vi "LabView Text Okuma.vi"() -> ()   [LabVIEW 2017]
uses:
  <vilib>/Math Plots/3D Math Plots/3D Bar/3D Bar XCtrl/3D Bar.xctl
  <vilib>/Utility/file.llb/Read Delimited Spreadsheet (DBL).vi
  <vilib>/Math Plots/3D Math Plots/3D Bar/3D Bar Datatype/Public/Plot Helper (Matrix).vi
  <vilib>/Math Plots/3D Math Plots/3D Bar/3D Bar Datatype/3D Bar Datatype.lvclass
panel:
  in  "stop 2":bool
  in  "stop":bool
  in  "Gerilme Türünü Seçiniz":string(combo)
  in  "Parça Seçiniz":string(combo)
  in  "Grafik Türünü Seçiniz":string(combo)
  out "?":refnum<class "3D Plot Datatype.lvclass">[](xcontrol)
  out "Array 3":dbl[][](array[numeric])
  out "Min. Yer Değiştirme(mm)":dbl
  out "Max. Yer Değiştirme(mm)":dbl
  out "Max.VonMises Gerilmesi(MPA)":dbl
  out "Min. VonMises Gerilmesi (MPA)":dbl
  in  "Gerilme Türünü Seçiniz":string(combo)
  in  "Ugulanacak Kuvvet Seçiniz (N)":string(combo)
  in  "Parça Seçiniz":string(combo)
  out "Sonuçlar":dbl[][](array[numeric])
  in  "Çıkış":bool
  in  "Oku":bool
  in  "Analiz Yapmak İstedeğiniz Parçanın Veri Dosyasını Açınız!":path
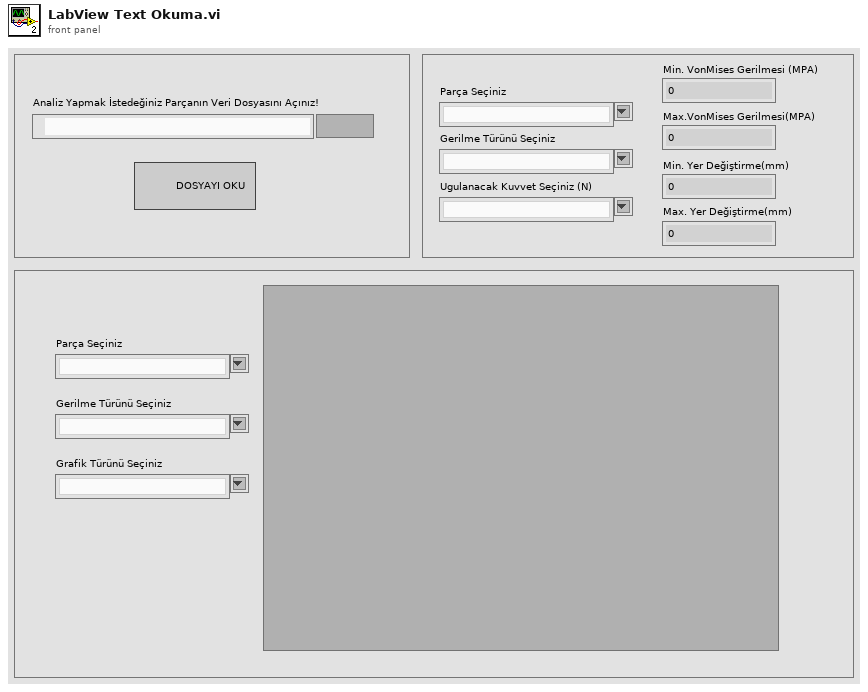
[diagram p1: front panel]
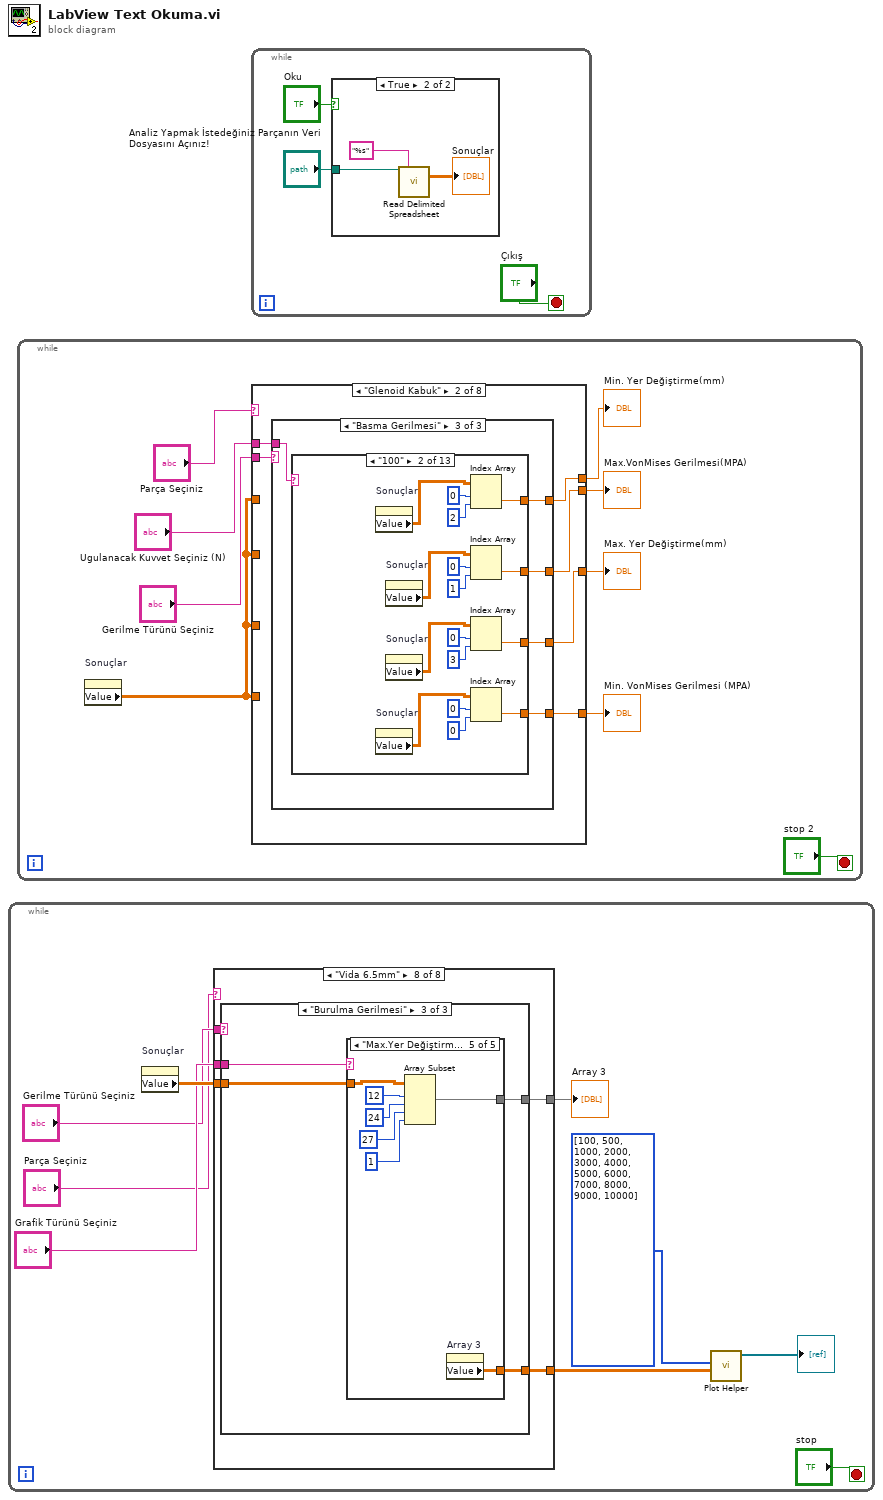
[diagram p0: block diagram]
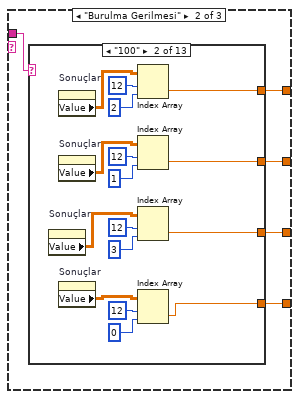
[diagram p4: hidden frame]
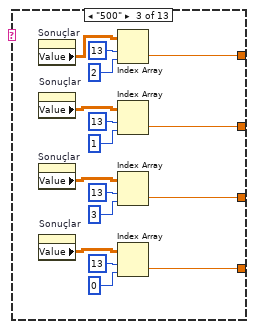
[diagram p6: hidden frame]
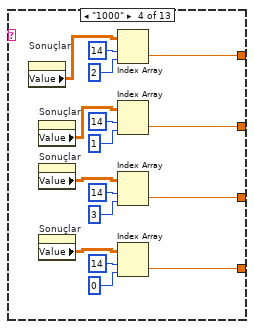
[diagram p7: hidden frame]
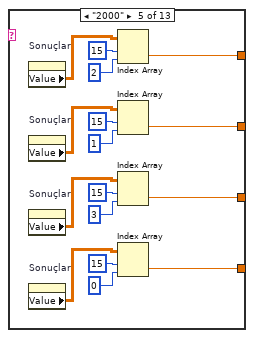
[diagram p8: hidden frame]
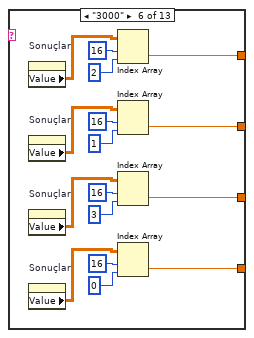
[diagram p9: hidden frame]
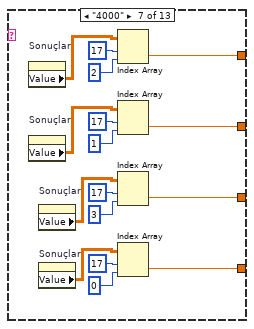
[diagram p10: hidden frame]
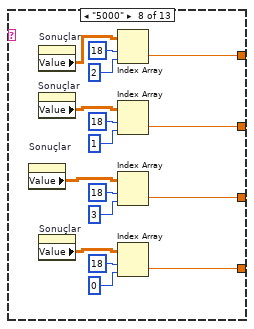
[diagram p11: hidden frame]
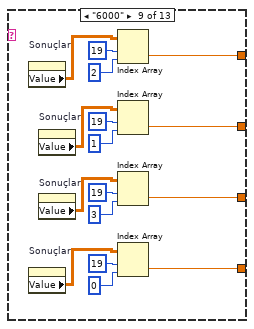
[diagram p12: hidden frame]
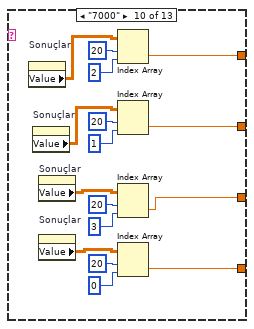
[diagram p13: hidden frame]
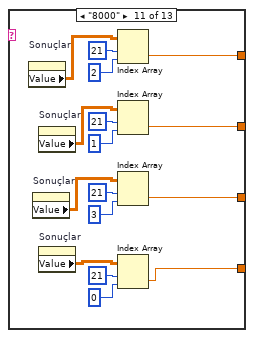
[diagram p14: hidden frame]
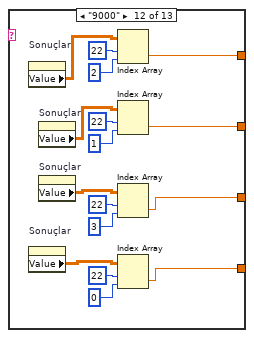
[diagram p15: hidden frame]
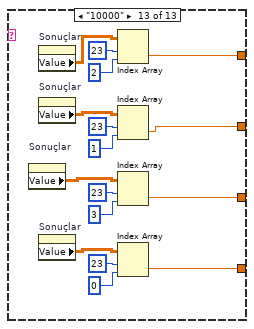
[diagram p16: hidden frame]
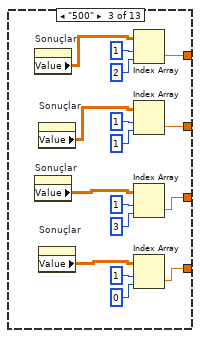
[diagram p18: hidden frame]
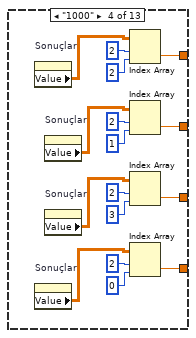
[diagram p19: hidden frame]
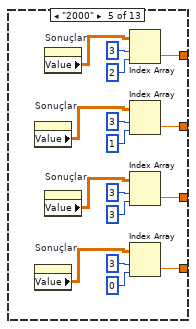
[diagram p20: hidden frame]
diagram:
  n1 = while {
    stop <- "stop" stop-if-true
    n2 = property on="Sonuçlar" class="Arr (strict)"() -> ("Value"=w8:dbl[][])  [unwired: 2 in, 2 out]
    n3 = case shown="\"Vida 6.5mm\"" "Parça Seçiniz" {
      tunnel: w8 -> [_ w14 w83 w152 w220 w290 w359 w428]
      tunnel: "Grafik Türünü Seçiniz" -> [_ w13 w80 w149 w218 w287 w356 w426]
      tunnel: [_ w10 w82 w151 w219 w289 w358 w427] -> w2
      tunnel: [_ w11 w81 w150 w221 w288 w357 w424] -> w6
      tunnel: "Gerilme Türünü Seçiniz" -> [_ w12 w79 w148 w217 w286 w355 w425]
      frame "False", Default {
      }
      frame "Glenoid Kabuk" {
        n4 = case shown="\"Burulma Gerilmesi\"" w12 {
          tunnel: w14 -> [_ w17 w49]
          tunnel: [_ w15 w48] -> w10
          tunnel: [_ w18 w47] -> w11
          tunnel: w13 -> [_ w16 w50]
          frame "False", Default {
          }
          frame "Basma Gerilmesi" {
            n5 = case shown="\"Max.Yer Değiştirme\"" w16 {
              tunnel: w17 -> [_ w20 w28 w35 w43]
              tunnel: [_ w21 w27 w36 w42] -> w15
              tunnel: [_ w19 w26 w33 w40] -> w18
              frame "False", Default {
              }
              frame "Min.VonMises" {
                n6 = Array Subset(array=w20, index (row)=0 ("index"), length (row)=12 ("length"), index (col)=0 ("index"), length (col)=1 ("length")) -> (w21:dbl[][])
                n7 = property on="Array 3" class="Arr (strict)"() -> ("Value"=w19:dbl[][])  [unwired: 2 in, 2 out]
              }
              frame "Max.VonMises" {
                n8 = Array Subset(array=w28, index (row)=0 ("index"), length (row)=12 ("length"), index (col)=1 ("index"), length (col)=1 ("length")) -> (w27:dbl[][])
                n9 = property on="Array 3" class="Arr (strict)"() -> ("Value"=w26:dbl[][])  [unwired: 2 in, 2 out]
              }
              frame "Min.Yer Değiştirme" {
                n10 = Array Subset(array=w35, index (row)=0 ("index"), length (row)=12 ("length"), index (col)=2 ("index"), length (col)=1 ("length")) -> (w36:dbl[][])
                n11 = property on="Array 3" class="Arr (strict)"() -> ("Value"=w33:dbl[][])  [unwired: 2 in, 2 out]
              }
              frame "Max.Yer Değiştirme" {
                n12 = Array Subset(array=w43, index (row)=0 ("index"), length (row)=12 ("length"), index (col)=3 ("index"), length (col)=1 ("length")) -> (w42:dbl[][])
                n13 = property on="Array 3" class="Arr (strict)"() -> ("Value"=w40:dbl[][])  [unwired: 2 in, 2 out]
              }
            }
          }
          frame "Burulma Gerilmesi" {
            n14 = case shown="\"Max.Yer Değiştirme\"" w50 {
              tunnel: w49 -> [_ w57 w60 w67 w75]
              tunnel: [_ w52 w59 w68 w74] -> w48
              tunnel: [_ w51 w58 w65 w72] -> w47
              frame "False", Default {
              }
              frame "Min.VonMises" {
                n15 = Array Subset(array=w57, index (row)=12 ("index"), length (row)=24 ("length"), index (col)=0 ("index"), length (col)=1 ("length")) -> (w52:dbl[][])
                n16 = property on="Array 3" class="Arr (strict)"() -> ("Value"=w51:dbl[][])  [unwired: 2 in, 2 out]
              }
              frame "Max.VonMises" {
                n17 = Array Subset(array=w60, index (row)=12 ("index"), length (row)=24 ("length"), index (col)=1 ("index"), length (col)=1 ("length")) -> (w59:dbl[][])
                n18 = property on="Array 3" class="Arr (strict)"() -> ("Value"=w58:dbl[][])  [unwired: 2 in, 2 out]
              }
              frame "Min.Yer Değiştirme" {
                n19 = Array Subset(array=w67, index (row)=12 ("index"), length (row)=24 ("length"), index (col)=2 ("index"), length (col)=1 ("length")) -> (w68:dbl[][])
                n20 = property on="Array 3" class="Arr (strict)"() -> ("Value"=w65:dbl[][])  [unwired: 2 in, 2 out]
              }
              frame "Max.Yer Değiştirme" {
                n21 = Array Subset(array=w75, index (row)=12 ("index"), length (row)=24 ("length"), index (col)=3 ("index"), length (col)=1 ("length")) -> (w74:dbl[][])
                n22 = property on="Array 3" class="Arr (strict)"() -> ("Value"=w72:dbl[][])  [unwired: 2 in, 2 out]
              }
            }
          }
        }
      }
      frame "Glenoid Yuva" {
        n23 = case shown="\"Burulma Gerilmesi\"" w79 {
          tunnel: w83 -> [_ w86 w118]
          tunnel: [_ w85 w117] -> w82
          tunnel: [_ w87 w116] -> w81
          tunnel: w80 -> [_ w84 w119]
          frame "False", Default {
          }
          frame "Basma Gerilmesi" {
            n24 = case shown="\"Max.Yer Değiştirme\"" w84 {
              tunnel: w86 -> [_ w89 w97 w104 w112]
              tunnel: [_ w90 w96 w105 w111] -> w85
              tunnel: [_ w88 w95 w102 w109] -> w87
              frame "False", Default {
              }
              frame "Min.VonMises" {
                n25 = Array Subset(array=w89, index (row)=0 ("index"), length (row)=12 ("length"), index (col)=4 ("index"), length (col)=1 ("length")) -> (w90:dbl[][])
                n26 = property on="Array 3" class="Arr (strict)"() -> ("Value"=w88:dbl[][])  [unwired: 2 in, 2 out]
              }
              frame "Max.VonMises" {
                n27 = Array Subset(array=w97, index (row)=0 ("index"), length (row)=12 ("length"), index (col)=5 ("index"), length (col)=1 ("length")) -> (w96:dbl[][])
                n28 = property on="Array 3" class="Arr (strict)"() -> ("Value"=w95:dbl[][])  [unwired: 2 in, 2 out]
              }
              frame "Min.Yer Değiştirme" {
                n29 = Array Subset(array=w104, index (row)=0 ("index"), length (row)=12 ("length"), index (col)=6 ("index"), length (col)=1 ("length")) -> (w105:dbl[][])
                n30 = property on="Array 3" class="Arr (strict)"() -> ("Value"=w102:dbl[][])  [unwired: 2 in, 2 out]
              }
              frame "Max.Yer Değiştirme" {
                n31 = Array Subset(array=w112, index (row)=0 ("index"), length (row)=12 ("length"), index (col)=7 ("index"), length (col)=1 ("length")) -> (w111:dbl[][])
                n32 = property on="Array 3" class="Arr (strict)"() -> ("Value"=w109:dbl[][])  [unwired: 2 in, 2 out]
              }
            }
          }
          frame "Burulma Gerilmesi" {
            n33 = case shown="\"Max.Yer Değiştirme\"" w119 {
              tunnel: w118 -> [_ w126 w129 w136 w144]
              tunnel: [_ w121 w128 w137 w143] -> w117
              tunnel: [_ w120 w127 w134 w141] -> w116
              frame "False", Default {
              }
              frame "Min.VonMises" {
                n34 = Array Subset(array=w126, index (row)=12 ("index"), length (row)=24 ("length"), index (col)=4 ("index"), length (col)=1 ("length")) -> (w121:dbl[][])
                n35 = property on="Array 3" class="Arr (strict)"() -> ("Value"=w120:dbl[][])  [unwired: 2 in, 2 out]
              }
              frame "Max.VonMises" {
                n36 = Array Subset(array=w129, index (row)=12 ("index"), length (row)=24 ("length"), index (col)=5 ("index"), length (col)=1 ("length")) -> (w128:dbl[][])
                n37 = property on="Array 3" class="Arr (strict)"() -> ("Value"=w127:dbl[][])  [unwired: 2 in, 2 out]
              }
              frame "Min.Yer Değiştirme" {
                n38 = Array Subset(array=w136, index (row)=12 ("index"), length (row)=24 ("length"), index (col)=6 ("index"), length (col)=1 ("length")) -> (w137:dbl[][])
                n39 = property on="Array 3" class="Arr (strict)"() -> ("Value"=w134:dbl[][])  [unwired: 2 in, 2 out]
              }
              frame "Max.Yer Değiştirme" {
                n40 = Array Subset(array=w144, index (row)=12 ("index"), length (row)=24 ("length"), index (col)=7 ("index"), length (col)=1 ("length")) -> (w143:dbl[][])
                n41 = property on="Array 3" class="Arr (strict)"() -> ("Value"=w141:dbl[][])  [unwired: 2 in, 2 out]
              }
            }
          }
        }
      }
      frame "BüyükKafa" {
        n42 = case shown="\"Burulma Gerilmesi\"" w148 {
          tunnel: w152 -> [_ w155 w187]
          tunnel: [_ w154 w186] -> w151
          tunnel: [_ w156 w185] -> w150
          tunnel: w149 -> [_ w153 w188]
          frame "False", Default {
          }
          frame "Basma Gerilmesi" {
            n43 = case shown="\"Min.VonMises\"" w153 {
              tunnel: w155 -> [_ w158 w166 w173 w181]
              tunnel: [_ w159 w165 w174 w180] -> w154
              tunnel: [_ w157 w164 w171 w178] -> w156
              frame "False", Default {
              }
              frame "Min.VonMises" {
                n44 = Array Subset(array=w158, index (row)=0 ("index"), length (row)=12 ("length"), index (col)=8 ("index"), length (col)=1 ("length")) -> (w159:dbl[][])
                n45 = property on="Array 3" class="Arr (strict)"() -> ("Value"=w157:dbl[][])  [unwired: 2 in, 2 out]
              }
              frame "Max.VonMises" {
                n46 = Array Subset(array=w166, index (row)=0 ("index"), length (row)=12 ("length"), index (col)=9 ("index"), length (col)=1 ("length")) -> (w165:dbl[][])
                n47 = property on="Array 3" class="Arr (strict)"() -> ("Value"=w164:dbl[][])  [unwired: 2 in, 2 out]
              }
              frame "Min.Yer Değiştirme" {
                n48 = Array Subset(array=w173, index (row)=0 ("index"), length (row)=12 ("length"), index (col)=10 ("index"), length (col)=1 ("length")) -> (w174:dbl[][])
                n49 = property on="Array 3" class="Arr (strict)"() -> ("Value"=w171:dbl[][])  [unwired: 2 in, 2 out]
              }
              frame "Max.Yer Değiştirme" {
                n50 = Array Subset(array=w181, index (row)=0 ("index"), length (row)=12 ("length"), index (col)=11 ("index"), length (col)=1 ("length")) -> (w180:dbl[][])
                n51 = property on="Array 3" class="Arr (strict)"() -> ("Value"=w178:dbl[][])  [unwired: 2 in, 2 out]
              }
            }
          }
          frame "Burulma Gerilmesi" {
            n52 = case shown="\"Max.Yer Değiştirme\"" w188 {
              tunnel: w187 -> [_ w195 w198 w205 w213]
              tunnel: [_ w190 w197 w206 w212] -> w186
              tunnel: [_ w189 w196 w203 w210] -> w185
              frame "False", Default {
              }
              frame "Min.VonMises" {
                n53 = Array Subset(array=w195, index (row)=12 ("index"), length (row)=24 ("length"), index (col)=8 ("index"), length (col)=1 ("length")) -> (w190:dbl[][])
                n54 = property on="Array 3" class="Arr (strict)"() -> ("Value"=w189:dbl[][])  [unwired: 2 in, 2 out]
              }
              frame "Max.VonMises" {
                n55 = Array Subset(array=w198, index (row)=12 ("index"), length (row)=24 ("length"), index (col)=9 ("index"), length (col)=1 ("length")) -> (w197:dbl[][])
                n56 = property on="Array 3" class="Arr (strict)"() -> ("Value"=w196:dbl[][])  [unwired: 2 in, 2 out]
              }
              frame "Min.Yer Değiştirme" {
                n57 = Array Subset(array=w205, index (row)=12 ("index"), length (row)=24 ("length"), index (col)=10 ("index"), length (col)=1 ("length")) -> (w206:dbl[][])
                n58 = property on="Array 3" class="Arr (strict)"() -> ("Value"=w203:dbl[][])  [unwired: 2 in, 2 out]
              }
              frame "Max.Yer Değiştirme" {
                n59 = Array Subset(array=w213, index (row)=12 ("index"), length (row)=24 ("length"), index (col)=11 ("index"), length (col)=1 ("length")) -> (w212:dbl[][])
                n60 = property on="Array 3" class="Arr (strict)"() -> ("Value"=w210:dbl[][])  [unwired: 2 in, 2 out]
              }
            }
          }
        }
      }
      frame "KüçükKafa" {
        n61 = case shown="\"Burulma Gerilmesi\"" w217 {
          tunnel: w220 -> [_ w224 w256]
          tunnel: [_ w223 w255] -> w219
          tunnel: [_ w225 w254] -> w221
          tunnel: w218 -> [_ w222 w257]
          frame "False", Default {
          }
          frame "Basma Gerilmesi" {
            n62 = case shown="\"Min.Yer Değiştirme\"" w222 {
              tunnel: w224 -> [_ w232 w235 w242 w250]
              tunnel: [_ w227 w234 w243 w249] -> w223
              tunnel: [_ w226 w233 w240 w247] -> w225
              frame "False", Default {
              }
              frame "Min.VonMises" {
                n63 = Array Subset(array=w232, index (row)=0 ("index"), length (row)=12 ("length"), index (col)=12 ("index"), length (col)=1 ("length")) -> (w227:dbl[][])
                n64 = property on="Array 3" class="Arr (strict)"() -> ("Value"=w226:dbl[][])  [unwired: 2 in, 2 out]
              }
              frame "Max.VonMises" {
                n65 = Array Subset(array=w235, index (row)=0 ("index"), length (row)=12 ("length"), index (col)=13 ("index"), length (col)=1 ("length")) -> (w234:dbl[][])
                n66 = property on="Array 3" class="Arr (strict)"() -> ("Value"=w233:dbl[][])  [unwired: 2 in, 2 out]
              }
              frame "Min.Yer Değiştirme" {
                n67 = Array Subset(array=w242, index (row)=0 ("index"), length (row)=12 ("length"), index (col)=14 ("index"), length (col)=1 ("length")) -> (w243:dbl[][])
                n68 = property on="Array 3" class="Arr (strict)"() -> ("Value"=w240:dbl[][])  [unwired: 2 in, 2 out]
              }
              frame "Max.Yer Değiştirme" {
                n69 = Array Subset(array=w250, index (row)=0 ("index"), length (row)=12 ("length"), index (col)=15 ("index"), length (col)=1 ("length")) -> (w249:dbl[][])
                n70 = property on="Array 3" class="Arr (strict)"() -> ("Value"=w247:dbl[][])  [unwired: 2 in, 2 out]
              }
            }
          }
          frame "Burulma Gerilmesi" {
            n71 = case shown="\"Max.Yer Değiştirme\"" w257 {
              tunnel: w256 -> [_ w264 w267 w274 w282]
              tunnel: [_ w259 w266 w275 w281] -> w255
              tunnel: [_ w258 w265 w272 w279] -> w254
              frame "False", Default {
              }
              frame "Min.VonMises" {
                n72 = Array Subset(array=w264, index (row)=12 ("index"), length (row)=24 ("length"), index (col)=12 ("index"), length (col)=1 ("length")) -> (w259:dbl[][])
                n73 = property on="Array 3" class="Arr (strict)"() -> ("Value"=w258:dbl[][])  [unwired: 2 in, 2 out]
              }
              frame "Max.VonMises" {
                n74 = Array Subset(array=w267, index (row)=12 ("index"), length (row)=24 ("length"), index (col)=13 ("index"), length (col)=1 ("length")) -> (w266:dbl[][])
                n75 = property on="Array 3" class="Arr (strict)"() -> ("Value"=w265:dbl[][])  [unwired: 2 in, 2 out]
              }
              frame "Min.Yer Değiştirme" {
                n76 = Array Subset(array=w274, index (row)=12 ("index"), length (row)=24 ("length"), index (col)=14 ("index"), length (col)=1 ("length")) -> (w275:dbl[][])
                n77 = property on="Array 3" class="Arr (strict)"() -> ("Value"=w272:dbl[][])  [unwired: 2 in, 2 out]
              }
              frame "Max.Yer Değiştirme" {
                n78 = Array Subset(array=w282, index (row)=12 ("index"), length (row)=24 ("length"), index (col)=15 ("index"), length (col)=1 ("length")) -> (w281:dbl[][])
                n79 = property on="Array 3" class="Arr (strict)"() -> ("Value"=w279:dbl[][])  [unwired: 2 in, 2 out]
              }
            }
          }
        }
      }
      frame "Humeral Sap" {
        n80 = case shown="\"Basma Gerilmesi\"" w286 {
          tunnel: w290 -> [_ w294 w325]
          tunnel: [_ w291 w324] -> w289
          tunnel: [_ w293 w323] -> w288
          tunnel: w287 -> [_ w292 w326]
          frame "False", Default {
          }
          frame "Basma Gerilmesi" {
            n81 = case shown="\"Max.Yer Değiştirme\"" w292 {
              tunnel: w294 -> [_ w301 w304 w311 w319]
              tunnel: [_ w296 w303 w312 w318] -> w291
              tunnel: [_ w295 w302 w310 w317] -> w293
              frame "False", Default {
              }
              frame "Min.VonMises" {
                n82 = Array Subset(array=w301, index (row)=0 ("index"), length (row)=12 ("length"), index (col)=16 ("index"), length (col)=1 ("length")) -> (w296:dbl[][])
                n83 = property on="Array 3" class="Arr (strict)"() -> ("Value"=w295:dbl[][])  [unwired: 2 in, 2 out]
              }
              frame "Max.VonMises" {
                n84 = Array Subset(array=w304, index (row)=0 ("index"), length (row)=12 ("length"), index (col)=17 ("index"), length (col)=1 ("length")) -> (w303:dbl[][])
                n85 = property on="Array 3" class="Arr (strict)"() -> ("Value"=w302:dbl[][])  [unwired: 2 in, 2 out]
              }
              frame "Min.Yer Değiştirme" {
                n86 = Array Subset(array=w311, index (row)=0 ("index"), length (row)=12 ("length"), index (col)=18 ("index"), length (col)=1 ("length")) -> (w312:dbl[][])
                n87 = property on="Array 3" class="Arr (strict)"() -> ("Value"=w310:dbl[][])  [unwired: 2 in, 2 out]
              }
              frame "Max.Yer Değiştirme" {
                n88 = Array Subset(array=w319, index (row)=0 ("index"), length (row)=12 ("length"), index (col)=19 ("index"), length (col)=1 ("length")) -> (w318:dbl[][])
                n89 = property on="Array 3" class="Arr (strict)"() -> ("Value"=w317:dbl[][])  [unwired: 2 in, 2 out]
              }
            }
          }
          frame "Burulma Gerilmesi" {
            n90 = case shown="\"Max.Yer Değiştirme\"" w326 {
              tunnel: w325 -> [_ w333 w336 w343 w351]
              tunnel: [_ w328 w335 w344 w350] -> w324
              tunnel: [_ w327 w334 w341 w348] -> w323
              frame "False", Default {
              }
              frame "Min.VonMises" {
                n91 = Array Subset(array=w333, index (row)=12 ("index"), length (row)=24 ("length"), index (col)=16 ("index"), length (col)=1 ("length")) -> (w328:dbl[][])
                n92 = property on="Array 3" class="Arr (strict)"() -> ("Value"=w327:dbl[][])  [unwired: 2 in, 2 out]
              }
              frame "Max.VonMises" {
                n93 = Array Subset(array=w336, index (row)=12 ("index"), length (row)=24 ("length"), index (col)=17 ("index"), length (col)=1 ("length")) -> (w335:dbl[][])
                n94 = property on="Array 3" class="Arr (strict)"() -> ("Value"=w334:dbl[][])  [unwired: 2 in, 2 out]
              }
              frame "Min.Yer Değiştirme" {
                n95 = Array Subset(array=w343, index (row)=12 ("index"), length (row)=24 ("length"), index (col)=18 ("index"), length (col)=1 ("length")) -> (w344:dbl[][])
                n96 = property on="Array 3" class="Arr (strict)"() -> ("Value"=w341:dbl[][])  [unwired: 2 in, 2 out]
              }
              frame "Max.Yer Değiştirme" {
                n97 = Array Subset(array=w351, index (row)=12 ("index"), length (row)=24 ("length"), index (col)=19 ("index"), length (col)=1 ("length")) -> (w350:dbl[][])
                n98 = property on="Array 3" class="Arr (strict)"() -> ("Value"=w348:dbl[][])  [unwired: 2 in, 2 out]
              }
            }
          }
        }
      }
      frame "Vida 4mm" {
        n99 = case shown="\"Burulma Gerilmesi\"" w355 {
          tunnel: w359 -> [_ w362 w394]
          tunnel: [_ w361 w393] -> w358
          tunnel: [_ w363 w392] -> w357
          tunnel: w356 -> [_ w360 w395]
          frame "False", Default {
          }
          frame "Basma Gerilmesi" {
            n100 = case shown="\"False\", Default" w360 {
              tunnel: w362 -> [_ w370 w373 w380 w388]
              tunnel: [_ w365 w372 w381 w387] -> w361
              tunnel: [_ w364 w371 w378 w385] -> w363
              frame "False", Default {
              }
              frame "Min.VonMises" {
                n101 = Array Subset(array=w370, index (row)=0 ("index"), length (row)=12 ("length"), index (col)=20 ("index"), length (col)=1 ("length")) -> (w365:dbl[][])
                n102 = property on="Array 3" class="Arr (strict)"() -> ("Value"=w364:dbl[][])  [unwired: 2 in, 2 out]
              }
              frame "Max.VonMises" {
                n103 = Array Subset(array=w373, index (row)=0 ("index"), length (row)=12 ("length"), index (col)=21 ("index"), length (col)=1 ("length")) -> (w372:dbl[][])
                n104 = property on="Array 3" class="Arr (strict)"() -> ("Value"=w371:dbl[][])  [unwired: 2 in, 2 out]
              }
              frame "Min.Yer Değiştirme" {
                n105 = Array Subset(array=w380, index (row)=0 ("index"), length (row)=12 ("length"), index (col)=22 ("index"), length (col)=1 ("length")) -> (w381:dbl[][])
                n106 = property on="Array 3" class="Arr (strict)"() -> ("Value"=w378:dbl[][])  [unwired: 2 in, 2 out]
              }
              frame "Max.Yer Değiştirme" {
                n107 = Array Subset(array=w388, index (row)=0 ("index"), length (row)=12 ("length"), index (col)=23 ("index"), length (col)=1 ("length")) -> (w387:dbl[][])
                n108 = property on="Array 3" class="Arr (strict)"() -> ("Value"=w385:dbl[][])  [unwired: 2 in, 2 out]
              }
            }
          }
          frame "Burulma Gerilmesi" {
            n109 = case shown="\"False\", Default" w395 {
              tunnel: w394 -> [_ w402 w405 w412 w420]
              tunnel: [_ w397 w404 w413 w419] -> w393
              tunnel: [_ w396 w403 w410 w417] -> w392
              frame "False", Default {
              }
              frame "Min.VonMises" {
                n110 = Array Subset(array=w402, index (row)=12 ("index"), length (row)=24 ("length"), index (col)=20 ("index"), length (col)=1 ("length")) -> (w397:dbl[][])
                n111 = property on="Array 3" class="Arr (strict)"() -> ("Value"=w396:dbl[][])  [unwired: 2 in, 2 out]
              }
              frame "Max.VonMises" {
                n112 = Array Subset(array=w405, index (row)=12 ("index"), length (row)=24 ("length"), index (col)=21 ("index"), length (col)=1 ("length")) -> (w404:dbl[][])
                n113 = property on="Array 3" class="Arr (strict)"() -> ("Value"=w403:dbl[][])  [unwired: 2 in, 2 out]
              }
              frame "Min.Yer Değiştirme" {
                n114 = Array Subset(array=w412, index (row)=12 ("index"), length (row)=24 ("length"), index (col)=22 ("index"), length (col)=1 ("length")) -> (w413:dbl[][])
                n115 = property on="Array 3" class="Arr (strict)"() -> ("Value"=w410:dbl[][])  [unwired: 2 in, 2 out]
              }
              frame "Max.Yer Değiştirme" {
                n116 = Array Subset(array=w420, index (row)=12 ("index"), length (row)=24 ("length"), index (col)=23 ("index"), length (col)=1 ("length")) -> (w419:dbl[][])
                n117 = property on="Array 3" class="Arr (strict)"() -> ("Value"=w417:dbl[][])  [unwired: 2 in, 2 out]
              }
            }
          }
        }
      }
      frame "Vida 6.5mm" {
        n118 = case shown="\"Burulma Gerilmesi\"" w425 {
          tunnel: w428 -> [_ w431 w463]
          tunnel: [_ w430 w462] -> w427
          tunnel: [_ w432 w461] -> w424
          tunnel: w426 -> [_ w429 w464]
          frame "False", Default {
          }
          frame "Basma Gerilmesi" {
            n119 = case shown="\"Min.VonMises\"" w429 {
              tunnel: w431 -> [_ w434 w442 w449 w457]
              tunnel: [_ w435 w441 w450 w456] -> w430
              tunnel: [_ w433 w440 w447 w454] -> w432
              frame "False", Default {
              }
              frame "Min.VonMises" {
                n120 = Array Subset(array=w434, index (row)=0 ("index"), length (row)=12 ("length"), index (col)=24 ("index"), length (col)=1 ("length")) -> (w435:dbl[][])
                n121 = property on="Array 3" class="Arr (strict)"() -> ("Value"=w433:dbl[][])  [unwired: 2 in, 2 out]
              }
              frame "Max.VonMises" {
                n122 = Array Subset(array=w442, index (row)=0 ("index"), length (row)=12 ("length"), index (col)=25 ("index"), length (col)=1 ("length")) -> (w441:dbl[][])
                n123 = property on="Array 3" class="Arr (strict)"() -> ("Value"=w440:dbl[][])  [unwired: 2 in, 2 out]
              }
              frame "Min.Yer Değiştirme" {
                n124 = Array Subset(array=w449, index (row)=0 ("index"), length (row)=12 ("length"), index (col)=26 ("index"), length (col)=1 ("length")) -> (w450:dbl[][])
                n125 = property on="Array 3" class="Arr (strict)"() -> ("Value"=w447:dbl[][])  [unwired: 2 in, 2 out]
              }
              frame "Max.Yer Değiştirme" {
                n126 = Array Subset(array=w457, index (row)=0 ("index"), length (row)=12 ("length"), index (col)=27 ("index"), length (col)=1 ("length")) -> (w456:dbl[][])
                n127 = property on="Array 3" class="Arr (strict)"() -> ("Value"=w454:dbl[][])  [unwired: 2 in, 2 out]
              }
            }
          }
          frame "Burulma Gerilmesi" {
            n128 = case shown="\"Max.Yer Değiştirme\"" w464 {
              tunnel: w463 -> [_ w471 w474 w481 w489]
              tunnel: [_ w466 w473 w482 w488] -> w462
              tunnel: [_ w465 w472 w479 w486] -> w461
              frame "False", Default {
              }
              frame "Min.VonMises" {
                n129 = Array Subset(array=w471, index (row)=12 ("index"), length (row)=24 ("length"), index (col)=24 ("index"), length (col)=1 ("length")) -> (w466:dbl[][])
                n130 = property on="Array 3" class="Arr (strict)"() -> ("Value"=w465:dbl[][])  [unwired: 2 in, 2 out]
              }
              frame "Max.VonMises" {
                n131 = Array Subset(array=w474, index (row)=12 ("index"), length (row)=24 ("length"), index (col)=24 ("index"), length (col)=1 ("length")) -> (w473:dbl[][])
                n132 = property on="Array 3" class="Arr (strict)"() -> ("Value"=w472:dbl[][])  [unwired: 2 in, 2 out]
              }
              frame "Min.Yer Değiştirme" {
                n133 = Array Subset(array=w481, index (row)=12 ("index"), length (row)=24 ("length"), index (col)=26 ("index"), length (col)=1 ("length")) -> (w482:dbl[][])
                n134 = property on="Array 3" class="Arr (strict)"() -> ("Value"=w479:dbl[][])  [unwired: 2 in, 2 out]
              }
              frame "Max.Yer Değiştirme" {
                n135 = Array Subset(array=w489, index (row)=12 ("index"), length (row)=24 ("length"), index (col)=27 ("index"), length (col)=1 ("length")) -> (w488:dbl[][])
                n136 = property on="Array 3" class="Arr (strict)"() -> ("Value"=w486:dbl[][])  [unwired: 2 in, 2 out]
              }
            }
          }
        }
      }
    }
    "Array 3" <- w2
    n137 = call-poly <vilib>:"Plot Helper.vi"("z matrix"=w6, "y vector"=i32[] [100, 500, 1000, 2000, 3000, 4000, 5000, 6000, 7000, 8000, 9000, 10000]) -> ("3D Plot lvclass Array out"=→"?":refnum<class "3D Plot Datatype.lvclass">[])  [unwired: 1 in, 8 out]
  }
  n138 = while {
    stop <- "stop 2" stop-if-true
    n139 = property on="Sonuçlar" class="Arr (strict)"() -> ("Value"=w494:dbl[][])  [unwired: 2 in, 2 out]
    n140 = case shown="\"Glenoid Kabuk\"" "Parça Seçiniz" {
      tunnel: "Gerilme Türünü Seçiniz" -> [_ w506 w906 w1306 w1706 w2111 w2522 w2934]
      tunnel: "Ugulanacak Kuvvet Seçiniz (N)" -> [_ w507 w907 w1307 w1707 w2110 w2523 w2935]
      tunnel: [_ w505 w903 w1304 w1705 w2103 w2514 w2926] -> w498
      tunnel: [_ w504 w904 w1303 w1703 w2106 w2516 w2928] -> w497
      tunnel: [_ w503 w905 w1302 w1702 w2108 w2517 w2929] -> w495
      tunnel: [_ w502 w902 w1305 w1704 w2102 w2515 w2927] -> w496
      tunnel: w494 -> [_ _ _ _ _ w2109 w2519 w2931]
      tunnel: w494 -> [_ _ _ _ _ w2107 w2521 w2933]
      tunnel: w494 -> [_ _ _ _ _ w2105 w2520 w2932]
      tunnel: w494 -> [_ _ _ _ _ w2104 w2518 w2930]
      frame "False", Default {
      }
      frame "Glenoid Kabuk" {
        n141 = case shown="\"Basma Gerilmesi\"" w506 {
          tunnel: w507 -> [_ w512 w709]
          tunnel: [_ w509 w708] -> w505
          tunnel: [_ w511 w707] -> w504
          tunnel: [_ w510 w706] -> w503
          tunnel: [_ w508 w705] -> w502
          frame "False", Default {
          }
          frame "Burulma Gerilmesi" {
            n142 = case shown="\"100\"" w512 {
              tunnel: [_ w514 w531 w546 w563 w579 w595 w612 w627 w642 w659 w674 w691] -> w511
              tunnel: [_ w513 w532 w545 w564 w580 w596 w611 w628 w641 w660 w673 w692] -> w510
              tunnel: [_ w515 w530 w547 w562 w578 w594 w610 w626 w643 w658 w675 w690] -> w509
              tunnel: [_ w516 w529 w548 w561 w577 w593 w609 w625 w644 w657 w676 w689] -> w508
              frame "False", Default {
              }
              frame "100" {
                n143 = property on="Sonuçlar" class="Arr (strict)"() -> ("Value"=w521:dbl[][])  [unwired: 2 in, 2 out]
                n144 = property on="Sonuçlar" class="Arr (strict)"() -> ("Value"=w524:dbl[][])  [unwired: 2 in, 2 out]
                n145 = property on="Sonuçlar" class="Arr (strict)"() -> ("Value"=w523:dbl[][])  [unwired: 2 in, 2 out]
                n146 = property on="Sonuçlar" class="Arr (strict)"() -> ("Value"=w522:dbl[][])  [unwired: 2 in, 2 out]
                n147 = Index Array(array=w524, index (row)=12 ("index"), index (col)=2 ("disabled index (col)")) -> (element=w513:dbl)
                n148 = Index Array(array=w523, index (row)=12 ("index"), index (col)=1 ("disabled index (col)")) -> (element=w514:dbl)
                n149 = Index Array(array=w521, index (row)=12 ("index"), index (col)=3 ("disabled index (col)")) -> (element=w516:dbl)
                n150 = Index Array(array=w522, index (row)=12 ("index"), index (col)=0 ("disabled index (col)")) -> (element=w515:dbl)
              }
              frame "500" {
                n151 = property on="Sonuçlar" class="Arr (strict)"() -> ("Value"=w534:dbl[][])  [unwired: 2 in, 2 out]
                n152 = property on="Sonuçlar" class="Arr (strict)"() -> ("Value"=w536:dbl[][])  [unwired: 2 in, 2 out]
                n153 = property on="Sonuçlar" class="Arr (strict)"() -> ("Value"=w540:dbl[][])  [unwired: 2 in, 2 out]
                n154 = property on="Sonuçlar" class="Arr (strict)"() -> ("Value"=w538:dbl[][])  [unwired: 2 in, 2 out]
                n155 = Index Array(array=w534, index (row)=13 ("index"), index (col)=2 ("disabled index (col)")) -> (element=w532:dbl)
                n156 = Index Array(array=w536, index (row)=13 ("index"), index (col)=1 ("disabled index (col)")) -> (element=w531:dbl)
                n157 = Index Array(array=w540, index (row)=13 ("index"), index (col)=3 ("disabled index (col)")) -> (element=w529:dbl)
                n158 = Index Array(array=w538, index (row)=13 ("index"), index (col)=0 ("disabled index (col)")) -> (element=w530:dbl)
              }
              frame "1000" {
                n159 = property on="Sonuçlar" class="Arr (strict)"() -> ("Value"=w556:dbl[][])  [unwired: 2 in, 2 out]
                n160 = property on="Sonuçlar" class="Arr (strict)"() -> ("Value"=w555:dbl[][])  [unwired: 2 in, 2 out]
                n161 = property on="Sonuçlar" class="Arr (strict)"() -> ("Value"=w553:dbl[][])  [unwired: 2 in, 2 out]
                n162 = property on="Sonuçlar" class="Arr (strict)"() -> ("Value"=w554:dbl[][])  [unwired: 2 in, 2 out]
                n163 = Index Array(array=w556, index (row)=14 ("index"), index (col)=2 ("disabled index (col)")) -> (element=w545:dbl)
                n164 = Index Array(array=w555, index (row)=14 ("index"), index (col)=1 ("disabled index (col)")) -> (element=w546:dbl)
                n165 = Index Array(array=w553, index (row)=14 ("index"), index (col)=3 ("disabled index (col)")) -> (element=w548:dbl)
                n166 = Index Array(array=w554, index (row)=14 ("index"), index (col)=0 ("disabled index (col)")) -> (element=w547:dbl)
              }
              frame "2000" {
                n167 = property on="Sonuçlar" class="Arr (strict)"() -> ("Value"=w572:dbl[][])  [unwired: 2 in, 2 out]
                n168 = property on="Sonuçlar" class="Arr (strict)"() -> ("Value"=w571:dbl[][])  [unwired: 2 in, 2 out]
                n169 = property on="Sonuçlar" class="Arr (strict)"() -> ("Value"=w569:dbl[][])  [unwired: 2 in, 2 out]
                n170 = property on="Sonuçlar" class="Arr (strict)"() -> ("Value"=w570:dbl[][])  [unwired: 2 in, 2 out]
                n171 = Index Array(array=w572, index (row)=15 ("index"), index (col)=2 ("disabled index (col)")) -> (element=w564:dbl)
                n172 = Index Array(array=w571, index (row)=15 ("index"), index (col)=1 ("disabled index (col)")) -> (element=w563:dbl)
                n173 = Index Array(array=w569, index (row)=15 ("index"), index (col)=3 ("disabled index (col)")) -> (element=w561:dbl)
                n174 = Index Array(array=w570, index (row)=15 ("index"), index (col)=0 ("disabled index (col)")) -> (element=w562:dbl)
              }
              frame "3000" {
                n175 = property on="Sonuçlar" class="Arr (strict)"() -> ("Value"=w582:dbl[][])  [unwired: 2 in, 2 out]
                n176 = property on="Sonuçlar" class="Arr (strict)"() -> ("Value"=w584:dbl[][])  [unwired: 2 in, 2 out]
                n177 = property on="Sonuçlar" class="Arr (strict)"() -> ("Value"=w588:dbl[][])  [unwired: 2 in, 2 out]
                n178 = property on="Sonuçlar" class="Arr (strict)"() -> ("Value"=w586:dbl[][])  [unwired: 2 in, 2 out]
                n179 = Index Array(array=w582, index (row)=16 ("index"), index (col)=2 ("disabled index (col)")) -> (element=w580:dbl)
                n180 = Index Array(array=w584, index (row)=16 ("index"), index (col)=1 ("disabled index (col)")) -> (element=w579:dbl)
                n181 = Index Array(array=w588, index (row)=16 ("index"), index (col)=3 ("disabled index (col)")) -> (element=w577:dbl)
                n182 = Index Array(array=w586, index (row)=16 ("index"), index (col)=0 ("disabled index (col)")) -> (element=w578:dbl)
              }
              frame "4000" {
                n183 = property on="Sonuçlar" class="Arr (strict)"() -> ("Value"=w601:dbl[][])  [unwired: 2 in, 2 out]
                n184 = property on="Sonuçlar" class="Arr (strict)"() -> ("Value"=w602:dbl[][])  [unwired: 2 in, 2 out]
                n185 = property on="Sonuçlar" class="Arr (strict)"() -> ("Value"=w604:dbl[][])  [unwired: 2 in, 2 out]
                n186 = property on="Sonuçlar" class="Arr (strict)"() -> ("Value"=w603:dbl[][])  [unwired: 2 in, 2 out]
                n187 = Index Array(array=w601, index (row)=17 ("index"), index (col)=2 ("disabled index (col)")) -> (element=w596:dbl)
                n188 = Index Array(array=w602, index (row)=17 ("index"), index (col)=1 ("disabled index (col)")) -> (element=w595:dbl)
                n189 = Index Array(array=w604, index (row)=17 ("index"), index (col)=3 ("disabled index (col)")) -> (element=w593:dbl)
                n190 = Index Array(array=w603, index (row)=17 ("index"), index (col)=0 ("disabled index (col)")) -> (element=w594:dbl)
              }
              frame "5000" {
                n191 = property on="Sonuçlar" class="Arr (strict)"() -> ("Value"=w617:dbl[][])  [unwired: 2 in, 2 out]
                n192 = property on="Sonuçlar" class="Arr (strict)"() -> ("Value"=w619:dbl[][])  [unwired: 2 in, 2 out]
                n193 = property on="Sonuçlar" class="Arr (strict)"() -> ("Value"=w620:dbl[][])  [unwired: 2 in, 2 out]
                n194 = property on="Sonuçlar" class="Arr (strict)"() -> ("Value"=w618:dbl[][])  [unwired: 2 in, 2 out]
                n195 = Index Array(array=w619, index (row)=18 ("index"), index (col)=2 ("disabled index (col)")) -> (element=w611:dbl)
                n196 = Index Array(array=w620, index (row)=18 ("index"), index (col)=1 ("disabled index (col)")) -> (element=w612:dbl)
                n197 = Index Array(array=w617, index (row)=18 ("index"), index (col)=3 ("disabled index (col)")) -> (element=w609:dbl)
                n198 = Index Array(array=w618, index (row)=18 ("index"), index (col)=0 ("disabled index (col)")) -> (element=w610:dbl)
              }
              frame "6000" {
                n199 = property on="Sonuçlar" class="Arr (strict)"() -> ("Value"=w633:dbl[][])  [unwired: 2 in, 2 out]
                n200 = property on="Sonuçlar" class="Arr (strict)"() -> ("Value"=w635:dbl[][])  [unwired: 2 in, 2 out]
                n201 = property on="Sonuçlar" class="Arr (strict)"() -> ("Value"=w634:dbl[][])  [unwired: 2 in, 2 out]
                n202 = property on="Sonuçlar" class="Arr (strict)"() -> ("Value"=w636:dbl[][])  [unwired: 2 in, 2 out]
                n203 = Index Array(array=w633, index (row)=19 ("index"), index (col)=2 ("disabled index (col)")) -> (element=w628:dbl)
                n204 = Index Array(array=w634, index (row)=19 ("index"), index (col)=1 ("disabled index (col)")) -> (element=w627:dbl)
                n205 = Index Array(array=w636, index (row)=19 ("index"), index (col)=3 ("disabled index (col)")) -> (element=w625:dbl)
                n206 = Index Array(array=w635, index (row)=19 ("index"), index (col)=0 ("disabled index (col)")) -> (element=w626:dbl)
              }
              frame "7000" {
                n207 = property on="Sonuçlar" class="Arr (strict)"() -> ("Value"=w649:dbl[][])  [unwired: 2 in, 2 out]
                n208 = property on="Sonuçlar" class="Arr (strict)"() -> ("Value"=w650:dbl[][])  [unwired: 2 in, 2 out]
                n209 = property on="Sonuçlar" class="Arr (strict)"() -> ("Value"=w652:dbl[][])  [unwired: 2 in, 2 out]
                n210 = property on="Sonuçlar" class="Arr (strict)"() -> ("Value"=w651:dbl[][])  [unwired: 2 in, 2 out]
                n211 = Index Array(array=w649, index (row)=20 ("index"), index (col)=2 ("disabled index (col)")) -> (element=w641:dbl)
                n212 = Index Array(array=w650, index (row)=20 ("index"), index (col)=1 ("disabled index (col)")) -> (element=w642:dbl)
                n213 = Index Array(array=w652, index (row)=20 ("index"), index (col)=3 ("disabled index (col)")) -> (element=w644:dbl)
                n214 = Index Array(array=w651, index (row)=20 ("index"), index (col)=0 ("disabled index (col)")) -> (element=w643:dbl)
              }
              frame "8000" {
                n215 = property on="Sonuçlar" class="Arr (strict)"() -> ("Value"=w665:dbl[][])  [unwired: 2 in, 2 out]
                n216 = property on="Sonuçlar" class="Arr (strict)"() -> ("Value"=w668:dbl[][])  [unwired: 2 in, 2 out]
                n217 = property on="Sonuçlar" class="Arr (strict)"() -> ("Value"=w666:dbl[][])  [unwired: 2 in, 2 out]
                n218 = property on="Sonuçlar" class="Arr (strict)"() -> ("Value"=w667:dbl[][])  [unwired: 2 in, 2 out]
                n219 = Index Array(array=w665, index (row)=21 ("index"), index (col)=2 ("disabled index (col)")) -> (element=w660:dbl)
                n220 = Index Array(array=w666, index (row)=21 ("index"), index (col)=1 ("disabled index (col)")) -> (element=w659:dbl)
                n221 = Index Array(array=w668, index (row)=21 ("index"), index (col)=3 ("disabled index (col)")) -> (element=w657:dbl)
                n222 = Index Array(array=w667, index (row)=21 ("index"), index (col)=0 ("disabled index (col)")) -> (element=w658:dbl)
              }
              frame "9000" {
                n223 = property on="Sonuçlar" class="Arr (strict)"() -> ("Value"=w681:dbl[][])  [unwired: 2 in, 2 out]
                n224 = property on="Sonuçlar" class="Arr (strict)"() -> ("Value"=w683:dbl[][])  [unwired: 2 in, 2 out]
                n225 = property on="Sonuçlar" class="Arr (strict)"() -> ("Value"=w682:dbl[][])  [unwired: 2 in, 2 out]
                n226 = property on="Sonuçlar" class="Arr (strict)"() -> ("Value"=w684:dbl[][])  [unwired: 2 in, 2 out]
                n227 = Index Array(array=w681, index (row)=22 ("index"), index (col)=2 ("disabled index (col)")) -> (element=w673:dbl)
                n228 = Index Array(array=w682, index (row)=22 ("index"), index (col)=1 ("disabled index (col)")) -> (element=w674:dbl)
                n229 = Index Array(array=w684, index (row)=22 ("index"), index (col)=3 ("disabled index (col)")) -> (element=w676:dbl)
                n230 = Index Array(array=w683, index (row)=22 ("index"), index (col)=0 ("disabled index (col)")) -> (element=w675:dbl)
              }
              frame "10000" {
                n231 = property on="Sonuçlar" class="Arr (strict)"() -> ("Value"=w697:dbl[][])  [unwired: 2 in, 2 out]
                n232 = property on="Sonuçlar" class="Arr (strict)"() -> ("Value"=w700:dbl[][])  [unwired: 2 in, 2 out]
                n233 = property on="Sonuçlar" class="Arr (strict)"() -> ("Value"=w699:dbl[][])  [unwired: 2 in, 2 out]
                n234 = property on="Sonuçlar" class="Arr (strict)"() -> ("Value"=w698:dbl[][])  [unwired: 2 in, 2 out]
                n235 = Index Array(array=w700, index (row)=23 ("index"), index (col)=2 ("disabled index (col)")) -> (element=w692:dbl)
                n236 = Index Array(array=w699, index (row)=23 ("index"), index (col)=1 ("disabled index (col)")) -> (element=w691:dbl)
                n237 = Index Array(array=w697, index (row)=23 ("index"), index (col)=3 ("disabled index (col)")) -> (element=w689:dbl)
                n238 = Index Array(array=w698, index (row)=23 ("index"), index (col)=0 ("disabled index (col)")) -> (element=w690:dbl)
              }
            }
          }
          frame "Basma Gerilmesi" {
            n239 = case shown="\"100\"" w709 {
              tunnel: [_ w713 w738 w745 w761 w777 w793 w809 w826 w845 w854 w873 w886] -> w708
              tunnel: [_ w710 w734 w742 w758 w774 w790 w806 w822 w842 w856 w870 w889] -> w707
              tunnel: [_ w712 w727 w744 w760 w776 w792 w808 w827 w844 w857 w872 w887] -> w706
              tunnel: [_ w711 w726 w743 w759 w775 w791 w807 w824 w843 w855 w871 w888] -> w705
              frame "False", Default {
              }
              frame "100" {
                n240 = property on="Sonuçlar" class="Arr (strict)"() -> ("Value"=w723:dbl[][])  [unwired: 2 in, 2 out]
                n241 = property on="Sonuçlar" class="Arr (strict)"() -> ("Value"=w722:dbl[][])  [unwired: 2 in, 2 out]
                n242 = property on="Sonuçlar" class="Arr (strict)"() -> ("Value"=w725:dbl[][])  [unwired: 2 in, 2 out]
                n243 = property on="Sonuçlar" class="Arr (strict)"() -> ("Value"=w724:dbl[][])  [unwired: 2 in, 2 out]
                n244 = Index Array(array=w723, index (row)=0, index (col)=2 ("disabled index (col)")) -> (element=w712:dbl)
                n245 = Index Array(array=w725, index (row)=0, index (col)=1 ("disabled index (col)")) -> (element=w710:dbl)
                n246 = Index Array(array=w724, index (row)=0, index (col)=3 ("disabled index (col)")) -> (element=w711:dbl)
                n247 = Index Array(array=w722, index (row)=0, index (col)=0 ("disabled index (col)")) -> (element=w713:dbl)
              }
              frame "500" {
                n248 = property on="Sonuçlar" class="Arr (strict)"() -> ("Value"=w733:dbl[][])  [unwired: 2 in, 2 out]
                n249 = property on="Sonuçlar" class="Arr (strict)"() -> ("Value"=w730:dbl[][])  [unwired: 2 in, 2 out]
                n250 = property on="Sonuçlar" class="Arr (strict)"() -> ("Value"=w737:dbl[][])  [unwired: 2 in, 2 out]
                n251 = property on="Sonuçlar" class="Arr (strict)"() -> ("Value"=w741:dbl[][])  [unwired: 2 in, 2 out]
                n252 = Index Array(array=w733, index (row)=1, index (col)=2 ("disabled index (col)")) -> (element=w727:dbl)
                n253 = Index Array(array=w737, index (row)=1, index (col)=1 ("disabled index (col)")) -> (element=w734:dbl)
                n254 = Index Array(array=w730, index (row)=1, index (col)=3 ("disabled index (col)")) -> (element=w726:dbl)
                n255 = Index Array(array=w741, index (row)=1, index (col)=0 ("disabled index (col)")) -> (element=w738:dbl)
              }
              frame "1000" {
                n256 = property on="Sonuçlar" class="Arr (strict)"() -> ("Value"=w755:dbl[][])  [unwired: 2 in, 2 out]
                n257 = property on="Sonuçlar" class="Arr (strict)"() -> ("Value"=w754:dbl[][])  [unwired: 2 in, 2 out]
                n258 = property on="Sonuçlar" class="Arr (strict)"() -> ("Value"=w757:dbl[][])  [unwired: 2 in, 2 out]
                n259 = property on="Sonuçlar" class="Arr (strict)"() -> ("Value"=w756:dbl[][])  [unwired: 2 in, 2 out]
                n260 = Index Array(array=w755, index (row)=2, index (col)=2 ("disabled index (col)")) -> (element=w744:dbl)
                n261 = Index Array(array=w757, index (row)=2, index (col)=1 ("disabled index (col)")) -> (element=w742:dbl)
                n262 = Index Array(array=w756, index (row)=2, index (col)=3 ("disabled index (col)")) -> (element=w743:dbl)
                n263 = Index Array(array=w754, index (row)=2, index (col)=0 ("disabled index (col)")) -> (element=w745:dbl)
              }
              frame "2000" {
                n264 = property on="Sonuçlar" class="Arr (strict)"() -> ("Value"=w773:dbl[][])  [unwired: 2 in, 2 out]
                n265 = property on="Sonuçlar" class="Arr (strict)"() -> ("Value"=w770:dbl[][])  [unwired: 2 in, 2 out]
                n266 = property on="Sonuçlar" class="Arr (strict)"() -> ("Value"=w771:dbl[][])  [unwired: 2 in, 2 out]
                n267 = property on="Sonuçlar" class="Arr (strict)"() -> ("Value"=w772:dbl[][])  [unwired: 2 in, 2 out]
                n268 = Index Array(array=w771, index (row)=3, index (col)=2 ("disabled index (col)")) -> (element=w760:dbl)
                n269 = Index Array(array=w773, index (row)=3, index (col)=1 ("disabled index (col)")) -> (element=w758:dbl)
                n270 = Index Array(array=w772, index (row)=3, index (col)=3 ("disabled index (col)")) -> (element=w759:dbl)
                n271 = Index Array(array=w770, index (row)=3, index (col)=0 ("disabled index (col)")) -> (element=w761:dbl)
              }
              frame "3000" {
                n272 = property on="Sonuçlar" class="Arr (strict)"() -> ("Value"=w787:dbl[][])  [unwired: 2 in, 2 out]
                n273 = property on="Sonuçlar" class="Arr (strict)"() -> ("Value"=w789:dbl[][])  [unwired: 2 in, 2 out]
                n274 = property on="Sonuçlar" class="Arr (strict)"() -> ("Value"=w788:dbl[][])  [unwired: 2 in, 2 out]
                n275 = property on="Sonuçlar" class="Arr (strict)"() -> ("Value"=w786:dbl[][])  [unwired: 2 in, 2 out]
                n276 = Index Array(array=w787, index (row)=4, index (col)=2 ("disabled index (col)")) -> (element=w776:dbl)
                n277 = Index Array(array=w789, index (row)=4, index (col)=1 ("disabled index (col)")) -> (element=w774:dbl)
                n278 = Index Array(array=w788, index (row)=4, index (col)=3 ("disabled index (col)")) -> (element=w775:dbl)
                n279 = Index Array(array=w786, index (row)=4, index (col)=0 ("disabled index (col)")) -> (element=w777:dbl)
              }
              frame "4000" {
                n280 = property on="Sonuçlar" class="Arr (strict)"() -> ("Value"=w805:dbl[][])  [unwired: 2 in, 2 out]
                n281 = property on="Sonuçlar" class="Arr (strict)"() -> ("Value"=w804:dbl[][])  [unwired: 2 in, 2 out]
                n282 = property on="Sonuçlar" class="Arr (strict)"() -> ("Value"=w802:dbl[][])  [unwired: 2 in, 2 out]
                n283 = property on="Sonuçlar" class="Arr (strict)"() -> ("Value"=w803:dbl[][])  [unwired: 2 in, 2 out]
                n284 = Index Array(array=w804, index (row)=5, index (col)=2 ("disabled index (col)")) -> (element=w792:dbl)
                n285 = Index Array(array=w802, index (row)=5 ("disabled index (row)"), index (col)=1 ("disabled index (col)")) -> (element=w790:dbl)
                n286 = Index Array(array=w803, index (row)=5, index (col)=3 ("disabled index (col)")) -> (element=w791:dbl)
                n287 = Index Array(array=w805, index (row)=5, index (col)=0 ("disabled index (col)")) -> (element=w793:dbl)
              }
              frame "5000" {
                n288 = property on="Sonuçlar" class="Arr (strict)"() -> ("Value"=w818:dbl[][])  [unwired: 2 in, 2 out]
                n289 = property on="Sonuçlar" class="Arr (strict)"() -> ("Value"=w819:dbl[][])  [unwired: 2 in, 2 out]
                n290 = property on="Sonuçlar" class="Arr (strict)"() -> ("Value"=w821:dbl[][])  [unwired: 2 in, 2 out]
                n291 = property on="Sonuçlar" class="Arr (strict)"() -> ("Value"=w820:dbl[][])  [unwired: 2 in, 2 out]
                n292 = Index Array(array=w819, index (row)=6, index (col)=2 ("disabled index (col)")) -> (element=w808:dbl)
                n293 = Index Array(array=w821, index (row)=6, index (col)=1 ("disabled index (col)")) -> (element=w806:dbl)
                n294 = Index Array(array=w820, index (row)=6 ("disabled index (row)"), index (col)=3 ("disabled index (col)")) -> (element=w807:dbl)
                n295 = Index Array(array=w818, index (row)=6, index (col)=0 ("disabled index (col)")) -> (element=w809:dbl)
              }
              frame "6000" {
                n296 = property on="Sonuçlar" class="Arr (strict)"() -> ("Value"=w832:dbl[][])  [unwired: 2 in, 2 out]
                n297 = property on="Sonuçlar" class="Arr (strict)"() -> ("Value"=w833:dbl[][])  [unwired: 2 in, 2 out]
                n298 = property on="Sonuçlar" class="Arr (strict)"() -> ("Value"=w830:dbl[][])  [unwired: 2 in, 2 out]
                n299 = property on="Sonuçlar" class="Arr (strict)"() -> ("Value"=w831:dbl[][])  [unwired: 2 in, 2 out]
                n300 = Index Array(array=w832, index (row)=7 ("index"), index (col)=2 ("disabled index (col)")) -> (element=w827:dbl)
                n301 = Index Array(array=w830, index (row)=7 ("index"), index (col)=1 ("disabled index (col)")) -> (element=w822:dbl)
                n302 = Index Array(array=w831, index (row)=7 ("index"), index (col)=3 ("disabled index (col)")) -> (element=w824:dbl)
                n303 = Index Array(array=w833, index (row)=7 ("index"), index (col)=0 ("disabled index (col)")) -> (element=w826:dbl)
              }
              frame "7000" {
                n304 = property on="Sonuçlar" class="Arr (strict)"() -> ("Value"=w849:dbl[][])  [unwired: 2 in, 2 out]
                n305 = property on="Sonuçlar" class="Arr (strict)"() -> ("Value"=w848:dbl[][])  [unwired: 2 in, 2 out]
                n306 = property on="Sonuçlar" class="Arr (strict)"() -> ("Value"=w846:dbl[][])  [unwired: 2 in, 2 out]
                n307 = property on="Sonuçlar" class="Arr (strict)"() -> ("Value"=w847:dbl[][])  [unwired: 2 in, 2 out]
                n308 = Index Array(array=w848, index (row)=8 ("index"), index (col)=2 ("disabled index (col)")) -> (element=w844:dbl)
                n309 = Index Array(array=w846, index (row)=8 ("index"), index (col)=1 ("disabled index (col)")) -> (element=w842:dbl)
                n310 = Index Array(array=w847, index (row)=8 ("index"), index (col)=3 ("disabled index (col)")) -> (element=w843:dbl)
                n311 = Index Array(array=w849, index (row)=8 ("index"), index (col)=0 ("disabled index (col)")) -> (element=w845:dbl)
              }
              frame "8000" {
                n312 = property on="Sonuçlar" class="Arr (strict)"() -> ("Value"=w865:dbl[][])  [unwired: 2 in, 2 out]
                n313 = property on="Sonuçlar" class="Arr (strict)"() -> ("Value"=w863:dbl[][])  [unwired: 2 in, 2 out]
                n314 = property on="Sonuçlar" class="Arr (strict)"() -> ("Value"=w864:dbl[][])  [unwired: 2 in, 2 out]
                n315 = property on="Sonuçlar" class="Arr (strict)"() -> ("Value"=w862:dbl[][])  [unwired: 2 in, 2 out]
                n316 = Index Array(array=w863, index (row)=9 ("index"), index (col)=2 ("disabled index (col)")) -> (element=w857:dbl)
                n317 = Index Array(array=w864, index (row)=9 ("index"), index (col)=1 ("disabled index (col)")) -> (element=w856:dbl)
                n318 = Index Array(array=w862, index (row)=9 ("index"), index (col)=3 ("disabled index (col)")) -> (element=w855:dbl)
                n319 = Index Array(array=w865, index (row)=9 ("index"), index (col)=0 ("disabled index (col)")) -> (element=w854:dbl)
              }
              frame "9000" {
                n320 = property on="Sonuçlar" class="Arr (strict)"() -> ("Value"=w878:dbl[][])  [unwired: 2 in, 2 out]
                n321 = property on="Sonuçlar" class="Arr (strict)"() -> ("Value"=w879:dbl[][])  [unwired: 2 in, 2 out]
                n322 = property on="Sonuçlar" class="Arr (strict)"() -> ("Value"=w881:dbl[][])  [unwired: 2 in, 2 out]
                n323 = property on="Sonuçlar" class="Arr (strict)"() -> ("Value"=w880:dbl[][])  [unwired: 2 in, 2 out]
                n324 = Index Array(array=w879, index (row)=10 ("index"), index (col)=2 ("disabled index (col)")) -> (element=w872:dbl)
                n325 = Index Array(array=w881, index (row)=10 ("index"), index (col)=1 ("disabled index (col)")) -> (element=w870:dbl)
                n326 = Index Array(array=w880, index (row)=10 ("index"), index (col)=3 ("disabled index (col)")) -> (element=w871:dbl)
                n327 = Index Array(array=w878, index (row)=10 ("index"), index (col)=0 ("disabled index (col)")) -> (element=w873:dbl)
              }
              frame "10000" {
                n328 = property on="Sonuçlar" class="Arr (strict)"() -> ("Value"=w894:dbl[][])  [unwired: 2 in, 2 out]
                n329 = property on="Sonuçlar" class="Arr (strict)"() -> ("Value"=w895:dbl[][])  [unwired: 2 in, 2 out]
                n330 = property on="Sonuçlar" class="Arr (strict)"() -> ("Value"=w897:dbl[][])  [unwired: 2 in, 2 out]
                n331 = property on="Sonuçlar" class="Arr (strict)"() -> ("Value"=w896:dbl[][])  [unwired: 2 in, 2 out]
                n332 = Index Array(array=w895, index (row)=11 ("index"), index (col)=2 ("disabled index (col)")) -> (element=w887:dbl)
                n333 = Index Array(array=w897, index (row)=11 ("index"), index (col)=1 ("disabled index (col)")) -> (element=w889:dbl)
                n334 = Index Array(array=w896, index (row)=11 ("index"), index (col)=3 ("disabled index (col)")) -> (element=w888:dbl)
                n335 = Index Array(array=w894, index (row)=11 ("index"), index (col)=0 ("disabled index (col)")) -> (element=w886:dbl)
              }
            }
          }
        }
      }
      frame "Glenoid Yuva" {
        n336 = case shown="\"Burulma Gerilmesi\"" w906 {
          tunnel: w907 -> [_ w912 w1109]
          tunnel: [_ w911 w1108] -> w905
          tunnel: [_ w910 w1107] -> w904
          tunnel: [_ w909 w1106] -> w903
          tunnel: [_ w908 w1105] -> w902
          frame "False", Default {
          }
          frame "Burulma Gerilmesi" {
            n337 = case shown="\"10000\"" w912 {
              tunnel: [_ w916 w932 w948 w964 w980 w999 w1015 w1031 w1048 w1064 w1080 w1096] -> w911
              tunnel: [_ w915 w931 w947 w963 w979 w998 w1013 w1030 w1046 w1061 w1077 w1095] -> w910
              tunnel: [_ w914 w930 w946 w962 w978 w995 w1011 w1029 w1043 w1060 w1076 w1093] -> w909
              tunnel: [_ w913 w929 w945 w961 w977 w993 w1009 w1028 w1042 w1058 w1073 w1091] -> w908
              frame "False", Default {
              }
              frame "100" {
                n338 = property on="Sonuçlar" class="Arr (strict)"() -> ("Value"=w921:dbl[][])  [unwired: 2 in, 2 out]
                n339 = property on="Sonuçlar" class="Arr (strict)"() -> ("Value"=w919:dbl[][])  [unwired: 2 in, 2 out]
                n340 = property on="Sonuçlar" class="Arr (strict)"() -> ("Value"=w917:dbl[][])  [unwired: 2 in, 2 out]
                n341 = property on="Sonuçlar" class="Arr (strict)"() -> ("Value"=w918:dbl[][])  [unwired: 2 in, 2 out]
                n342 = Index Array(array=w921, index (row)=12 ("index"), index (col)=6 ("disabled index (col)")) -> (element=w916:dbl)
                n343 = Index Array(array=w919, index (row)=12 ("index"), index (col)=5 ("disabled index (col)")) -> (element=w915:dbl)
                n344 = Index Array(array=w917, index (row)=12 ("index"), index (col)=7 ("disabled index (col)")) -> (element=w913:dbl)
                n345 = Index Array(array=w918, index (row)=12 ("index"), index (col)=4 ("disabled index (col)")) -> (element=w914:dbl)
              }
              frame "500" {
                n346 = property on="Sonuçlar" class="Arr (strict)"() -> ("Value"=w934:dbl[][])  [unwired: 2 in, 2 out]
                n347 = property on="Sonuçlar" class="Arr (strict)"() -> ("Value"=w935:dbl[][])  [unwired: 2 in, 2 out]
                n348 = property on="Sonuçlar" class="Arr (strict)"() -> ("Value"=w937:dbl[][])  [unwired: 2 in, 2 out]
                n349 = property on="Sonuçlar" class="Arr (strict)"() -> ("Value"=w936:dbl[][])  [unwired: 2 in, 2 out]
                n350 = Index Array(array=w934, index (row)=13 ("index"), index (col)=6 ("disabled index (col)")) -> (element=w932:dbl)
                n351 = Index Array(array=w935, index (row)=13 ("index"), index (col)=5 ("disabled index (col)")) -> (element=w931:dbl)
                n352 = Index Array(array=w937, index (row)=13 ("index"), index (col)=7 ("disabled index (col)")) -> (element=w929:dbl)
                n353 = Index Array(array=w936, index (row)=13 ("index"), index (col)=4 ("disabled index (col)")) -> (element=w930:dbl)
              }
              frame "1000" {
                n354 = property on="Sonuçlar" class="Arr (strict)"() -> ("Value"=w950:dbl[][])  [unwired: 2 in, 2 out]
                n355 = property on="Sonuçlar" class="Arr (strict)"() -> ("Value"=w951:dbl[][])  [unwired: 2 in, 2 out]
                n356 = property on="Sonuçlar" class="Arr (strict)"() -> ("Value"=w953:dbl[][])  [unwired: 2 in, 2 out]
                n357 = property on="Sonuçlar" class="Arr (strict)"() -> ("Value"=w952:dbl[][])  [unwired: 2 in, 2 out]
                n358 = Index Array(array=w950, index (row)=14 ("index"), index (col)=6 ("disabled index (col)")) -> (element=w948:dbl)
                n359 = Index Array(array=w951, index (row)=14 ("index"), index (col)=5 ("disabled index (col)")) -> (element=w947:dbl)
                n360 = Index Array(array=w953, index (row)=14 ("index"), index (col)=7 ("disabled index (col)")) -> (element=w945:dbl)
                n361 = Index Array(array=w952, index (row)=14 ("index"), index (col)=4 ("disabled index (col)")) -> (element=w946:dbl)
              }
              frame "2000" {
                n362 = property on="Sonuçlar" class="Arr (strict)"() -> ("Value"=w969:dbl[][])  [unwired: 2 in, 2 out]
                n363 = property on="Sonuçlar" class="Arr (strict)"() -> ("Value"=w967:dbl[][])  [unwired: 2 in, 2 out]
                n364 = property on="Sonuçlar" class="Arr (strict)"() -> ("Value"=w965:dbl[][])  [unwired: 2 in, 2 out]
                n365 = property on="Sonuçlar" class="Arr (strict)"() -> ("Value"=w966:dbl[][])  [unwired: 2 in, 2 out]
                n366 = Index Array(array=w969, index (row)=15 ("index"), index (col)=6 ("disabled index (col)")) -> (element=w964:dbl)
                n367 = Index Array(array=w967, index (row)=15 ("index"), index (col)=5 ("disabled index (col)")) -> (element=w963:dbl)
                n368 = Index Array(array=w965, index (row)=15 ("index"), index (col)=7 ("disabled index (col)")) -> (element=w961:dbl)
                n369 = Index Array(array=w966, index (row)=15 ("index"), index (col)=4 ("disabled index (col)")) -> (element=w962:dbl)
              }
              frame "3000" {
                n370 = property on="Sonuçlar" class="Arr (strict)"() -> ("Value"=w985:dbl[][])  [unwired: 2 in, 2 out]
                n371 = property on="Sonuçlar" class="Arr (strict)"() -> ("Value"=w983:dbl[][])  [unwired: 2 in, 2 out]
                n372 = property on="Sonuçlar" class="Arr (strict)"() -> ("Value"=w981:dbl[][])  [unwired: 2 in, 2 out]
                n373 = property on="Sonuçlar" class="Arr (strict)"() -> ("Value"=w982:dbl[][])  [unwired: 2 in, 2 out]
                n374 = Index Array(array=w985, index (row)=16 ("index"), index (col)=6 ("disabled index (col)")) -> (element=w980:dbl)
                n375 = Index Array(array=w983, index (row)=16 ("index"), index (col)=5 ("disabled index (col)")) -> (element=w979:dbl)
                n376 = Index Array(array=w981, index (row)=16 ("index"), index (col)=7 ("disabled index (col)")) -> (element=w977:dbl)
                n377 = Index Array(array=w982, index (row)=16 ("index"), index (col)=4 ("disabled index (col)")) -> (element=w978:dbl)
              }
              frame "4000" {
                n378 = property on="Sonuçlar" class="Arr (strict)"() -> ("Value"=w1001:dbl[][])  [unwired: 2 in, 2 out]
                n379 = property on="Sonuçlar" class="Arr (strict)"() -> ("Value"=w997:dbl[][])  [unwired: 2 in, 2 out]
                n380 = property on="Sonuçlar" class="Arr (strict)"() -> ("Value"=w994:dbl[][])  [unwired: 2 in, 2 out]
                n381 = property on="Sonuçlar" class="Arr (strict)"() -> ("Value"=w996:dbl[][])  [unwired: 2 in, 2 out]
                n382 = Index Array(array=w1001, index (row)=17 ("index"), index (col)=6 ("disabled index (col)")) -> (element=w999:dbl)
                n383 = Index Array(array=w997, index (row)=17 ("index"), index (col)=5 ("disabled index (col)")) -> (element=w998:dbl)
                n384 = Index Array(array=w994, index (row)=17 ("index"), index (col)=7 ("disabled index (col)")) -> (element=w993:dbl)
                n385 = Index Array(array=w996, index (row)=17 ("index"), index (col)=4 ("disabled index (col)")) -> (element=w995:dbl)
              }
              frame "5000" {
                n386 = property on="Sonuçlar" class="Arr (strict)"() -> ("Value"=w1017:dbl[][])  [unwired: 2 in, 2 out]
                n387 = property on="Sonuçlar" class="Arr (strict)"() -> ("Value"=w1014:dbl[][])  [unwired: 2 in, 2 out]
                n388 = property on="Sonuçlar" class="Arr (strict)"() -> ("Value"=w1010:dbl[][])  [unwired: 2 in, 2 out]
                n389 = property on="Sonuçlar" class="Arr (strict)"() -> ("Value"=w1012:dbl[][])  [unwired: 2 in, 2 out]
                n390 = Index Array(array=w1017, index (row)=18 ("index"), index (col)=6 ("disabled index (col)")) -> (element=w1015:dbl)
                n391 = Index Array(array=w1014, index (row)=18 ("index"), index (col)=5 ("disabled index (col)")) -> (element=w1013:dbl)
                n392 = Index Array(array=w1010, index (row)=18 ("index"), index (col)=7 ("disabled index (col)")) -> (element=w1009:dbl)
                n393 = Index Array(array=w1012, index (row)=18 ("index"), index (col)=4 ("disabled index (col)")) -> (element=w1011:dbl)
              }
              frame "6000" {
                n394 = property on="Sonuçlar" class="Arr (strict)"() -> ("Value"=w1033:dbl[][])  [unwired: 2 in, 2 out]
                n395 = property on="Sonuçlar" class="Arr (strict)"() -> ("Value"=w1025:dbl[][])  [unwired: 2 in, 2 out]
                n396 = property on="Sonuçlar" class="Arr (strict)"() -> ("Value"=w1027:dbl[][])  [unwired: 2 in, 2 out]
                n397 = property on="Sonuçlar" class="Arr (strict)"() -> ("Value"=w1026:dbl[][])  [unwired: 2 in, 2 out]
                n398 = Index Array(array=w1033, index (row)=19 ("index"), index (col)=6 ("disabled index (col)")) -> (element=w1031:dbl)
                n399 = Index Array(array=w1025, index (row)=19 ("index"), index (col)=5 ("disabled index (col)")) -> (element=w1030:dbl)
                n400 = Index Array(array=w1027, index (row)=19 ("index"), index (col)=7 ("disabled index (col)")) -> (element=w1028:dbl)
                n401 = Index Array(array=w1026, index (row)=19 ("index"), index (col)=4 ("disabled index (col)")) -> (element=w1029:dbl)
              }
              frame "7000" {
                n402 = property on="Sonuçlar" class="Arr (strict)"() -> ("Value"=w1049:dbl[][])  [unwired: 2 in, 2 out]
                n403 = property on="Sonuçlar" class="Arr (strict)"() -> ("Value"=w1045:dbl[][])  [unwired: 2 in, 2 out]
                n404 = property on="Sonuçlar" class="Arr (strict)"() -> ("Value"=w1041:dbl[][])  [unwired: 2 in, 2 out]
                n405 = property on="Sonuçlar" class="Arr (strict)"() -> ("Value"=w1044:dbl[][])  [unwired: 2 in, 2 out]
                n406 = Index Array(array=w1049, index (row)=20 ("index"), index (col)=6 ("disabled index (col)")) -> (element=w1048:dbl)
                n407 = Index Array(array=w1045, index (row)=20 ("index"), index (col)=5 ("disabled index (col)")) -> (element=w1046:dbl)
                n408 = Index Array(array=w1041, index (row)=20 ("index"), index (col)=7 ("disabled index (col)")) -> (element=w1042:dbl)
                n409 = Index Array(array=w1044, index (row)=20 ("index"), index (col)=4 ("disabled index (col)")) -> (element=w1043:dbl)
              }
              frame "8000" {
                n410 = property on="Sonuçlar" class="Arr (strict)"() -> ("Value"=w1065:dbl[][])  [unwired: 2 in, 2 out]
                n411 = property on="Sonuçlar" class="Arr (strict)"() -> ("Value"=w1062:dbl[][])  [unwired: 2 in, 2 out]
                n412 = property on="Sonuçlar" class="Arr (strict)"() -> ("Value"=w1057:dbl[][])  [unwired: 2 in, 2 out]
                n413 = property on="Sonuçlar" class="Arr (strict)"() -> ("Value"=w1059:dbl[][])  [unwired: 2 in, 2 out]
                n414 = Index Array(array=w1065, index (row)=21 ("index"), index (col)=6 ("disabled index (col)")) -> (element=w1064:dbl)
                n415 = Index Array(array=w1062, index (row)=21 ("index"), index (col)=5 ("disabled index (col)")) -> (element=w1061:dbl)
                n416 = Index Array(array=w1057, index (row)=21 ("index"), index (col)=7 ("disabled index (col)")) -> (element=w1058:dbl)
                n417 = Index Array(array=w1059, index (row)=21 ("index"), index (col)=4 ("disabled index (col)")) -> (element=w1060:dbl)
              }
              frame "9000" {
                n418 = property on="Sonuçlar" class="Arr (strict)"() -> ("Value"=w1081:dbl[][])  [unwired: 2 in, 2 out]
                n419 = property on="Sonuçlar" class="Arr (strict)"() -> ("Value"=w1078:dbl[][])  [unwired: 2 in, 2 out]
                n420 = property on="Sonuçlar" class="Arr (strict)"() -> ("Value"=w1074:dbl[][])  [unwired: 2 in, 2 out]
                n421 = property on="Sonuçlar" class="Arr (strict)"() -> ("Value"=w1075:dbl[][])  [unwired: 2 in, 2 out]
                n422 = Index Array(array=w1081, index (row)=22 ("index"), index (col)=6 ("disabled index (col)")) -> (element=w1080:dbl)
                n423 = Index Array(array=w1078, index (row)=22 ("index"), index (col)=5 ("disabled index (col)")) -> (element=w1077:dbl)
                n424 = Index Array(array=w1074, index (row)=22 ("index"), index (col)=7 ("disabled index (col)")) -> (element=w1073:dbl)
                n425 = Index Array(array=w1075, index (row)=22 ("index"), index (col)=4 ("disabled index (col)")) -> (element=w1076:dbl)
              }
              frame "10000" {
                n426 = property on="Sonuçlar" class="Arr (strict)"() -> ("Value"=w1097:dbl[][])  [unwired: 2 in, 2 out]
                n427 = property on="Sonuçlar" class="Arr (strict)"() -> ("Value"=w1094:dbl[][])  [unwired: 2 in, 2 out]
                n428 = property on="Sonuçlar" class="Arr (strict)"() -> ("Value"=w1090:dbl[][])  [unwired: 2 in, 2 out]
                n429 = property on="Sonuçlar" class="Arr (strict)"() -> ("Value"=w1092:dbl[][])  [unwired: 2 in, 2 out]
                n430 = Index Array(array=w1097, index (row)=23 ("index"), index (col)=6 ("disabled index (col)")) -> (element=w1096:dbl)
                n431 = Index Array(array=w1094, index (row)=23 ("index"), index (col)=5 ("disabled index (col)")) -> (element=w1095:dbl)
                n432 = Index Array(array=w1090, index (row)=23 ("index"), index (col)=7 ("disabled index (col)")) -> (element=w1091:dbl)
                n433 = Index Array(array=w1092, index (row)=23 ("index"), index (col)=4 ("disabled index (col)")) -> (element=w1093:dbl)
              }
            }
          }
          frame "Basma Gerilmesi" {
            n434 = case shown="\"10000\"" w1109 {
              tunnel: [_ w1113 w1129 w1145 w1161 w1177 w1193 w1209 w1225 w1241 w1257 w1270 w1289] -> w1108
              tunnel: [_ w1112 w1128 w1144 w1160 w1176 w1192 w1208 w1224 w1240 w1256 w1271 w1288] -> w1107
              tunnel: [_ w1111 w1127 w1143 w1159 w1175 w1191 w1207 w1223 w1239 w1255 w1272 w1287] -> w1106
              tunnel: [_ w1110 w1126 w1142 w1158 w1174 w1190 w1206 w1222 w1238 w1254 w1273 w1286] -> w1105
              frame "False", Default {
              }
              frame "100" {
                n435 = property on="Sonuçlar" class="Arr (strict)"() -> ("Value"=w1121:dbl[][])  [unwired: 2 in, 2 out]
                n436 = property on="Sonuçlar" class="Arr (strict)"() -> ("Value"=w1119:dbl[][])  [unwired: 2 in, 2 out]
                n437 = property on="Sonuçlar" class="Arr (strict)"() -> ("Value"=w1115:dbl[][])  [unwired: 2 in, 2 out]
                n438 = property on="Sonuçlar" class="Arr (strict)"() -> ("Value"=w1117:dbl[][])  [unwired: 2 in, 2 out]
                n439 = Index Array(array=w1121, index (row)=0 ("index"), index (col)=6 ("disabled index (col)")) -> (element=w1113:dbl)
                n440 = Index Array(array=w1119, index (row)=0 ("index"), index (col)=5 ("disabled index (col)")) -> (element=w1112:dbl)
                n441 = Index Array(array=w1115, index (row)=0 ("index"), index (col)=7 ("disabled index (col)")) -> (element=w1110:dbl)
                n442 = Index Array(array=w1117, index (row)=0 ("index"), index (col)=4 ("disabled index (col)")) -> (element=w1111:dbl)
              }
              frame "500" {
                n443 = property on="Sonuçlar" class="Arr (strict)"() -> ("Value"=w1131:dbl[][])  [unwired: 2 in, 2 out]
                n444 = property on="Sonuçlar" class="Arr (strict)"() -> ("Value"=w1133:dbl[][])  [unwired: 2 in, 2 out]
                n445 = property on="Sonuçlar" class="Arr (strict)"() -> ("Value"=w1132:dbl[][])  [unwired: 2 in, 2 out]
                n446 = property on="Sonuçlar" class="Arr (strict)"() -> ("Value"=w1134:dbl[][])  [unwired: 2 in, 2 out]
                n447 = Index Array(array=w1131, index (row)=1 ("index"), index (col)=6 ("disabled index (col)")) -> (element=w1129:dbl)
                n448 = Index Array(array=w1133, index (row)=1 ("index"), index (col)=5 ("disabled index (col)")) -> (element=w1128:dbl)
                n449 = Index Array(array=w1132, index (row)=1 ("index"), index (col)=7 ("disabled index (col)")) -> (element=w1126:dbl)
                n450 = Index Array(array=w1134, index (row)=1 ("index"), index (col)=4 ("disabled index (col)")) -> (element=w1127:dbl)
              }
              frame "1000" {
                n451 = property on="Sonuçlar" class="Arr (strict)"() -> ("Value"=w1147:dbl[][])  [unwired: 2 in, 2 out]
                n452 = property on="Sonuçlar" class="Arr (strict)"() -> ("Value"=w1148:dbl[][])  [unwired: 2 in, 2 out]
                n453 = property on="Sonuçlar" class="Arr (strict)"() -> ("Value"=w1150:dbl[][])  [unwired: 2 in, 2 out]
                n454 = property on="Sonuçlar" class="Arr (strict)"() -> ("Value"=w1149:dbl[][])  [unwired: 2 in, 2 out]
                n455 = Index Array(array=w1147, index (row)=2 ("index"), index (col)=6 ("disabled index (col)")) -> (element=w1145:dbl)
                n456 = Index Array(array=w1148, index (row)=2 ("index"), index (col)=5 ("disabled index (col)")) -> (element=w1144:dbl)
                n457 = Index Array(array=w1150, index (row)=2 ("index"), index (col)=7 ("disabled index (col)")) -> (element=w1142:dbl)
                n458 = Index Array(array=w1149, index (row)=2 ("index"), index (col)=4 ("disabled index (col)")) -> (element=w1143:dbl)
              }
              frame "2000" {
                n459 = property on="Sonuçlar" class="Arr (strict)"() -> ("Value"=w1163:dbl[][])  [unwired: 2 in, 2 out]
                n460 = property on="Sonuçlar" class="Arr (strict)"() -> ("Value"=w1164:dbl[][])  [unwired: 2 in, 2 out]
                n461 = property on="Sonuçlar" class="Arr (strict)"() -> ("Value"=w1166:dbl[][])  [unwired: 2 in, 2 out]
                n462 = property on="Sonuçlar" class="Arr (strict)"() -> ("Value"=w1165:dbl[][])  [unwired: 2 in, 2 out]
                n463 = Index Array(array=w1163, index (row)=3 ("index"), index (col)=6 ("disabled index (col)")) -> (element=w1161:dbl)
                n464 = Index Array(array=w1164, index (row)=3 ("index"), index (col)=5 ("disabled index (col)")) -> (element=w1160:dbl)
                n465 = Index Array(array=w1166, index (row)=3 ("index"), index (col)=7 ("disabled index (col)")) -> (element=w1158:dbl)
                n466 = Index Array(array=w1165, index (row)=3 ("index"), index (col)=4 ("disabled index (col)")) -> (element=w1159:dbl)
              }
              frame "3000" {
                n467 = property on="Sonuçlar" class="Arr (strict)"() -> ("Value"=w1179:dbl[][])  [unwired: 2 in, 2 out]
                n468 = property on="Sonuçlar" class="Arr (strict)"() -> ("Value"=w1180:dbl[][])  [unwired: 2 in, 2 out]
                n469 = property on="Sonuçlar" class="Arr (strict)"() -> ("Value"=w1182:dbl[][])  [unwired: 2 in, 2 out]
                n470 = property on="Sonuçlar" class="Arr (strict)"() -> ("Value"=w1181:dbl[][])  [unwired: 2 in, 2 out]
                n471 = Index Array(array=w1179, index (row)=4 ("index"), index (col)=6 ("disabled index (col)")) -> (element=w1177:dbl)
                n472 = Index Array(array=w1180, index (row)=4 ("index"), index (col)=5 ("disabled index (col)")) -> (element=w1176:dbl)
                n473 = Index Array(array=w1182, index (row)=4 ("index"), index (col)=7 ("disabled index (col)")) -> (element=w1174:dbl)
                n474 = Index Array(array=w1181, index (row)=4 ("index"), index (col)=4 ("disabled index (col)")) -> (element=w1175:dbl)
              }
              frame "4000" {
                n475 = property on="Sonuçlar" class="Arr (strict)"() -> ("Value"=w1195:dbl[][])  [unwired: 2 in, 2 out]
                n476 = property on="Sonuçlar" class="Arr (strict)"() -> ("Value"=w1196:dbl[][])  [unwired: 2 in, 2 out]
                n477 = property on="Sonuçlar" class="Arr (strict)"() -> ("Value"=w1198:dbl[][])  [unwired: 2 in, 2 out]
                n478 = property on="Sonuçlar" class="Arr (strict)"() -> ("Value"=w1197:dbl[][])  [unwired: 2 in, 2 out]
                n479 = Index Array(array=w1195, index (row)=5 ("index"), index (col)=6 ("disabled index (col)")) -> (element=w1193:dbl)
                n480 = Index Array(array=w1196, index (row)=5 ("index"), index (col)=5 ("disabled index (col)")) -> (element=w1192:dbl)
                n481 = Index Array(array=w1198, index (row)=5 ("index"), index (col)=7 ("disabled index (col)")) -> (element=w1190:dbl)
                n482 = Index Array(array=w1197, index (row)=5 ("index"), index (col)=4 ("disabled index (col)")) -> (element=w1191:dbl)
              }
              frame "5000" {
                n483 = property on="Sonuçlar" class="Arr (strict)"() -> ("Value"=w1211:dbl[][])  [unwired: 2 in, 2 out]
                n484 = property on="Sonuçlar" class="Arr (strict)"() -> ("Value"=w1212:dbl[][])  [unwired: 2 in, 2 out]
                n485 = property on="Sonuçlar" class="Arr (strict)"() -> ("Value"=w1214:dbl[][])  [unwired: 2 in, 2 out]
                n486 = property on="Sonuçlar" class="Arr (strict)"() -> ("Value"=w1213:dbl[][])  [unwired: 2 in, 2 out]
                n487 = Index Array(array=w1211, index (row)=6 ("index"), index (col)=6 ("disabled index (col)")) -> (element=w1209:dbl)
                n488 = Index Array(array=w1212, index (row)=6 ("index"), index (col)=5 ("disabled index (col)")) -> (element=w1208:dbl)
                n489 = Index Array(array=w1214, index (row)=6 ("index"), index (col)=7 ("disabled index (col)")) -> (element=w1206:dbl)
                n490 = Index Array(array=w1213, index (row)=6 ("index"), index (col)=4 ("disabled index (col)")) -> (element=w1207:dbl)
              }
              frame "6000" {
                n491 = property on="Sonuçlar" class="Arr (strict)"() -> ("Value"=w1227:dbl[][])  [unwired: 2 in, 2 out]
                n492 = property on="Sonuçlar" class="Arr (strict)"() -> ("Value"=w1228:dbl[][])  [unwired: 2 in, 2 out]
                n493 = property on="Sonuçlar" class="Arr (strict)"() -> ("Value"=w1230:dbl[][])  [unwired: 2 in, 2 out]
                n494 = property on="Sonuçlar" class="Arr (strict)"() -> ("Value"=w1229:dbl[][])  [unwired: 2 in, 2 out]
                n495 = Index Array(array=w1227, index (row)=7 ("index"), index (col)=6 ("disabled index (col)")) -> (element=w1225:dbl)
                n496 = Index Array(array=w1228, index (row)=7 ("index"), index (col)=5 ("disabled index (col)")) -> (element=w1224:dbl)
                n497 = Index Array(array=w1230, index (row)=7 ("index"), index (col)=7 ("disabled index (col)")) -> (element=w1222:dbl)
                n498 = Index Array(array=w1229, index (row)=7 ("index"), index (col)=4 ("disabled index (col)")) -> (element=w1223:dbl)
              }
              frame "7000" {
                n499 = property on="Sonuçlar" class="Arr (strict)"() -> ("Value"=w1243:dbl[][])  [unwired: 2 in, 2 out]
                n500 = property on="Sonuçlar" class="Arr (strict)"() -> ("Value"=w1244:dbl[][])  [unwired: 2 in, 2 out]
                n501 = property on="Sonuçlar" class="Arr (strict)"() -> ("Value"=w1246:dbl[][])  [unwired: 2 in, 2 out]
                n502 = property on="Sonuçlar" class="Arr (strict)"() -> ("Value"=w1245:dbl[][])  [unwired: 2 in, 2 out]
                n503 = Index Array(array=w1243, index (row)=8 ("index"), index (col)=6 ("disabled index (col)")) -> (element=w1241:dbl)
                n504 = Index Array(array=w1244, index (row)=8 ("index"), index (col)=5 ("disabled index (col)")) -> (element=w1240:dbl)
                n505 = Index Array(array=w1246, index (row)=8 ("index"), index (col)=7 ("disabled index (col)")) -> (element=w1238:dbl)
                n506 = Index Array(array=w1245, index (row)=8 ("index"), index (col)=4 ("disabled index (col)")) -> (element=w1239:dbl)
              }
              frame "8000" {
                n507 = property on="Sonuçlar" class="Arr (strict)"() -> ("Value"=w1259:dbl[][])  [unwired: 2 in, 2 out]
                n508 = property on="Sonuçlar" class="Arr (strict)"() -> ("Value"=w1260:dbl[][])  [unwired: 2 in, 2 out]
                n509 = property on="Sonuçlar" class="Arr (strict)"() -> ("Value"=w1262:dbl[][])  [unwired: 2 in, 2 out]
                n510 = property on="Sonuçlar" class="Arr (strict)"() -> ("Value"=w1261:dbl[][])  [unwired: 2 in, 2 out]
                n511 = Index Array(array=w1259, index (row)=9 ("index"), index (col)=6 ("disabled index (col)")) -> (element=w1257:dbl)
                n512 = Index Array(array=w1260, index (row)=9 ("index"), index (col)=5 ("disabled index (col)")) -> (element=w1256:dbl)
                n513 = Index Array(array=w1262, index (row)=9 ("index"), index (col)=7 ("disabled index (col)")) -> (element=w1254:dbl)
                n514 = Index Array(array=w1261, index (row)=9 ("index"), index (col)=4 ("disabled index (col)")) -> (element=w1255:dbl)
              }
              frame "9000" {
                n515 = property on="Sonuçlar" class="Arr (strict)"() -> ("Value"=w1278:dbl[][])  [unwired: 2 in, 2 out]
                n516 = property on="Sonuçlar" class="Arr (strict)"() -> ("Value"=w1276:dbl[][])  [unwired: 2 in, 2 out]
                n517 = property on="Sonuçlar" class="Arr (strict)"() -> ("Value"=w1274:dbl[][])  [unwired: 2 in, 2 out]
                n518 = property on="Sonuçlar" class="Arr (strict)"() -> ("Value"=w1275:dbl[][])  [unwired: 2 in, 2 out]
                n519 = Index Array(array=w1278, index (row)=10 ("index"), index (col)=6 ("disabled index (col)")) -> (element=w1270:dbl)
                n520 = Index Array(array=w1276, index (row)=10 ("index"), index (col)=5 ("disabled index (col)")) -> (element=w1271:dbl)
                n521 = Index Array(array=w1274, index (row)=10 ("index"), index (col)=7 ("disabled index (col)")) -> (element=w1273:dbl)
                n522 = Index Array(array=w1275, index (row)=10 ("index"), index (col)=4 ("disabled index (col)")) -> (element=w1272:dbl)
              }
              frame "10000" {
                n523 = property on="Sonuçlar" class="Arr (strict)"() -> ("Value"=w1291:dbl[][])  [unwired: 2 in, 2 out]
                n524 = property on="Sonuçlar" class="Arr (strict)"() -> ("Value"=w1292:dbl[][])  [unwired: 2 in, 2 out]
                n525 = property on="Sonuçlar" class="Arr (strict)"() -> ("Value"=w1294:dbl[][])  [unwired: 2 in, 2 out]
                n526 = property on="Sonuçlar" class="Arr (strict)"() -> ("Value"=w1293:dbl[][])  [unwired: 2 in, 2 out]
                n527 = Index Array(array=w1291, index (row)=11 ("index"), index (col)=6 ("disabled index (col)")) -> (element=w1289:dbl)
                n528 = Index Array(array=w1292, index (row)=11 ("index"), index (col)=5 ("disabled index (col)")) -> (element=w1288:dbl)
                n529 = Index Array(array=w1294, index (row)=11 ("index"), index (col)=7 ("disabled index (col)")) -> (element=w1286:dbl)
                n530 = Index Array(array=w1293, index (row)=11 ("index"), index (col)=4 ("disabled index (col)")) -> (element=w1287:dbl)
              }
            }
          }
        }
      }
      frame "BüyükKafa" {
        n531 = case shown="\"Basma Gerilmesi\"" w1306 {
          tunnel: w1307 -> [_ w1312 w1509]
          tunnel: [_ w1311 w1508] -> w1305
          tunnel: [_ w1310 w1507] -> w1304
          tunnel: [_ w1309 w1506] -> w1303
          tunnel: [_ w1308 w1505] -> w1302
          frame "False", Default {
          }
          frame "Burulma Gerilmesi" {
            n532 = case shown="\"10000\"" w1312 {
              tunnel: [_ w1319 w1335 w1351 w1361 w1384 w1393 w1412 w1425 w1441 w1457 w1476 w1489] -> w1311
              tunnel: [_ w1317 w1333 w1350 w1363 w1382 w1395 w1411 w1427 w1443 w1459 w1475 w1491] -> w1310
              tunnel: [_ w1315 w1332 w1349 w1367 w1380 w1397 w1410 w1429 w1445 w1461 w1474 w1493] -> w1309
              tunnel: [_ w1313 w1331 w1348 w1365 w1378 w1399 w1409 w1431 w1447 w1463 w1473 w1495] -> w1308
              frame "False", Default {
              }
              frame "100" {
                n533 = property on="Sonuçlar" class="Arr (strict)"() -> ("Value"=w1314:dbl[][])  [unwired: 2 in, 2 out]
                n534 = property on="Sonuçlar" class="Arr (strict)"() -> ("Value"=w1316:dbl[][])  [unwired: 2 in, 2 out]
                n535 = property on="Sonuçlar" class="Arr (strict)"() -> ("Value"=w1320:dbl[][])  [unwired: 2 in, 2 out]
                n536 = property on="Sonuçlar" class="Arr (strict)"() -> ("Value"=w1318:dbl[][])  [unwired: 2 in, 2 out]
                n537 = Index Array(array=w1314, index (row)=12 ("index"), index (col)=10 ("disabled index (col)")) -> (element=w1313:dbl)
                n538 = Index Array(array=w1316, index (row)=12 ("index"), index (col)=9 ("disabled index (col)")) -> (element=w1315:dbl)
                n539 = Index Array(array=w1320, index (row)=12 ("index"), index (col)=11 ("disabled index (col)")) -> (element=w1319:dbl)
                n540 = Index Array(array=w1318, index (row)=12 ("index"), index (col)=8 ("disabled index (col)")) -> (element=w1317:dbl)
              }
              frame "500" {
                n541 = property on="Sonuçlar" class="Arr (strict)"() -> ("Value"=w1330:dbl[][])  [unwired: 2 in, 2 out]
                n542 = property on="Sonuçlar" class="Arr (strict)"() -> ("Value"=w1329:dbl[][])  [unwired: 2 in, 2 out]
                n543 = property on="Sonuçlar" class="Arr (strict)"() -> ("Value"=w1336:dbl[][])  [unwired: 2 in, 2 out]
                n544 = property on="Sonuçlar" class="Arr (strict)"() -> ("Value"=w1334:dbl[][])  [unwired: 2 in, 2 out]
                n545 = Index Array(array=w1330, index (row)=13 ("index"), index (col)=10 ("disabled index (col)")) -> (element=w1331:dbl)
                n546 = Index Array(array=w1329, index (row)=13 ("index"), index (col)=9 ("disabled index (col)")) -> (element=w1332:dbl)
                n547 = Index Array(array=w1336, index (row)=13 ("index"), index (col)=11 ("disabled index (col)")) -> (element=w1335:dbl)
                n548 = Index Array(array=w1334, index (row)=13 ("index"), index (col)=8 ("disabled index (col)")) -> (element=w1333:dbl)
              }
              frame "1000" {
                n549 = property on="Sonuçlar" class="Arr (strict)"() -> ("Value"=w1345:dbl[][])  [unwired: 2 in, 2 out]
                n550 = property on="Sonuçlar" class="Arr (strict)"() -> ("Value"=w1346:dbl[][])  [unwired: 2 in, 2 out]
                n551 = property on="Sonuçlar" class="Arr (strict)"() -> ("Value"=w1352:dbl[][])  [unwired: 2 in, 2 out]
                n552 = property on="Sonuçlar" class="Arr (strict)"() -> ("Value"=w1347:dbl[][])  [unwired: 2 in, 2 out]
                n553 = Index Array(array=w1345, index (row)=14 ("index"), index (col)=10 ("disabled index (col)")) -> (element=w1348:dbl)
                n554 = Index Array(array=w1346, index (row)=14 ("index"), index (col)=9 ("disabled index (col)")) -> (element=w1349:dbl)
                n555 = Index Array(array=w1352, index (row)=14 ("index"), index (col)=11 ("disabled index (col)")) -> (element=w1351:dbl)
                n556 = Index Array(array=w1347, index (row)=14 ("index"), index (col)=8 ("disabled index (col)")) -> (element=w1350:dbl)
              }
              frame "2000" {
                n557 = property on="Sonuçlar" class="Arr (strict)"() -> ("Value"=w1366:dbl[][])  [unwired: 2 in, 2 out]
                n558 = property on="Sonuçlar" class="Arr (strict)"() -> ("Value"=w1368:dbl[][])  [unwired: 2 in, 2 out]
                n559 = property on="Sonuçlar" class="Arr (strict)"() -> ("Value"=w1362:dbl[][])  [unwired: 2 in, 2 out]
                n560 = property on="Sonuçlar" class="Arr (strict)"() -> ("Value"=w1364:dbl[][])  [unwired: 2 in, 2 out]
                n561 = Index Array(array=w1366, index (row)=15 ("index"), index (col)=10 ("disabled index (col)")) -> (element=w1365:dbl)
                n562 = Index Array(array=w1368, index (row)=15 ("index"), index (col)=9 ("disabled index (col)")) -> (element=w1367:dbl)
                n563 = Index Array(array=w1362, index (row)=15 ("index"), index (col)=11 ("disabled index (col)")) -> (element=w1361:dbl)
                n564 = Index Array(array=w1364, index (row)=15 ("index"), index (col)=8 ("disabled index (col)")) -> (element=w1363:dbl)
              }
              frame "3000" {
                n565 = property on="Sonuçlar" class="Arr (strict)"() -> ("Value"=w1379:dbl[][])  [unwired: 2 in, 2 out]
                n566 = property on="Sonuçlar" class="Arr (strict)"() -> ("Value"=w1381:dbl[][])  [unwired: 2 in, 2 out]
                n567 = property on="Sonuçlar" class="Arr (strict)"() -> ("Value"=w1385:dbl[][])  [unwired: 2 in, 2 out]
                n568 = property on="Sonuçlar" class="Arr (strict)"() -> ("Value"=w1383:dbl[][])  [unwired: 2 in, 2 out]
                n569 = Index Array(array=w1379, index (row)=16 ("index"), index (col)=10 ("disabled index (col)")) -> (element=w1378:dbl)
                n570 = Index Array(array=w1381, index (row)=16 ("index"), index (col)=9 ("disabled index (col)")) -> (element=w1380:dbl)
                n571 = Index Array(array=w1385, index (row)=16 ("index"), index (col)=11 ("disabled index (col)")) -> (element=w1384:dbl)
                n572 = Index Array(array=w1383, index (row)=16 ("index"), index (col)=8 ("disabled index (col)")) -> (element=w1382:dbl)
              }
              frame "4000" {
                n573 = property on="Sonuçlar" class="Arr (strict)"() -> ("Value"=w1400:dbl[][])  [unwired: 2 in, 2 out]
                n574 = property on="Sonuçlar" class="Arr (strict)"() -> ("Value"=w1398:dbl[][])  [unwired: 2 in, 2 out]
                n575 = property on="Sonuçlar" class="Arr (strict)"() -> ("Value"=w1394:dbl[][])  [unwired: 2 in, 2 out]
                n576 = property on="Sonuçlar" class="Arr (strict)"() -> ("Value"=w1396:dbl[][])  [unwired: 2 in, 2 out]
                n577 = Index Array(array=w1400, index (row)=17 ("index"), index (col)=10 ("disabled index (col)")) -> (element=w1399:dbl)
                n578 = Index Array(array=w1398, index (row)=17 ("index"), index (col)=9 ("disabled index (col)")) -> (element=w1397:dbl)
                n579 = Index Array(array=w1394, index (row)=17 ("index"), index (col)=11 ("disabled index (col)")) -> (element=w1393:dbl)
                n580 = Index Array(array=w1396, index (row)=17 ("index"), index (col)=8 ("disabled index (col)")) -> (element=w1395:dbl)
              }
              frame "5000" {
                n581 = property on="Sonuçlar" class="Arr (strict)"() -> ("Value"=w1416:dbl[][])  [unwired: 2 in, 2 out]
                n582 = property on="Sonuçlar" class="Arr (strict)"() -> ("Value"=w1415:dbl[][])  [unwired: 2 in, 2 out]
                n583 = property on="Sonuçlar" class="Arr (strict)"() -> ("Value"=w1413:dbl[][])  [unwired: 2 in, 2 out]
                n584 = property on="Sonuçlar" class="Arr (strict)"() -> ("Value"=w1414:dbl[][])  [unwired: 2 in, 2 out]
                n585 = Index Array(array=w1416, index (row)=18 ("index"), index (col)=10 ("disabled index (col)")) -> (element=w1409:dbl)
                n586 = Index Array(array=w1415, index (row)=18 ("index"), index (col)=9 ("disabled index (col)")) -> (element=w1410:dbl)
                n587 = Index Array(array=w1413, index (row)=18 ("index"), index (col)=11 ("disabled index (col)")) -> (element=w1412:dbl)
                n588 = Index Array(array=w1414, index (row)=18 ("index"), index (col)=8 ("disabled index (col)")) -> (element=w1411:dbl)
              }
              frame "6000" {
                n589 = property on="Sonuçlar" class="Arr (strict)"() -> ("Value"=w1432:dbl[][])  [unwired: 2 in, 2 out]
                n590 = property on="Sonuçlar" class="Arr (strict)"() -> ("Value"=w1430:dbl[][])  [unwired: 2 in, 2 out]
                n591 = property on="Sonuçlar" class="Arr (strict)"() -> ("Value"=w1426:dbl[][])  [unwired: 2 in, 2 out]
                n592 = property on="Sonuçlar" class="Arr (strict)"() -> ("Value"=w1428:dbl[][])  [unwired: 2 in, 2 out]
                n593 = Index Array(array=w1432, index (row)=19 ("index"), index (col)=10 ("disabled index (col)")) -> (element=w1431:dbl)
                n594 = Index Array(array=w1430, index (row)=19 ("index"), index (col)=9 ("disabled index (col)")) -> (element=w1429:dbl)
                n595 = Index Array(array=w1426, index (row)=19 ("index"), index (col)=11 ("disabled index (col)")) -> (element=w1425:dbl)
                n596 = Index Array(array=w1428, index (row)=19 ("index"), index (col)=8 ("disabled index (col)")) -> (element=w1427:dbl)
              }
              frame "7000" {
                n597 = property on="Sonuçlar" class="Arr (strict)"() -> ("Value"=w1448:dbl[][])  [unwired: 2 in, 2 out]
                n598 = property on="Sonuçlar" class="Arr (strict)"() -> ("Value"=w1446:dbl[][])  [unwired: 2 in, 2 out]
                n599 = property on="Sonuçlar" class="Arr (strict)"() -> ("Value"=w1442:dbl[][])  [unwired: 2 in, 2 out]
                n600 = property on="Sonuçlar" class="Arr (strict)"() -> ("Value"=w1444:dbl[][])  [unwired: 2 in, 2 out]
                n601 = Index Array(array=w1448, index (row)=20 ("index"), index (col)=10 ("disabled index (col)")) -> (element=w1447:dbl)
                n602 = Index Array(array=w1446, index (row)=20 ("index"), index (col)=9 ("disabled index (col)")) -> (element=w1445:dbl)
                n603 = Index Array(array=w1442, index (row)=20 ("index"), index (col)=11 ("disabled index (col)")) -> (element=w1441:dbl)
                n604 = Index Array(array=w1444, index (row)=20 ("index"), index (col)=8 ("disabled index (col)")) -> (element=w1443:dbl)
              }
              frame "8000" {
                n605 = property on="Sonuçlar" class="Arr (strict)"() -> ("Value"=w1464:dbl[][])  [unwired: 2 in, 2 out]
                n606 = property on="Sonuçlar" class="Arr (strict)"() -> ("Value"=w1462:dbl[][])  [unwired: 2 in, 2 out]
                n607 = property on="Sonuçlar" class="Arr (strict)"() -> ("Value"=w1458:dbl[][])  [unwired: 2 in, 2 out]
                n608 = property on="Sonuçlar" class="Arr (strict)"() -> ("Value"=w1460:dbl[][])  [unwired: 2 in, 2 out]
                n609 = Index Array(array=w1464, index (row)=21 ("index"), index (col)=10 ("disabled index (col)")) -> (element=w1463:dbl)
                n610 = Index Array(array=w1462, index (row)=21 ("index"), index (col)=9 ("disabled index (col)")) -> (element=w1461:dbl)
                n611 = Index Array(array=w1458, index (row)=21 ("index"), index (col)=11 ("disabled index (col)")) -> (element=w1457:dbl)
                n612 = Index Array(array=w1460, index (row)=21 ("index"), index (col)=8 ("disabled index (col)")) -> (element=w1459:dbl)
              }
              frame "9000" {
                n613 = property on="Sonuçlar" class="Arr (strict)"() -> ("Value"=w1480:dbl[][])  [unwired: 2 in, 2 out]
                n614 = property on="Sonuçlar" class="Arr (strict)"() -> ("Value"=w1479:dbl[][])  [unwired: 2 in, 2 out]
                n615 = property on="Sonuçlar" class="Arr (strict)"() -> ("Value"=w1477:dbl[][])  [unwired: 2 in, 2 out]
                n616 = property on="Sonuçlar" class="Arr (strict)"() -> ("Value"=w1478:dbl[][])  [unwired: 2 in, 2 out]
                n617 = Index Array(array=w1480, index (row)=22 ("index"), index (col)=10 ("disabled index (col)")) -> (element=w1473:dbl)
                n618 = Index Array(array=w1479, index (row)=22 ("index"), index (col)=9 ("disabled index (col)")) -> (element=w1474:dbl)
                n619 = Index Array(array=w1477, index (row)=22 ("index"), index (col)=11 ("disabled index (col)")) -> (element=w1476:dbl)
                n620 = Index Array(array=w1478, index (row)=22 ("index"), index (col)=8 ("disabled index (col)")) -> (element=w1475:dbl)
              }
              frame "10000" {
                n621 = property on="Sonuçlar" class="Arr (strict)"() -> ("Value"=w1496:dbl[][])  [unwired: 2 in, 2 out]
                n622 = property on="Sonuçlar" class="Arr (strict)"() -> ("Value"=w1494:dbl[][])  [unwired: 2 in, 2 out]
                n623 = property on="Sonuçlar" class="Arr (strict)"() -> ("Value"=w1490:dbl[][])  [unwired: 2 in, 2 out]
                n624 = property on="Sonuçlar" class="Arr (strict)"() -> ("Value"=w1492:dbl[][])  [unwired: 2 in, 2 out]
                n625 = Index Array(array=w1496, index (row)=23 ("index"), index (col)=10 ("disabled index (col)")) -> (element=w1495:dbl)
                n626 = Index Array(array=w1494, index (row)=23 ("index"), index (col)=9 ("disabled index (col)")) -> (element=w1493:dbl)
                n627 = Index Array(array=w1490, index (row)=23 ("index"), index (col)=11 ("disabled index (col)")) -> (element=w1489:dbl)
                n628 = Index Array(array=w1492, index (row)=23 ("index"), index (col)=8 ("disabled index (col)")) -> (element=w1491:dbl)
              }
            }
          }
          frame "Basma Gerilmesi" {
            n629 = case shown="\"10000\"" w1509 {
              tunnel: [_ w1516 w1532 w1548 w1564 w1574 w1590 w1607 w1622 w1644 w1654 w1676 w1689] -> w1508
              tunnel: [_ w1514 w1530 w1542 w1563 w1575 w1591 w1608 w1623 w1642 w1655 w1674 w1688] -> w1507
              tunnel: [_ w1512 w1528 w1543 w1560 w1576 w1592 w1609 w1624 w1640 w1656 w1672 w1687] -> w1506
              tunnel: [_ w1511 w1526 w1544 w1558 w1577 w1593 w1610 w1625 w1638 w1657 w1670 w1686] -> w1505
              frame "False", Default {
              }
              frame "100" {
                n630 = property on="Sonuçlar" class="Arr (strict)"() -> ("Value"=w1510:dbl[][])  [unwired: 2 in, 2 out]
                n631 = property on="Sonuçlar" class="Arr (strict)"() -> ("Value"=w1517:dbl[][])  [unwired: 2 in, 2 out]
                n632 = property on="Sonuçlar" class="Arr (strict)"() -> ("Value"=w1513:dbl[][])  [unwired: 2 in, 2 out]
                n633 = property on="Sonuçlar" class="Arr (strict)"() -> ("Value"=w1515:dbl[][])  [unwired: 2 in, 2 out]
                n634 = Index Array(array=w1510, index (row)=0 ("index"), index (col)=10 ("disabled index (col)")) -> (element=w1511:dbl)
                n635 = Index Array(array=w1517, index (row)=0 ("index"), index (col)=11 ("disabled index (col)")) -> (element=w1516:dbl)
                n636 = Index Array(array=w1513, index (row)=0 ("index"), index (col)=9 ("disabled index (col)")) -> (element=w1512:dbl)
                n637 = Index Array(array=w1515, index (row)=0 ("index"), index (col)=8 ("disabled index (col)")) -> (element=w1514:dbl)
              }
              frame "500" {
                n638 = property on="Sonuçlar" class="Arr (strict)"() -> ("Value"=w1527:dbl[][])  [unwired: 2 in, 2 out]
                n639 = property on="Sonuçlar" class="Arr (strict)"() -> ("Value"=w1533:dbl[][])  [unwired: 2 in, 2 out]
                n640 = property on="Sonuçlar" class="Arr (strict)"() -> ("Value"=w1529:dbl[][])  [unwired: 2 in, 2 out]
                n641 = property on="Sonuçlar" class="Arr (strict)"() -> ("Value"=w1531:dbl[][])  [unwired: 2 in, 2 out]
                n642 = Index Array(array=w1527, index (row)=1 ("index"), index (col)=10 ("disabled index (col)")) -> (element=w1526:dbl)
                n643 = Index Array(array=w1533, index (row)=1 ("index"), index (col)=11 ("disabled index (col)")) -> (element=w1532:dbl)
                n644 = Index Array(array=w1529, index (row)=1 ("index"), index (col)=9 ("disabled index (col)")) -> (element=w1528:dbl)
                n645 = Index Array(array=w1531, index (row)=1 ("index"), index (col)=8 ("disabled index (col)")) -> (element=w1530:dbl)
              }
              frame "1000" {
                n646 = property on="Sonuçlar" class="Arr (strict)"() -> ("Value"=w1545:dbl[][])  [unwired: 2 in, 2 out]
                n647 = property on="Sonuçlar" class="Arr (strict)"() -> ("Value"=w1549:dbl[][])  [unwired: 2 in, 2 out]
                n648 = property on="Sonuçlar" class="Arr (strict)"() -> ("Value"=w1546:dbl[][])  [unwired: 2 in, 2 out]
                n649 = property on="Sonuçlar" class="Arr (strict)"() -> ("Value"=w1547:dbl[][])  [unwired: 2 in, 2 out]
                n650 = Index Array(array=w1545, index (row)=2 ("index"), index (col)=10 ("disabled index (col)")) -> (element=w1544:dbl)
                n651 = Index Array(array=w1549, index (row)=2 ("index"), index (col)=11 ("disabled index (col)")) -> (element=w1548:dbl)
                n652 = Index Array(array=w1546, index (row)=2 ("index"), index (col)=9 ("disabled index (col)")) -> (element=w1543:dbl)
                n653 = Index Array(array=w1547, index (row)=2 ("index"), index (col)=8 ("disabled index (col)")) -> (element=w1542:dbl)
              }
              frame "2000" {
                n654 = property on="Sonuçlar" class="Arr (strict)"() -> ("Value"=w1559:dbl[][])  [unwired: 2 in, 2 out]
                n655 = property on="Sonuçlar" class="Arr (strict)"() -> ("Value"=w1565:dbl[][])  [unwired: 2 in, 2 out]
                n656 = property on="Sonuçlar" class="Arr (strict)"() -> ("Value"=w1561:dbl[][])  [unwired: 2 in, 2 out]
                n657 = property on="Sonuçlar" class="Arr (strict)"() -> ("Value"=w1562:dbl[][])  [unwired: 2 in, 2 out]
                n658 = Index Array(array=w1559, index (row)=3 ("index"), index (col)=10 ("disabled index (col)")) -> (element=w1558:dbl)
                n659 = Index Array(array=w1565, index (row)=3 ("index"), index (col)=11 ("disabled index (col)")) -> (element=w1564:dbl)
                n660 = Index Array(array=w1561, index (row)=3 ("index"), index (col)=9 ("disabled index (col)")) -> (element=w1560:dbl)
                n661 = Index Array(array=w1562, index (row)=3 ("index"), index (col)=8 ("disabled index (col)")) -> (element=w1563:dbl)
              }
              frame "3000" {
                n662 = property on="Sonuçlar" class="Arr (strict)"() -> ("Value"=w1578:dbl[][])  [unwired: 2 in, 2 out]
                n663 = property on="Sonuçlar" class="Arr (strict)"() -> ("Value"=w1581:dbl[][])  [unwired: 2 in, 2 out]
                n664 = property on="Sonuçlar" class="Arr (strict)"() -> ("Value"=w1579:dbl[][])  [unwired: 2 in, 2 out]
                n665 = property on="Sonuçlar" class="Arr (strict)"() -> ("Value"=w1580:dbl[][])  [unwired: 2 in, 2 out]
                n666 = Index Array(array=w1578, index (row)=4 ("index"), index (col)=10 ("disabled index (col)")) -> (element=w1577:dbl)
                n667 = Index Array(array=w1581, index (row)=4 ("index"), index (col)=11 ("disabled index (col)")) -> (element=w1574:dbl)
                n668 = Index Array(array=w1579, index (row)=4 ("index"), index (col)=9 ("disabled index (col)")) -> (element=w1576:dbl)
                n669 = Index Array(array=w1580, index (row)=4 ("index"), index (col)=8 ("disabled index (col)")) -> (element=w1575:dbl)
              }
              frame "4000" {
                n670 = property on="Sonuçlar" class="Arr (strict)"() -> ("Value"=w1594:dbl[][])  [unwired: 2 in, 2 out]
                n671 = property on="Sonuçlar" class="Arr (strict)"() -> ("Value"=w1597:dbl[][])  [unwired: 2 in, 2 out]
                n672 = property on="Sonuçlar" class="Arr (strict)"() -> ("Value"=w1595:dbl[][])  [unwired: 2 in, 2 out]
                n673 = property on="Sonuçlar" class="Arr (strict)"() -> ("Value"=w1596:dbl[][])  [unwired: 2 in, 2 out]
                n674 = Index Array(array=w1594, index (row)=5 ("index"), index (col)=10 ("disabled index (col)")) -> (element=w1593:dbl)
                n675 = Index Array(array=w1597, index (row)=5 ("index"), index (col)=11 ("disabled index (col)")) -> (element=w1590:dbl)
                n676 = Index Array(array=w1595, index (row)=5 ("index"), index (col)=9 ("disabled index (col)")) -> (element=w1592:dbl)
                n677 = Index Array(array=w1596, index (row)=5 ("index"), index (col)=8 ("disabled index (col)")) -> (element=w1591:dbl)
              }
              frame "5000" {
                n678 = property on="Sonuçlar" class="Arr (strict)"() -> ("Value"=w1611:dbl[][])  [unwired: 2 in, 2 out]
                n679 = property on="Sonuçlar" class="Arr (strict)"() -> ("Value"=w1614:dbl[][])  [unwired: 2 in, 2 out]
                n680 = property on="Sonuçlar" class="Arr (strict)"() -> ("Value"=w1612:dbl[][])  [unwired: 2 in, 2 out]
                n681 = property on="Sonuçlar" class="Arr (strict)"() -> ("Value"=w1613:dbl[][])  [unwired: 2 in, 2 out]
                n682 = Index Array(array=w1611, index (row)=6 ("index"), index (col)=10 ("disabled index (col)")) -> (element=w1610:dbl)
                n683 = Index Array(array=w1614, index (row)=6 ("index"), index (col)=10 ("disabled index (col)")) -> (element=w1607:dbl)
                n684 = Index Array(array=w1612, index (row)=6 ("index"), index (col)=9 ("disabled index (col)")) -> (element=w1609:dbl)
                n685 = Index Array(array=w1613, index (row)=6 ("index"), index (col)=8 ("disabled index (col)")) -> (element=w1608:dbl)
              }
              frame "6000" {
                n686 = property on="Sonuçlar" class="Arr (strict)"() -> ("Value"=w1626:dbl[][])  [unwired: 2 in, 2 out]
                n687 = property on="Sonuçlar" class="Arr (strict)"() -> ("Value"=w1629:dbl[][])  [unwired: 2 in, 2 out]
                n688 = property on="Sonuçlar" class="Arr (strict)"() -> ("Value"=w1627:dbl[][])  [unwired: 2 in, 2 out]
                n689 = property on="Sonuçlar" class="Arr (strict)"() -> ("Value"=w1628:dbl[][])  [unwired: 2 in, 2 out]
                n690 = Index Array(array=w1626, index (row)=7 ("index"), index (col)=10 ("disabled index (col)")) -> (element=w1625:dbl)
                n691 = Index Array(array=w1629, index (row)=7 ("index"), index (col)=11 ("disabled index (col)")) -> (element=w1622:dbl)
                n692 = Index Array(array=w1627, index (row)=7 ("index"), index (col)=9 ("disabled index (col)")) -> (element=w1624:dbl)
                n693 = Index Array(array=w1628, index (row)=7 ("index"), index (col)=8 ("disabled index (col)")) -> (element=w1623:dbl)
              }
              frame "7000" {
                n694 = property on="Sonuçlar" class="Arr (strict)"() -> ("Value"=w1639:dbl[][])  [unwired: 2 in, 2 out]
                n695 = property on="Sonuçlar" class="Arr (strict)"() -> ("Value"=w1645:dbl[][])  [unwired: 2 in, 2 out]
                n696 = property on="Sonuçlar" class="Arr (strict)"() -> ("Value"=w1641:dbl[][])  [unwired: 2 in, 2 out]
                n697 = property on="Sonuçlar" class="Arr (strict)"() -> ("Value"=w1643:dbl[][])  [unwired: 2 in, 2 out]
                n698 = Index Array(array=w1639, index (row)=8 ("index"), index (col)=10 ("disabled index (col)")) -> (element=w1638:dbl)
                n699 = Index Array(array=w1645, index (row)=8 ("index"), index (col)=11 ("disabled index (col)")) -> (element=w1644:dbl)
                n700 = Index Array(array=w1641, index (row)=8 ("index"), index (col)=9 ("disabled index (col)")) -> (element=w1640:dbl)
                n701 = Index Array(array=w1643, index (row)=8 ("index"), index (col)=8 ("disabled index (col)")) -> (element=w1642:dbl)
              }
              frame "8000" {
                n702 = property on="Sonuçlar" class="Arr (strict)"() -> ("Value"=w1658:dbl[][])  [unwired: 2 in, 2 out]
                n703 = property on="Sonuçlar" class="Arr (strict)"() -> ("Value"=w1661:dbl[][])  [unwired: 2 in, 2 out]
                n704 = property on="Sonuçlar" class="Arr (strict)"() -> ("Value"=w1659:dbl[][])  [unwired: 2 in, 2 out]
                n705 = property on="Sonuçlar" class="Arr (strict)"() -> ("Value"=w1660:dbl[][])  [unwired: 2 in, 2 out]
                n706 = Index Array(array=w1658, index (row)=9 ("index"), index (col)=10 ("disabled index (col)")) -> (element=w1657:dbl)
                n707 = Index Array(array=w1661, index (row)=9 ("index"), index (col)=11 ("disabled index (col)")) -> (element=w1654:dbl)
                n708 = Index Array(array=w1659, index (row)=9 ("index"), index (col)=9 ("disabled index (col)")) -> (element=w1656:dbl)
                n709 = Index Array(array=w1660, index (row)=9 ("index"), index (col)=8 ("disabled index (col)")) -> (element=w1655:dbl)
              }
              frame "9000" {
                n710 = property on="Sonuçlar" class="Arr (strict)"() -> ("Value"=w1671:dbl[][])  [unwired: 2 in, 2 out]
                n711 = property on="Sonuçlar" class="Arr (strict)"() -> ("Value"=w1673:dbl[][])  [unwired: 2 in, 2 out]
                n712 = property on="Sonuçlar" class="Arr (strict)"() -> ("Value"=w1677:dbl[][])  [unwired: 2 in, 2 out]
                n713 = property on="Sonuçlar" class="Arr (strict)"() -> ("Value"=w1675:dbl[][])  [unwired: 2 in, 2 out]
                n714 = Index Array(array=w1671, index (row)=10 ("index"), index (col)=10 ("disabled index (col)")) -> (element=w1670:dbl)
                n715 = Index Array(array=w1673, index (row)=10 ("index"), index (col)=9 ("disabled index (col)")) -> (element=w1672:dbl)
                n716 = Index Array(array=w1677, index (row)=10 ("index"), index (col)=11 ("disabled index (col)")) -> (element=w1676:dbl)
                n717 = Index Array(array=w1675, index (row)=10 ("index"), index (col)=8 ("disabled index (col)")) -> (element=w1674:dbl)
              }
              frame "10000" {
                n718 = property on="Sonuçlar" class="Arr (strict)"() -> ("Value"=w1693:dbl[][])  [unwired: 2 in, 2 out]
                n719 = property on="Sonuçlar" class="Arr (strict)"() -> ("Value"=w1692:dbl[][])  [unwired: 2 in, 2 out]
                n720 = property on="Sonuçlar" class="Arr (strict)"() -> ("Value"=w1690:dbl[][])  [unwired: 2 in, 2 out]
                n721 = property on="Sonuçlar" class="Arr (strict)"() -> ("Value"=w1691:dbl[][])  [unwired: 2 in, 2 out]
                n722 = Index Array(array=w1693, index (row)=11 ("index"), index (col)=10 ("disabled index (col)")) -> (element=w1686:dbl)
                n723 = Index Array(array=w1692, index (row)=11 ("index"), index (col)=9 ("disabled index (col)")) -> (element=w1687:dbl)
                n724 = Index Array(array=w1690, index (row)=11 ("index"), index (col)=10 ("disabled index (col)")) -> (element=w1689:dbl)
                n725 = Index Array(array=w1691, index (row)=11 ("index"), index (col)=8 ("disabled index (col)")) -> (element=w1688:dbl)
              }
            }
          }
        }
      }
      frame "KüçükKafa" {
        n726 = case shown="\"Basma Gerilmesi\"" w1706 {
          tunnel: w1707 -> [_ w1712 w1909]
          tunnel: [_ w1708 w1908] -> w1705
          tunnel: [_ w1709 w1907] -> w1704
          tunnel: [_ w1710 w1906] -> w1703
          tunnel: [_ w1711 w1905] -> w1702
          frame "False", Default {
          }
          frame "Burulma Gerilmesi" {
            n727 = case shown="\"10000\"" w1712 {
              tunnel: [_ w1719 w1735 w1751 w1767 w1783 w1799 w1815 w1831 w1847 w1863 w1879 w1895] -> w1711
              tunnel: [_ w1717 w1733 w1749 w1765 w1781 w1797 w1813 w1829 w1845 w1861 w1873 w1893] -> w1710
              tunnel: [_ w1715 w1731 w1747 w1763 w1779 w1795 w1811 w1827 w1843 w1859 w1874 w1891] -> w1709
              tunnel: [_ w1713 w1729 w1745 w1761 w1777 w1793 w1809 w1825 w1841 w1857 w1875 w1889] -> w1708
              frame "False", Default {
              }
              frame "100" {
                n728 = property on="Sonuçlar" class="Arr (strict)"() -> ("Value"=w1720:dbl[][])  [unwired: 2 in, 2 out]
                n729 = property on="Sonuçlar" class="Arr (strict)"() -> ("Value"=w1718:dbl[][])  [unwired: 2 in, 2 out]
                n730 = property on="Sonuçlar" class="Arr (strict)"() -> ("Value"=w1716:dbl[][])  [unwired: 2 in, 2 out]
                n731 = property on="Sonuçlar" class="Arr (strict)"() -> ("Value"=w1714:dbl[][])  [unwired: 2 in, 2 out]
                n732 = Index Array(array=w1720, index (row)=12 ("index"), index (col)=13 ("disabled index (col)")) -> (element=w1719:dbl)
                n733 = Index Array(array=w1718, index (row)=12 ("index"), index (col)=14 ("disabled index (col)")) -> (element=w1717:dbl)
                n734 = Index Array(array=w1716, index (row)=12 ("index"), index (col)=15 ("disabled index (col)")) -> (element=w1715:dbl)
                n735 = Index Array(array=w1714, index (row)=12 ("index"), index (col)=12 ("disabled index (col)")) -> (element=w1713:dbl)
              }
              frame "500" {
                n736 = property on="Sonuçlar" class="Arr (strict)"() -> ("Value"=w1736:dbl[][])  [unwired: 2 in, 2 out]
                n737 = property on="Sonuçlar" class="Arr (strict)"() -> ("Value"=w1734:dbl[][])  [unwired: 2 in, 2 out]
                n738 = property on="Sonuçlar" class="Arr (strict)"() -> ("Value"=w1732:dbl[][])  [unwired: 2 in, 2 out]
                n739 = property on="Sonuçlar" class="Arr (strict)"() -> ("Value"=w1730:dbl[][])  [unwired: 2 in, 2 out]
                n740 = Index Array(array=w1736, index (row)=13 ("index"), index (col)=14 ("disabled index (col)")) -> (element=w1735:dbl)
                n741 = Index Array(array=w1734, index (row)=13 ("index"), index (col)=13 ("disabled index (col)")) -> (element=w1733:dbl)
                n742 = Index Array(array=w1732, index (row)=13 ("index"), index (col)=15 ("disabled index (col)")) -> (element=w1731:dbl)
                n743 = Index Array(array=w1730, index (row)=13 ("index"), index (col)=12 ("disabled index (col)")) -> (element=w1729:dbl)
              }
              frame "1000" {
                n744 = property on="Sonuçlar" class="Arr (strict)"() -> ("Value"=w1752:dbl[][])  [unwired: 2 in, 2 out]
                n745 = property on="Sonuçlar" class="Arr (strict)"() -> ("Value"=w1750:dbl[][])  [unwired: 2 in, 2 out]
                n746 = property on="Sonuçlar" class="Arr (strict)"() -> ("Value"=w1748:dbl[][])  [unwired: 2 in, 2 out]
                n747 = property on="Sonuçlar" class="Arr (strict)"() -> ("Value"=w1746:dbl[][])  [unwired: 2 in, 2 out]
                n748 = Index Array(array=w1752, index (row)=14 ("index"), index (col)=14 ("disabled index (col)")) -> (element=w1751:dbl)
                n749 = Index Array(array=w1750, index (row)=14 ("index"), index (col)=13 ("disabled index (col)")) -> (element=w1749:dbl)
                n750 = Index Array(array=w1748, index (row)=14 ("index"), index (col)=15 ("disabled index (col)")) -> (element=w1747:dbl)
                n751 = Index Array(array=w1746, index (row)=14 ("index"), index (col)=12 ("disabled index (col)")) -> (element=w1745:dbl)
              }
              frame "2000" {
                n752 = property on="Sonuçlar" class="Arr (strict)"() -> ("Value"=w1768:dbl[][])  [unwired: 2 in, 2 out]
                n753 = property on="Sonuçlar" class="Arr (strict)"() -> ("Value"=w1766:dbl[][])  [unwired: 2 in, 2 out]
                n754 = property on="Sonuçlar" class="Arr (strict)"() -> ("Value"=w1764:dbl[][])  [unwired: 2 in, 2 out]
                n755 = property on="Sonuçlar" class="Arr (strict)"() -> ("Value"=w1762:dbl[][])  [unwired: 2 in, 2 out]
                n756 = Index Array(array=w1768, index (row)=15 ("index"), index (col)=14 ("disabled index (col)")) -> (element=w1767:dbl)
                n757 = Index Array(array=w1766, index (row)=15 ("index"), index (col)=13 ("disabled index (col)")) -> (element=w1765:dbl)
                n758 = Index Array(array=w1764, index (row)=15 ("index"), index (col)=15 ("disabled index (col)")) -> (element=w1763:dbl)
                n759 = Index Array(array=w1762, index (row)=15 ("index"), index (col)=12 ("disabled index (col)")) -> (element=w1761:dbl)
              }
              frame "3000" {
                n760 = property on="Sonuçlar" class="Arr (strict)"() -> ("Value"=w1784:dbl[][])  [unwired: 2 in, 2 out]
                n761 = property on="Sonuçlar" class="Arr (strict)"() -> ("Value"=w1782:dbl[][])  [unwired: 2 in, 2 out]
                n762 = property on="Sonuçlar" class="Arr (strict)"() -> ("Value"=w1780:dbl[][])  [unwired: 2 in, 2 out]
                n763 = property on="Sonuçlar" class="Arr (strict)"() -> ("Value"=w1778:dbl[][])  [unwired: 2 in, 2 out]
                n764 = Index Array(array=w1784, index (row)=16 ("index"), index (col)=14 ("disabled index (col)")) -> (element=w1783:dbl)
                n765 = Index Array(array=w1782, index (row)=16 ("index"), index (col)=13 ("disabled index (col)")) -> (element=w1781:dbl)
                n766 = Index Array(array=w1780, index (row)=16 ("index"), index (col)=15 ("disabled index (col)")) -> (element=w1779:dbl)
                n767 = Index Array(array=w1778, index (row)=16 ("index"), index (col)=12 ("disabled index (col)")) -> (element=w1777:dbl)
              }
              frame "4000" {
                n768 = property on="Sonuçlar" class="Arr (strict)"() -> ("Value"=w1800:dbl[][])  [unwired: 2 in, 2 out]
                n769 = property on="Sonuçlar" class="Arr (strict)"() -> ("Value"=w1798:dbl[][])  [unwired: 2 in, 2 out]
                n770 = property on="Sonuçlar" class="Arr (strict)"() -> ("Value"=w1796:dbl[][])  [unwired: 2 in, 2 out]
                n771 = property on="Sonuçlar" class="Arr (strict)"() -> ("Value"=w1794:dbl[][])  [unwired: 2 in, 2 out]
                n772 = Index Array(array=w1800, index (row)=17 ("index"), index (col)=14 ("disabled index (col)")) -> (element=w1799:dbl)
                n773 = Index Array(array=w1798, index (row)=17 ("index"), index (col)=13 ("disabled index (col)")) -> (element=w1797:dbl)
                n774 = Index Array(array=w1796, index (row)=17 ("index"), index (col)=15 ("disabled index (col)")) -> (element=w1795:dbl)
                n775 = Index Array(array=w1794, index (row)=17 ("index"), index (col)=12 ("disabled index (col)")) -> (element=w1793:dbl)
              }
              frame "5000" {
                n776 = property on="Sonuçlar" class="Arr (strict)"() -> ("Value"=w1816:dbl[][])  [unwired: 2 in, 2 out]
                n777 = property on="Sonuçlar" class="Arr (strict)"() -> ("Value"=w1814:dbl[][])  [unwired: 2 in, 2 out]
                n778 = property on="Sonuçlar" class="Arr (strict)"() -> ("Value"=w1812:dbl[][])  [unwired: 2 in, 2 out]
                n779 = property on="Sonuçlar" class="Arr (strict)"() -> ("Value"=w1810:dbl[][])  [unwired: 2 in, 2 out]
                n780 = Index Array(array=w1816, index (row)=18 ("index"), index (col)=14 ("disabled index (col)")) -> (element=w1815:dbl)
                n781 = Index Array(array=w1814, index (row)=18 ("index"), index (col)=13 ("disabled index (col)")) -> (element=w1813:dbl)
                n782 = Index Array(array=w1812, index (row)=18 ("index"), index (col)=15 ("disabled index (col)")) -> (element=w1811:dbl)
                n783 = Index Array(array=w1810, index (row)=18 ("index"), index (col)=12 ("disabled index (col)")) -> (element=w1809:dbl)
              }
              frame "6000" {
                n784 = property on="Sonuçlar" class="Arr (strict)"() -> ("Value"=w1832:dbl[][])  [unwired: 2 in, 2 out]
                n785 = property on="Sonuçlar" class="Arr (strict)"() -> ("Value"=w1830:dbl[][])  [unwired: 2 in, 2 out]
                n786 = property on="Sonuçlar" class="Arr (strict)"() -> ("Value"=w1828:dbl[][])  [unwired: 2 in, 2 out]
                n787 = property on="Sonuçlar" class="Arr (strict)"() -> ("Value"=w1826:dbl[][])  [unwired: 2 in, 2 out]
                n788 = Index Array(array=w1832, index (row)=19 ("index"), index (col)=14 ("disabled index (col)")) -> (element=w1831:dbl)
                n789 = Index Array(array=w1830, index (row)=19 ("index"), index (col)=13 ("disabled index (col)")) -> (element=w1829:dbl)
                n790 = Index Array(array=w1828, index (row)=19 ("index"), index (col)=15 ("disabled index (col)")) -> (element=w1827:dbl)
                n791 = Index Array(array=w1826, index (row)=19 ("index"), index (col)=12 ("disabled index (col)")) -> (element=w1825:dbl)
              }
              frame "7000" {
                n792 = property on="Sonuçlar" class="Arr (strict)"() -> ("Value"=w1848:dbl[][])  [unwired: 2 in, 2 out]
                n793 = property on="Sonuçlar" class="Arr (strict)"() -> ("Value"=w1846:dbl[][])  [unwired: 2 in, 2 out]
                n794 = property on="Sonuçlar" class="Arr (strict)"() -> ("Value"=w1844:dbl[][])  [unwired: 2 in, 2 out]
                n795 = property on="Sonuçlar" class="Arr (strict)"() -> ("Value"=w1842:dbl[][])  [unwired: 2 in, 2 out]
                n796 = Index Array(array=w1848, index (row)=20 ("index"), index (col)=14 ("disabled index (col)")) -> (element=w1847:dbl)
                n797 = Index Array(array=w1846, index (row)=20 ("index"), index (col)=13 ("disabled index (col)")) -> (element=w1845:dbl)
                n798 = Index Array(array=w1844, index (row)=20 ("index"), index (col)=15 ("disabled index (col)")) -> (element=w1843:dbl)
                n799 = Index Array(array=w1842, index (row)=20 ("index"), index (col)=12 ("disabled index (col)")) -> (element=w1841:dbl)
              }
              frame "8000" {
                n800 = property on="Sonuçlar" class="Arr (strict)"() -> ("Value"=w1864:dbl[][])  [unwired: 2 in, 2 out]
                n801 = property on="Sonuçlar" class="Arr (strict)"() -> ("Value"=w1862:dbl[][])  [unwired: 2 in, 2 out]
                n802 = property on="Sonuçlar" class="Arr (strict)"() -> ("Value"=w1860:dbl[][])  [unwired: 2 in, 2 out]
                n803 = property on="Sonuçlar" class="Arr (strict)"() -> ("Value"=w1858:dbl[][])  [unwired: 2 in, 2 out]
                n804 = Index Array(array=w1864, index (row)=21 ("index"), index (col)=14 ("disabled index (col)")) -> (element=w1863:dbl)
                n805 = Index Array(array=w1862, index (row)=21 ("index"), index (col)=13 ("disabled index (col)")) -> (element=w1861:dbl)
                n806 = Index Array(array=w1860, index (row)=21 ("index"), index (col)=15 ("disabled index (col)")) -> (element=w1859:dbl)
                n807 = Index Array(array=w1858, index (row)=21 ("index"), index (col)=12 ("disabled index (col)")) -> (element=w1857:dbl)
              }
              frame "9000" {
                n808 = property on="Sonuçlar" class="Arr (strict)"() -> ("Value"=w1880:dbl[][])  [unwired: 2 in, 2 out]
                n809 = property on="Sonuçlar" class="Arr (strict)"() -> ("Value"=w1878:dbl[][])  [unwired: 2 in, 2 out]
                n810 = property on="Sonuçlar" class="Arr (strict)"() -> ("Value"=w1877:dbl[][])  [unwired: 2 in, 2 out]
                n811 = property on="Sonuçlar" class="Arr (strict)"() -> ("Value"=w1876:dbl[][])  [unwired: 2 in, 2 out]
                n812 = Index Array(array=w1880, index (row)=22 ("index"), index (col)=14 ("disabled index (col)")) -> (element=w1879:dbl)
                n813 = Index Array(array=w1878, index (row)=22 ("index"), index (col)=13 ("disabled index (col)")) -> (element=w1873:dbl)
                n814 = Index Array(array=w1877, index (row)=22 ("index"), index (col)=15 ("disabled index (col)")) -> (element=w1874:dbl)
                n815 = Index Array(array=w1876, index (row)=22 ("index"), index (col)=12 ("disabled index (col)")) -> (element=w1875:dbl)
              }
              frame "10000" {
                n816 = property on="Sonuçlar" class="Arr (strict)"() -> ("Value"=w1896:dbl[][])  [unwired: 2 in, 2 out]
                n817 = property on="Sonuçlar" class="Arr (strict)"() -> ("Value"=w1894:dbl[][])  [unwired: 2 in, 2 out]
                n818 = property on="Sonuçlar" class="Arr (strict)"() -> ("Value"=w1892:dbl[][])  [unwired: 2 in, 2 out]
                n819 = property on="Sonuçlar" class="Arr (strict)"() -> ("Value"=w1890:dbl[][])  [unwired: 2 in, 2 out]
                n820 = Index Array(array=w1896, index (row)=23 ("index"), index (col)=14 ("disabled index (col)")) -> (element=w1895:dbl)
                n821 = Index Array(array=w1894, index (row)=23 ("index"), index (col)=13 ("disabled index (col)")) -> (element=w1893:dbl)
                n822 = Index Array(array=w1892, index (row)=23 ("index"), index (col)=15 ("disabled index (col)")) -> (element=w1891:dbl)
                n823 = Index Array(array=w1890, index (row)=23 ("index"), index (col)=12 ("disabled index (col)")) -> (element=w1889:dbl)
              }
            }
          }
          frame "Basma Gerilmesi" {
            n824 = case shown="\"100\"" w1909 {
              tunnel: [_ w1922 w1926 w1942 w1958 w1974 w1993 w2008 w2023 w2041 w2055 w2070 w2086] -> w1908
              tunnel: [_ w1923 w1928 w1944 w1960 w1976 w1992 w2007 w2024 w2040 w2056 w2072 w2092] -> w1907
              tunnel: [_ w1924 w1930 w1947 w1962 w1978 w1991 w2006 w2027 w2039 w2059 w2075 w2090] -> w1906
              tunnel: [_ w1925 w1932 w1948 w1964 w1980 w1990 w2012 w2028 w2038 w2060 w2076 w2088] -> w1905
              frame "False", Default {
              }
              frame "100" {
                n825 = property on="Sonuçlar" class="Arr (strict)"() -> ("Value"=w1913:dbl[][])  [unwired: 2 in, 2 out]
                n826 = property on="Sonuçlar" class="Arr (strict)"() -> ("Value"=w1912:dbl[][])  [unwired: 2 in, 2 out]
                n827 = property on="Sonuçlar" class="Arr (strict)"() -> ("Value"=w1911:dbl[][])  [unwired: 2 in, 2 out]
                n828 = property on="Sonuçlar" class="Arr (strict)"() -> ("Value"=w1910:dbl[][])  [unwired: 2 in, 2 out]
                n829 = Index Array(array=w1913, index (row)=0 ("index"), index (col)=14 ("disabled index (col)")) -> (element=w1925:dbl)
                n830 = Index Array(array=w1912, index (row)=0 ("index"), index (col)=13 ("disabled index (col)")) -> (element=w1924:dbl)
                n831 = Index Array(array=w1911, index (row)=0 ("index"), index (col)=15 ("disabled index (col)")) -> (element=w1923:dbl)
                n832 = Index Array(array=w1910, index (row)=0 ("index"), index (col)=12 ("disabled index (col)")) -> (element=w1922:dbl)
              }
              frame "500" {
                n833 = property on="Sonuçlar" class="Arr (strict)"() -> ("Value"=w1933:dbl[][])  [unwired: 2 in, 2 out]
                n834 = property on="Sonuçlar" class="Arr (strict)"() -> ("Value"=w1931:dbl[][])  [unwired: 2 in, 2 out]
                n835 = property on="Sonuçlar" class="Arr (strict)"() -> ("Value"=w1929:dbl[][])  [unwired: 2 in, 2 out]
                n836 = property on="Sonuçlar" class="Arr (strict)"() -> ("Value"=w1927:dbl[][])  [unwired: 2 in, 2 out]
                n837 = Index Array(array=w1933, index (row)=1 ("index"), index (col)=14 ("disabled index (col)")) -> (element=w1932:dbl)
                n838 = Index Array(array=w1931, index (row)=1 ("index"), index (col)=13 ("disabled index (col)")) -> (element=w1930:dbl)
                n839 = Index Array(array=w1929, index (row)=1 ("index"), index (col)=15 ("disabled index (col)")) -> (element=w1928:dbl)
                n840 = Index Array(array=w1927, index (row)=1 ("index"), index (col)=12 ("disabled index (col)")) -> (element=w1926:dbl)
              }
              frame "1000" {
                n841 = property on="Sonuçlar" class="Arr (strict)"() -> ("Value"=w1949:dbl[][])  [unwired: 2 in, 2 out]
                n842 = property on="Sonuçlar" class="Arr (strict)"() -> ("Value"=w1946:dbl[][])  [unwired: 2 in, 2 out]
                n843 = property on="Sonuçlar" class="Arr (strict)"() -> ("Value"=w1945:dbl[][])  [unwired: 2 in, 2 out]
                n844 = property on="Sonuçlar" class="Arr (strict)"() -> ("Value"=w1943:dbl[][])  [unwired: 2 in, 2 out]
                n845 = Index Array(array=w1949, index (row)=2 ("index"), index (col)=14 ("disabled index (col)")) -> (element=w1948:dbl)
                n846 = Index Array(array=w1946, index (row)=2 ("index"), index (col)=13 ("disabled index (col)")) -> (element=w1947:dbl)
                n847 = Index Array(array=w1945, index (row)=2 ("index"), index (col)=15 ("disabled index (col)")) -> (element=w1944:dbl)
                n848 = Index Array(array=w1943, index (row)=2 ("index"), index (col)=12 ("disabled index (col)")) -> (element=w1942:dbl)
              }
              frame "2000" {
                n849 = property on="Sonuçlar" class="Arr (strict)"() -> ("Value"=w1965:dbl[][])  [unwired: 2 in, 2 out]
                n850 = property on="Sonuçlar" class="Arr (strict)"() -> ("Value"=w1963:dbl[][])  [unwired: 2 in, 2 out]
                n851 = property on="Sonuçlar" class="Arr (strict)"() -> ("Value"=w1961:dbl[][])  [unwired: 2 in, 2 out]
                n852 = property on="Sonuçlar" class="Arr (strict)"() -> ("Value"=w1959:dbl[][])  [unwired: 2 in, 2 out]
                n853 = Index Array(array=w1965, index (row)=3 ("index"), index (col)=14 ("disabled index (col)")) -> (element=w1964:dbl)
                n854 = Index Array(array=w1963, index (row)=3 ("index"), index (col)=13 ("disabled index (col)")) -> (element=w1962:dbl)
                n855 = Index Array(array=w1961, index (row)=3 ("index"), index (col)=15 ("disabled index (col)")) -> (element=w1960:dbl)
                n856 = Index Array(array=w1959, index (row)=3 ("index"), index (col)=12 ("disabled index (col)")) -> (element=w1958:dbl)
              }
              frame "3000" {
                n857 = property on="Sonuçlar" class="Arr (strict)"() -> ("Value"=w1981:dbl[][])  [unwired: 2 in, 2 out]
                n858 = property on="Sonuçlar" class="Arr (strict)"() -> ("Value"=w1979:dbl[][])  [unwired: 2 in, 2 out]
                n859 = property on="Sonuçlar" class="Arr (strict)"() -> ("Value"=w1977:dbl[][])  [unwired: 2 in, 2 out]
                n860 = property on="Sonuçlar" class="Arr (strict)"() -> ("Value"=w1975:dbl[][])  [unwired: 2 in, 2 out]
                n861 = Index Array(array=w1981, index (row)=4 ("index"), index (col)=14 ("disabled index (col)")) -> (element=w1980:dbl)
                n862 = Index Array(array=w1979, index (row)=4 ("index"), index (col)=13 ("disabled index (col)")) -> (element=w1978:dbl)
                n863 = Index Array(array=w1977, index (row)=4 ("index"), index (col)=15 ("disabled index (col)")) -> (element=w1976:dbl)
                n864 = Index Array(array=w1975, index (row)=4 ("index"), index (col)=12 ("disabled index (col)")) -> (element=w1974:dbl)
              }
              frame "4000" {
                n865 = property on="Sonuçlar" class="Arr (strict)"() -> ("Value"=w1997:dbl[][])  [unwired: 2 in, 2 out]
                n866 = property on="Sonuçlar" class="Arr (strict)"() -> ("Value"=w1996:dbl[][])  [unwired: 2 in, 2 out]
                n867 = property on="Sonuçlar" class="Arr (strict)"() -> ("Value"=w1995:dbl[][])  [unwired: 2 in, 2 out]
                n868 = property on="Sonuçlar" class="Arr (strict)"() -> ("Value"=w1994:dbl[][])  [unwired: 2 in, 2 out]
                n869 = Index Array(array=w1997, index (row)=5 ("index"), index (col)=14 ("disabled index (col)")) -> (element=w1990:dbl)
                n870 = Index Array(array=w1996, index (row)=5 ("index"), index (col)=13 ("disabled index (col)")) -> (element=w1991:dbl)
                n871 = Index Array(array=w1995, index (row)=5 ("index"), index (col)=15 ("disabled index (col)")) -> (element=w1992:dbl)
                n872 = Index Array(array=w1994, index (row)=5 ("index"), index (col)=12 ("disabled index (col)")) -> (element=w1993:dbl)
              }
              frame "5000" {
                n873 = property on="Sonuçlar" class="Arr (strict)"() -> ("Value"=w2013:dbl[][])  [unwired: 2 in, 2 out]
                n874 = property on="Sonuçlar" class="Arr (strict)"() -> ("Value"=w2011:dbl[][])  [unwired: 2 in, 2 out]
                n875 = property on="Sonuçlar" class="Arr (strict)"() -> ("Value"=w2010:dbl[][])  [unwired: 2 in, 2 out]
                n876 = property on="Sonuçlar" class="Arr (strict)"() -> ("Value"=w2009:dbl[][])  [unwired: 2 in, 2 out]
                n877 = Index Array(array=w2013, index (row)=6 ("index"), index (col)=14 ("disabled index (col)")) -> (element=w2012:dbl)
                n878 = Index Array(array=w2011, index (row)=6 ("index"), index (col)=13 ("disabled index (col)")) -> (element=w2006:dbl)
                n879 = Index Array(array=w2010, index (row)=6 ("index"), index (col)=15 ("disabled index (col)")) -> (element=w2007:dbl)
                n880 = Index Array(array=w2009, index (row)=6 ("index"), index (col)=12 ("disabled index (col)")) -> (element=w2008:dbl)
              }
              frame "6000" {
                n881 = property on="Sonuçlar" class="Arr (strict)"() -> ("Value"=w2029:dbl[][])  [unwired: 2 in, 2 out]
                n882 = property on="Sonuçlar" class="Arr (strict)"() -> ("Value"=w2026:dbl[][])  [unwired: 2 in, 2 out]
                n883 = property on="Sonuçlar" class="Arr (strict)"() -> ("Value"=w2025:dbl[][])  [unwired: 2 in, 2 out]
                n884 = property on="Sonuçlar" class="Arr (strict)"() -> ("Value"=w2022:dbl[][])  [unwired: 2 in, 2 out]
                n885 = Index Array(array=w2029, index (row)=7 ("index"), index (col)=14 ("disabled index (col)")) -> (element=w2028:dbl)
                n886 = Index Array(array=w2026, index (row)=7 ("index"), index (col)=13 ("disabled index (col)")) -> (element=w2027:dbl)
                n887 = Index Array(array=w2025, index (row)=7 ("index"), index (col)=15 ("disabled index (col)")) -> (element=w2024:dbl)
                n888 = Index Array(array=w2022, index (row)=7 ("index"), index (col)=12 ("disabled index (col)")) -> (element=w2023:dbl)
              }
              frame "7000" {
                n889 = property on="Sonuçlar" class="Arr (strict)"() -> ("Value"=w2045:dbl[][])  [unwired: 2 in, 2 out]
                n890 = property on="Sonuçlar" class="Arr (strict)"() -> ("Value"=w2044:dbl[][])  [unwired: 2 in, 2 out]
                n891 = property on="Sonuçlar" class="Arr (strict)"() -> ("Value"=w2043:dbl[][])  [unwired: 2 in, 2 out]
                n892 = property on="Sonuçlar" class="Arr (strict)"() -> ("Value"=w2042:dbl[][])  [unwired: 2 in, 2 out]
                n893 = Index Array(array=w2045, index (row)=8 ("index"), index (col)=14 ("disabled index (col)")) -> (element=w2038:dbl)
                n894 = Index Array(array=w2044, index (row)=8 ("index"), index (col)=13 ("disabled index (col)")) -> (element=w2039:dbl)
                n895 = Index Array(array=w2043, index (row)=8 ("index"), index (col)=15 ("disabled index (col)")) -> (element=w2040:dbl)
                n896 = Index Array(array=w2042, index (row)=8 ("index"), index (col)=12 ("disabled index (col)")) -> (element=w2041:dbl)
              }
              frame "8000" {
                n897 = property on="Sonuçlar" class="Arr (strict)"() -> ("Value"=w2061:dbl[][])  [unwired: 2 in, 2 out]
                n898 = property on="Sonuçlar" class="Arr (strict)"() -> ("Value"=w2058:dbl[][])  [unwired: 2 in, 2 out]
                n899 = property on="Sonuçlar" class="Arr (strict)"() -> ("Value"=w2057:dbl[][])  [unwired: 2 in, 2 out]
                n900 = property on="Sonuçlar" class="Arr (strict)"() -> ("Value"=w2054:dbl[][])  [unwired: 2 in, 2 out]
                n901 = Index Array(array=w2061, index (row)=9 ("index"), index (col)=14 ("disabled index (col)")) -> (element=w2060:dbl)
                n902 = Index Array(array=w2058, index (row)=9 ("index"), index (col)=13 ("disabled index (col)")) -> (element=w2059:dbl)
                n903 = Index Array(array=w2057, index (row)=9 ("index"), index (col)=15 ("disabled index (col)")) -> (element=w2056:dbl)
                n904 = Index Array(array=w2054, index (row)=9 ("index"), index (col)=12 ("disabled index (col)")) -> (element=w2055:dbl)
              }
              frame "9000" {
                n905 = property on="Sonuçlar" class="Arr (strict)"() -> ("Value"=w2077:dbl[][])  [unwired: 2 in, 2 out]
                n906 = property on="Sonuçlar" class="Arr (strict)"() -> ("Value"=w2074:dbl[][])  [unwired: 2 in, 2 out]
                n907 = property on="Sonuçlar" class="Arr (strict)"() -> ("Value"=w2073:dbl[][])  [unwired: 2 in, 2 out]
                n908 = property on="Sonuçlar" class="Arr (strict)"() -> ("Value"=w2071:dbl[][])  [unwired: 2 in, 2 out]
                n909 = Index Array(array=w2077, index (row)=10 ("index"), index (col)=14 ("disabled index (col)")) -> (element=w2076:dbl)
                n910 = Index Array(array=w2074, index (row)=10 ("index"), index (col)=13 ("disabled index (col)")) -> (element=w2075:dbl)
                n911 = Index Array(array=w2073, index (row)=10 ("index"), index (col)=15 ("disabled index (col)")) -> (element=w2072:dbl)
                n912 = Index Array(array=w2071, index (row)=10 ("index"), index (col)=12 ("disabled index (col)")) -> (element=w2070:dbl)
              }
              frame "10000" {
                n913 = property on="Sonuçlar" class="Arr (strict)"() -> ("Value"=w2089:dbl[][])  [unwired: 2 in, 2 out]
                n914 = property on="Sonuçlar" class="Arr (strict)"() -> ("Value"=w2091:dbl[][])  [unwired: 2 in, 2 out]
                n915 = property on="Sonuçlar" class="Arr (strict)"() -> ("Value"=w2093:dbl[][])  [unwired: 2 in, 2 out]
                n916 = property on="Sonuçlar" class="Arr (strict)"() -> ("Value"=w2087:dbl[][])  [unwired: 2 in, 2 out]
                n917 = Index Array(array=w2089, index (row)=11 ("index"), index (col)=14 ("disabled index (col)")) -> (element=w2088:dbl)
                n918 = Index Array(array=w2091, index (row)=11 ("index"), index (col)=13 ("disabled index (col)")) -> (element=w2090:dbl)
                n919 = Index Array(array=w2093, index (row)=11 ("index"), index (col)=15 ("disabled index (col)")) -> (element=w2092:dbl)
                n920 = Index Array(array=w2087, index (row)=11 ("index"), index (col)=12 ("disabled index (col)")) -> (element=w2086:dbl)
              }
            }
          }
        }
      }
      frame "Humeral Sap" {
        n921 = case shown="\"Basma Gerilmesi\"" w2111 {
          tunnel: w2110 -> [_ w2120 w2321]
          tunnel: w2109 -> [_ w2117 w2320]
          tunnel: [_ w2115 w2319] -> w2108
          tunnel: w2107 -> [_ w2119 w2318]
          tunnel: [_ w2114 w2317] -> w2106
          tunnel: w2105 -> [_ w2118 w2316]
          tunnel: w2104 -> [_ w2116 w2315]
          tunnel: [_ w2112 w2314] -> w2103
          tunnel: [_ w2113 w2313] -> w2102
          frame "False", Default {
          }
          frame "Burulma Gerilmesi" {
            n922 = case shown="\"10000\"" w2120 {
              tunnel: w2119 -> [_ w2128 w2144 w2160 w2176 w2192 w2208 w2224 w2240 w2256 w2272 w2288 w2304]
              tunnel: w2118 -> [_ w2127 w2143 w2158 w2174 w2185 w2201 w2222 w2238 w2254 w2270 w2286 w2302]
              tunnel: w2117 -> [_ w2126 w2142 w2156 w2172 w2186 w2202 w2220 w2236 w2252 w2268 w2284 w2300]
              tunnel: w2116 -> [_ w2125 w2141 w2154 w2170 w2187 w2203 w2219 w2234 w2250 w2266 w2282 w2298]
              tunnel: [_ w2124 w2137 w2159 w2175 w2191 w2207 w2223 w2239 w2255 w2271 w2287 w2303] -> w2115
              tunnel: [_ w2123 w2138 w2157 w2173 w2190 w2206 w2221 w2237 w2253 w2269 w2285 w2301] -> w2114
              tunnel: [_ w2122 w2139 w2155 w2171 w2189 w2205 w2218 w2235 w2251 w2267 w2283 w2299] -> w2113
              tunnel: [_ w2121 w2140 w2153 w2169 w2188 w2204 w2217 w2233 w2249 w2265 w2281 w2297] -> w2112
              frame "False", Default {
              }
              frame "100" {
                n923 = Index Array(array=w2128, index (row)=12 ("index"), index (col)=18 ("disabled index (col)")) -> (element=w2124:dbl)
                n924 = Index Array(array=w2126, index (row)=12 ("index"), index (col)=17 ("disabled index (col)")) -> (element=w2122:dbl)
                n925 = Index Array(array=w2127, index (row)=12 ("index"), index (col)=19 ("disabled index (col)")) -> (element=w2123:dbl)
                n926 = Index Array(array=w2125, index (row)=12 ("index"), index (col)=16 ("disabled index (col)")) -> (element=w2121:dbl)
              }
              frame "500" {
                n927 = Index Array(array=w2144, index (row)=13 ("index"), index (col)=18 ("disabled index (col)")) -> (element=w2137:dbl)
                n928 = Index Array(array=w2142, index (row)=13 ("index"), index (col)=17 ("disabled index (col)")) -> (element=w2139:dbl)
                n929 = Index Array(array=w2143, index (row)=13 ("index"), index (col)=19 ("disabled index (col)")) -> (element=w2138:dbl)
                n930 = Index Array(array=w2141, index (row)=13 ("index"), index (col)=16 ("disabled index (col)")) -> (element=w2140:dbl)
              }
              frame "1000" {
                n931 = Index Array(array=w2160, index (row)=14 ("index"), index (col)=18 ("disabled index (col)")) -> (element=w2159:dbl)
                n932 = Index Array(array=w2156, index (row)=14 ("index"), index (col)=17 ("disabled index (col)")) -> (element=w2155:dbl)
                n933 = Index Array(array=w2158, index (row)=14 ("index"), index (col)=19 ("disabled index (col)")) -> (element=w2157:dbl)
                n934 = Index Array(array=w2154, index (row)=14 ("index"), index (col)=16 ("disabled index (col)")) -> (element=w2153:dbl)
              }
              frame "2000" {
                n935 = Index Array(array=w2176, index (row)=15 ("index"), index (col)=18 ("disabled index (col)")) -> (element=w2175:dbl)
                n936 = Index Array(array=w2172, index (row)=15 ("index"), index (col)=17 ("disabled index (col)")) -> (element=w2171:dbl)
                n937 = Index Array(array=w2174, index (row)=15 ("index"), index (col)=19 ("disabled index (col)")) -> (element=w2173:dbl)
                n938 = Index Array(array=w2170, index (row)=15 ("index"), index (col)=16 ("disabled index (col)")) -> (element=w2169:dbl)
              }
              frame "3000" {
                n939 = Index Array(array=w2192, index (row)=16 ("index"), index (col)=18 ("disabled index (col)")) -> (element=w2191:dbl)
                n940 = Index Array(array=w2186, index (row)=16 ("index"), index (col)=17 ("disabled index (col)")) -> (element=w2189:dbl)
                n941 = Index Array(array=w2185, index (row)=16 ("index"), index (col)=19 ("disabled index (col)")) -> (element=w2190:dbl)
                n942 = Index Array(array=w2187, index (row)=16 ("index"), index (col)=16 ("disabled index (col)")) -> (element=w2188:dbl)
              }
              frame "4000" {
                n943 = Index Array(array=w2208, index (row)=17 ("index"), index (col)=18 ("disabled index (col)")) -> (element=w2207:dbl)
                n944 = Index Array(array=w2202, index (row)=17 ("index"), index (col)=17 ("disabled index (col)")) -> (element=w2205:dbl)
                n945 = Index Array(array=w2201, index (row)=17 ("index"), index (col)=19 ("disabled index (col)")) -> (element=w2206:dbl)
                n946 = Index Array(array=w2203, index (row)=17 ("index"), index (col)=16 ("disabled index (col)")) -> (element=w2204:dbl)
              }
              frame "5000" {
                n947 = Index Array(array=w2224, index (row)=18 ("index"), index (col)=18 ("disabled index (col)")) -> (element=w2223:dbl)
                n948 = Index Array(array=w2220, index (row)=18 ("index"), index (col)=17 ("disabled index (col)")) -> (element=w2218:dbl)
                n949 = Index Array(array=w2222, index (row)=18 ("index"), index (col)=19 ("disabled index (col)")) -> (element=w2221:dbl)
                n950 = Index Array(array=w2219, index (row)=18 ("index"), index (col)=16 ("disabled index (col)")) -> (element=w2217:dbl)
              }
              frame "6000" {
                n951 = Index Array(array=w2240, index (row)=19 ("index"), index (col)=18 ("disabled index (col)")) -> (element=w2239:dbl)
                n952 = Index Array(array=w2236, index (row)=19 ("index"), index (col)=17 ("disabled index (col)")) -> (element=w2235:dbl)
                n953 = Index Array(array=w2238, index (row)=19 ("index"), index (col)=19 ("disabled index (col)")) -> (element=w2237:dbl)
                n954 = Index Array(array=w2234, index (row)=19 ("index"), index (col)=16 ("disabled index (col)")) -> (element=w2233:dbl)
              }
              frame "7000" {
                n955 = Index Array(array=w2256, index (row)=20 ("index"), index (col)=18 ("disabled index (col)")) -> (element=w2255:dbl)
                n956 = Index Array(array=w2252, index (row)=20 ("index"), index (col)=17 ("disabled index (col)")) -> (element=w2251:dbl)
                n957 = Index Array(array=w2254, index (row)=20 ("index"), index (col)=19 ("disabled index (col)")) -> (element=w2253:dbl)
                n958 = Index Array(array=w2250, index (row)=20 ("index"), index (col)=16 ("disabled index (col)")) -> (element=w2249:dbl)
              }
              frame "8000" {
                n959 = Index Array(array=w2272, index (row)=21 ("index"), index (col)=18 ("disabled index (col)")) -> (element=w2271:dbl)
                n960 = Index Array(array=w2268, index (row)=21 ("index"), index (col)=17 ("disabled index (col)")) -> (element=w2267:dbl)
                n961 = Index Array(array=w2270, index (row)=21 ("index"), index (col)=19 ("disabled index (col)")) -> (element=w2269:dbl)
                n962 = Index Array(array=w2266, index (row)=21 ("index"), index (col)=16 ("disabled index (col)")) -> (element=w2265:dbl)
              }
              frame "9000" {
                n963 = Index Array(array=w2288, index (row)=22 ("index"), index (col)=18 ("disabled index (col)")) -> (element=w2287:dbl)
                n964 = Index Array(array=w2284, index (row)=22 ("index"), index (col)=17 ("disabled index (col)")) -> (element=w2283:dbl)
                n965 = Index Array(array=w2286, index (row)=22 ("index"), index (col)=19 ("disabled index (col)")) -> (element=w2285:dbl)
                n966 = Index Array(array=w2282, index (row)=22 ("index"), index (col)=16 ("disabled index (col)")) -> (element=w2281:dbl)
              }
              frame "10000" {
                n967 = Index Array(array=w2304, index (row)=23 ("index"), index (col)=18 ("disabled index (col)")) -> (element=w2303:dbl)
                n968 = Index Array(array=w2300, index (row)=23 ("index"), index (col)=17 ("disabled index (col)")) -> (element=w2299:dbl)
                n969 = Index Array(array=w2302, index (row)=23 ("index"), index (col)=19 ("disabled index (col)")) -> (element=w2301:dbl)
                n970 = Index Array(array=w2298, index (row)=23 ("index"), index (col)=16 ("disabled index (col)")) -> (element=w2297:dbl)
              }
            }
          }
          frame "Basma Gerilmesi" {
            n971 = case shown="\"100\"" w2321 {
              tunnel: w2320 -> [_ w2325 w2343 w2359 w2375 w2389 w2408 w2423 w2439 w2455 w2469 w2487 w2505]
              tunnel: [_ w2328 w2338 w2357 w2373 w2390 w2406 w2418 w2437 w2452 w2472 w2485 w2504] -> w2319
              tunnel: w2318 -> [_ w2329 w2345 w2361 w2377 w2393 w2410 w2425 w2441 w2457 w2473 w2486 w2503]
              tunnel: [_ w2326 w2339 w2356 w2372 w2391 w2405 w2419 w2436 w2453 w2470 w2483 w2502] -> w2317
              tunnel: w2316 -> [_ w2327 w2344 w2360 w2376 w2392 w2409 w2424 w2440 w2456 w2471 w2488 w2501]
              tunnel: w2315 -> [_ w2323 w2342 w2358 w2374 w2388 w2407 w2422 w2438 w2454 w2468 w2489 w2500]
              tunnel: [_ w2322 w2341 w2354 w2370 w2386 w2403 w2421 w2434 w2450 w2466 w2482 w2499] -> w2314
              tunnel: [_ w2324 w2340 w2355 w2371 w2387 w2404 w2420 w2435 w2451 w2467 w2484 w2498] -> w2313
              frame "False", Default {
              }
              frame "100" {
                n972 = Index Array(array=w2329, index (row)=0 ("index"), index (col)=18 ("disabled index (col)")) -> (element=w2328:dbl)
                n973 = Index Array(array=w2325, index (row)=0 ("index"), index (col)=17 ("disabled index (col)")) -> (element=w2324:dbl)
                n974 = Index Array(array=w2327, index (row)=0 ("index"), index (col)=19 ("disabled index (col)")) -> (element=w2326:dbl)
                n975 = Index Array(array=w2323, index (row)=0 ("index"), index (col)=16 ("disabled index (col)")) -> (element=w2322:dbl)
              }
              frame "500" {
                n976 = Index Array(array=w2345, index (row)=1 ("index"), index (col)=18 ("disabled index (col)")) -> (element=w2338:dbl)
                n977 = Index Array(array=w2343, index (row)=1 ("index"), index (col)=17 ("disabled index (col)")) -> (element=w2340:dbl)
                n978 = Index Array(array=w2344, index (row)=1 ("index"), index (col)=19 ("disabled index (col)")) -> (element=w2339:dbl)
                n979 = Index Array(array=w2342, index (row)=1 ("index"), index (col)=16 ("disabled index (col)")) -> (element=w2341:dbl)
              }
              frame "1000" {
                n980 = Index Array(array=w2361, index (row)=2 ("index"), index (col)=18 ("disabled index (col)")) -> (element=w2357:dbl)
                n981 = Index Array(array=w2359, index (row)=2 ("index"), index (col)=17 ("disabled index (col)")) -> (element=w2355:dbl)
                n982 = Index Array(array=w2360, index (row)=2 ("index"), index (col)=19 ("disabled index (col)")) -> (element=w2356:dbl)
                n983 = Index Array(array=w2358, index (row)=2 ("index"), index (col)=16 ("disabled index (col)")) -> (element=w2354:dbl)
              }
              frame "2000" {
                n984 = Index Array(array=w2377, index (row)=3 ("index"), index (col)=18 ("disabled index (col)")) -> (element=w2373:dbl)
                n985 = Index Array(array=w2375, index (row)=3 ("index"), index (col)=17 ("disabled index (col)")) -> (element=w2371:dbl)
                n986 = Index Array(array=w2376, index (row)=3 ("index"), index (col)=19 ("disabled index (col)")) -> (element=w2372:dbl)
                n987 = Index Array(array=w2374, index (row)=3 ("index"), index (col)=16 ("disabled index (col)")) -> (element=w2370:dbl)
              }
              frame "3000" {
                n988 = Index Array(array=w2393, index (row)=4 ("index"), index (col)=18 ("disabled index (col)")) -> (element=w2390:dbl)
                n989 = Index Array(array=w2389, index (row)=4 ("index"), index (col)=17 ("disabled index (col)")) -> (element=w2387:dbl)
                n990 = Index Array(array=w2392, index (row)=4 ("index"), index (col)=19 ("disabled index (col)")) -> (element=w2391:dbl)
                n991 = Index Array(array=w2388, index (row)=4 ("index"), index (col)=16 ("disabled index (col)")) -> (element=w2386:dbl)
              }
              frame "4000" {
                n992 = Index Array(array=w2410, index (row)=5 ("index"), index (col)=18 ("disabled index (col)")) -> (element=w2406:dbl)
                n993 = Index Array(array=w2408, index (row)=5 ("index"), index (col)=17 ("disabled index (col)")) -> (element=w2404:dbl)
                n994 = Index Array(array=w2409, index (row)=5 ("index"), index (col)=19 ("disabled index (col)")) -> (element=w2405:dbl)
                n995 = Index Array(array=w2407, index (row)=5 ("index"), index (col)=16 ("disabled index (col)")) -> (element=w2403:dbl)
              }
              frame "5000" {
                n996 = Index Array(array=w2425, index (row)=6 ("index"), index (col)=18 ("disabled index (col)")) -> (element=w2418:dbl)
                n997 = Index Array(array=w2423, index (row)=6 ("index"), index (col)=17 ("disabled index (col)")) -> (element=w2420:dbl)
                n998 = Index Array(array=w2424, index (row)=6 ("index"), index (col)=19 ("disabled index (col)")) -> (element=w2419:dbl)
                n999 = Index Array(array=w2422, index (row)=6 ("index"), index (col)=16 ("disabled index (col)")) -> (element=w2421:dbl)
              }
              frame "6000" {
                n1000 = Index Array(array=w2441, index (row)=7 ("index"), index (col)=18 ("disabled index (col)")) -> (element=w2437:dbl)
                n1001 = Index Array(array=w2439, index (row)=7 ("index"), index (col)=17 ("disabled index (col)")) -> (element=w2435:dbl)
                n1002 = Index Array(array=w2440, index (row)=7 ("index"), index (col)=19 ("disabled index (col)")) -> (element=w2436:dbl)
                n1003 = Index Array(array=w2438, index (row)=7 ("index"), index (col)=16 ("disabled index (col)")) -> (element=w2434:dbl)
              }
              frame "7000" {
                n1004 = Index Array(array=w2457, index (row)=8 ("index"), index (col)=18 ("disabled index (col)")) -> (element=w2452:dbl)
                n1005 = Index Array(array=w2455, index (row)=8 ("index"), index (col)=17 ("disabled index (col)")) -> (element=w2451:dbl)
                n1006 = Index Array(array=w2456, index (row)=8 ("index"), index (col)=19 ("disabled index (col)")) -> (element=w2453:dbl)
                n1007 = Index Array(array=w2454, index (row)=8 ("index"), index (col)=16 ("disabled index (col)")) -> (element=w2450:dbl)
              }
              frame "8000" {
                n1008 = Index Array(array=w2473, index (row)=9 ("index"), index (col)=18 ("disabled index (col)")) -> (element=w2472:dbl)
                n1009 = Index Array(array=w2469, index (row)=9 ("index"), index (col)=17 ("disabled index (col)")) -> (element=w2467:dbl)
                n1010 = Index Array(array=w2471, index (row)=9 ("index"), index (col)=19 ("disabled index (col)")) -> (element=w2470:dbl)
                n1011 = Index Array(array=w2468, index (row)=9 ("index"), index (col)=16 ("disabled index (col)")) -> (element=w2466:dbl)
              }
              frame "9000" {
                n1012 = Index Array(array=w2486, index (row)=10 ("index"), index (col)=18 ("disabled index (col)")) -> (element=w2485:dbl)
                n1013 = Index Array(array=w2487, index (row)=10 ("index"), index (col)=17 ("disabled index (col)")) -> (element=w2484:dbl)
                n1014 = Index Array(array=w2488, index (row)=10 ("index"), index (col)=19 ("disabled index (col)")) -> (element=w2483:dbl)
                n1015 = Index Array(array=w2489, index (row)=10 ("index"), index (col)=16 ("disabled index (col)")) -> (element=w2482:dbl)
              }
              frame "10000" {
                n1016 = Index Array(array=w2503, index (row)=11 ("index"), index (col)=18 ("disabled index (col)")) -> (element=w2502:dbl)
                n1017 = Index Array(array=w2505, index (row)=11 ("index"), index (col)=17 ("disabled index (col)")) -> (element=w2504:dbl)
                n1018 = Index Array(array=w2501, index (row)=11 ("index"), index (col)=19 ("disabled index (col)")) -> (element=w2498:dbl)
                n1019 = Index Array(array=w2500, index (row)=11 ("index"), index (col)=16 ("disabled index (col)")) -> (element=w2499:dbl)
              }
            }
          }
        }
      }
      frame "Vida 4mm" {
        n1020 = case shown="\"Basma Gerilmesi\"" w2522 {
          tunnel: w2523 -> [_ w2532 w2733]
          tunnel: w2521 -> [_ w2531 w2732]
          tunnel: w2520 -> [_ w2530 w2730]
          tunnel: w2519 -> [_ w2529 w2731]
          tunnel: w2518 -> [_ w2528 w2729]
          tunnel: [_ w2527 w2728] -> w2517
          tunnel: [_ w2526 w2727] -> w2516
          tunnel: [_ w2525 w2726] -> w2515
          tunnel: [_ w2524 w2725] -> w2514
          frame "False", Default {
          }
          frame "Burulma Gerilmesi" {
            n1021 = case shown="\"10000\"" w2532 {
              tunnel: w2531 -> [_ w2540 w2556 w2572 w2588 w2604 w2620 w2636 w2652 w2668 w2684 w2700 w2716]
              tunnel: w2530 -> [_ w2539 w2554 w2569 w2586 w2602 w2616 w2632 w2648 w2664 w2680 w2696 w2712]
              tunnel: w2529 -> [_ w2538 w2555 w2571 w2587 w2603 w2618 w2634 w2650 w2666 w2682 w2698 w2714]
              tunnel: w2528 -> [_ w2537 w2553 w2568 w2585 w2601 w2614 w2630 w2646 w2662 w2678 w2694 w2710]
              tunnel: [_ w2536 w2549 w2565 w2581 w2600 w2619 w2635 w2651 w2667 w2683 w2699 w2715] -> w2527
              tunnel: [_ w2535 w2550 w2570 w2582 w2599 w2617 w2633 w2649 w2665 w2681 w2697 w2713] -> w2526
              tunnel: [_ w2534 w2551 w2566 w2583 w2598 w2615 w2631 w2647 w2663 w2679 w2695 w2711] -> w2525
              tunnel: [_ w2533 w2552 w2567 w2584 w2597 w2613 w2629 w2645 w2661 w2677 w2693 w2709] -> w2524
              frame "False", Default {
              }
              frame "100" {
                n1022 = Index Array(array=w2540, index (row)=12 ("index"), index (col)=22 ("disabled index (col)")) -> (element=w2536:dbl)
                n1023 = Index Array(array=w2538, index (row)=12 ("index"), index (col)=21 ("disabled index (col)")) -> (element=w2534:dbl)
                n1024 = Index Array(array=w2539, index (row)=12 ("index"), index (col)=23 ("disabled index (col)")) -> (element=w2535:dbl)
                n1025 = Index Array(array=w2537, index (row)=12 ("index"), index (col)=20 ("disabled index (col)")) -> (element=w2533:dbl)
              }
              frame "500" {
                n1026 = Index Array(array=w2556, index (row)=13 ("index"), index (col)=22 ("disabled index (col)")) -> (element=w2549:dbl)
                n1027 = Index Array(array=w2555, index (row)=13 ("index"), index (col)=21 ("disabled index (col)")) -> (element=w2550:dbl)
                n1028 = Index Array(array=w2554, index (row)=13 ("index"), index (col)=23 ("disabled index (col)")) -> (element=w2551:dbl)
                n1029 = Index Array(array=w2553, index (row)=13 ("index"), index (col)=20 ("disabled index (col)")) -> (element=w2552:dbl)
              }
              frame "1000" {
                n1030 = Index Array(array=w2572, index (row)=14 ("index"), index (col)=22 ("disabled index (col)")) -> (element=w2565:dbl)
                n1031 = Index Array(array=w2571, index (row)=14 ("index"), index (col)=21 ("disabled index (col)")) -> (element=w2570:dbl)
                n1032 = Index Array(array=w2569, index (row)=14 ("index"), index (col)=23 ("disabled index (col)")) -> (element=w2566:dbl)
                n1033 = Index Array(array=w2568, index (row)=14 ("index"), index (col)=20 ("disabled index (col)")) -> (element=w2567:dbl)
              }
              frame "2000" {
                n1034 = Index Array(array=w2588, index (row)=15 ("index"), index (col)=22 ("disabled index (col)")) -> (element=w2581:dbl)
                n1035 = Index Array(array=w2587, index (row)=15 ("index"), index (col)=21 ("disabled index (col)")) -> (element=w2582:dbl)
                n1036 = Index Array(array=w2586, index (row)=15 ("index"), index (col)=23 ("disabled index (col)")) -> (element=w2583:dbl)
                n1037 = Index Array(array=w2585, index (row)=15 ("index"), index (col)=20 ("disabled index (col)")) -> (element=w2584:dbl)
              }
              frame "3000" {
                n1038 = Index Array(array=w2604, index (row)=16 ("index"), index (col)=22 ("disabled index (col)")) -> (element=w2600:dbl)
                n1039 = Index Array(array=w2603, index (row)=16 ("index"), index (col)=21 ("disabled index (col)")) -> (element=w2599:dbl)
                n1040 = Index Array(array=w2602, index (row)=16 ("index"), index (col)=23 ("disabled index (col)")) -> (element=w2598:dbl)
                n1041 = Index Array(array=w2601, index (row)=16 ("index"), index (col)=20 ("disabled index (col)")) -> (element=w2597:dbl)
              }
              frame "4000" {
                n1042 = Index Array(array=w2620, index (row)=17 ("index"), index (col)=22 ("disabled index (col)")) -> (element=w2619:dbl)
                n1043 = Index Array(array=w2618, index (row)=17 ("index"), index (col)=21 ("disabled index (col)")) -> (element=w2617:dbl)
                n1044 = Index Array(array=w2616, index (row)=17 ("index"), index (col)=23 ("disabled index (col)")) -> (element=w2615:dbl)
                n1045 = Index Array(array=w2614, index (row)=17 ("index"), index (col)=20 ("disabled index (col)")) -> (element=w2613:dbl)
              }
              frame "5000" {
                n1046 = Index Array(array=w2636, index (row)=18 ("index"), index (col)=22 ("disabled index (col)")) -> (element=w2635:dbl)
                n1047 = Index Array(array=w2634, index (row)=18 ("index"), index (col)=21 ("disabled index (col)")) -> (element=w2633:dbl)
                n1048 = Index Array(array=w2632, index (row)=18 ("index"), index (col)=23 ("disabled index (col)")) -> (element=w2631:dbl)
                n1049 = Index Array(array=w2630, index (row)=18 ("index"), index (col)=20 ("disabled index (col)")) -> (element=w2629:dbl)
              }
              frame "6000" {
                n1050 = Index Array(array=w2652, index (row)=19 ("index"), index (col)=22 ("disabled index (col)")) -> (element=w2651:dbl)
                n1051 = Index Array(array=w2650, index (row)=19 ("index"), index (col)=21 ("disabled index (col)")) -> (element=w2649:dbl)
                n1052 = Index Array(array=w2648, index (row)=19 ("index"), index (col)=23 ("disabled index (col)")) -> (element=w2647:dbl)
                n1053 = Index Array(array=w2646, index (row)=19 ("index"), index (col)=20 ("disabled index (col)")) -> (element=w2645:dbl)
              }
              frame "7000" {
                n1054 = Index Array(array=w2668, index (row)=20 ("index"), index (col)=22 ("disabled index (col)")) -> (element=w2667:dbl)
                n1055 = Index Array(array=w2666, index (row)=20 ("index"), index (col)=21 ("disabled index (col)")) -> (element=w2665:dbl)
                n1056 = Index Array(array=w2664, index (row)=20 ("index"), index (col)=23 ("disabled index (col)")) -> (element=w2663:dbl)
                n1057 = Index Array(array=w2662, index (row)=20 ("index"), index (col)=20 ("disabled index (col)")) -> (element=w2661:dbl)
              }
              frame "8000" {
                n1058 = Index Array(array=w2684, index (row)=21 ("index"), index (col)=22 ("disabled index (col)")) -> (element=w2683:dbl)
                n1059 = Index Array(array=w2682, index (row)=21 ("index"), index (col)=21 ("disabled index (col)")) -> (element=w2681:dbl)
                n1060 = Index Array(array=w2680, index (row)=21 ("index"), index (col)=23 ("disabled index (col)")) -> (element=w2679:dbl)
                n1061 = Index Array(array=w2678, index (row)=21 ("index"), index (col)=20 ("disabled index (col)")) -> (element=w2677:dbl)
              }
              frame "9000" {
                n1062 = Index Array(array=w2700, index (row)=22 ("index"), index (col)=22 ("disabled index (col)")) -> (element=w2699:dbl)
                n1063 = Index Array(array=w2698, index (row)=22 ("index"), index (col)=21 ("disabled index (col)")) -> (element=w2697:dbl)
                n1064 = Index Array(array=w2696, index (row)=22 ("index"), index (col)=23 ("disabled index (col)")) -> (element=w2695:dbl)
                n1065 = Index Array(array=w2694, index (row)=22 ("index"), index (col)=20 ("disabled index (col)")) -> (element=w2693:dbl)
              }
              frame "10000" {
                n1066 = Index Array(array=w2716, index (row)=23 ("index"), index (col)=22 ("disabled index (col)")) -> (element=w2715:dbl)
                n1067 = Index Array(array=w2714, index (row)=23 ("index"), index (col)=21 ("disabled index (col)")) -> (element=w2713:dbl)
                n1068 = Index Array(array=w2712, index (row)=23 ("index"), index (col)=23 ("disabled index (col)")) -> (element=w2711:dbl)
                n1069 = Index Array(array=w2710, index (row)=23 ("index"), index (col)=20 ("disabled index (col)")) -> (element=w2709:dbl)
              }
            }
          }
          frame "Basma Gerilmesi" {
            n1070 = case shown="\"10000\"" w2733 {
              tunnel: w2732 -> [_ w2741 w2757 w2773 w2789 w2805 w2821 w2837 w2853 w2869 w2885 w2901 w2917]
              tunnel: w2731 -> [_ w2739 w2755 w2771 w2787 w2804 w2820 w2836 w2852 w2868 w2884 w2900 w2916]
              tunnel: w2730 -> [_ w2737 w2753 w2769 w2785 w2803 w2819 w2835 w2851 w2867 w2883 w2899 w2915]
              tunnel: w2729 -> [_ w2735 w2751 w2767 w2783 w2802 w2818 w2834 w2850 w2866 w2882 w2898 w2914]
              tunnel: [_ w2740 w2756 w2772 w2788 w2801 w2817 w2830 w2849 w2864 w2878 w2894 w2913] -> w2728
              tunnel: [_ w2738 w2754 w2770 w2786 w2800 w2816 w2831 w2848 w2865 w2879 w2895 w2912] -> w2727
              tunnel: [_ w2736 w2752 w2768 w2784 w2799 w2815 w2832 w2847 w2863 w2880 w2896 w2911] -> w2726
              tunnel: [_ w2734 w2750 w2766 w2782 w2798 w2814 w2833 w2846 w2862 w2881 w2897 w2910] -> w2725
              frame "False", Default {
              }
              frame "100" {
                n1071 = Index Array(array=w2741, index (row)=0 ("index"), index (col)=22 ("disabled index (col)")) -> (element=w2740:dbl)
                n1072 = Index Array(array=w2739, index (row)=0 ("index"), index (col)=21 ("disabled index (col)")) -> (element=w2738:dbl)
                n1073 = Index Array(array=w2737, index (row)=0 ("index"), index (col)=23 ("disabled index (col)")) -> (element=w2736:dbl)
                n1074 = Index Array(array=w2735, index (row)=0 ("index"), index (col)=20 ("disabled index (col)")) -> (element=w2734:dbl)
              }
              frame "500" {
                n1075 = Index Array(array=w2757, index (row)=1 ("index"), index (col)=22 ("disabled index (col)")) -> (element=w2756:dbl)
                n1076 = Index Array(array=w2755, index (row)=1 ("index"), index (col)=21 ("disabled index (col)")) -> (element=w2754:dbl)
                n1077 = Index Array(array=w2753, index (row)=1 ("index"), index (col)=23 ("disabled index (col)")) -> (element=w2752:dbl)
                n1078 = Index Array(array=w2751, index (row)=1 ("index"), index (col)=20 ("disabled index (col)")) -> (element=w2750:dbl)
              }
              frame "1000" {
                n1079 = Index Array(array=w2773, index (row)=2 ("index"), index (col)=22 ("disabled index (col)")) -> (element=w2772:dbl)
                n1080 = Index Array(array=w2771, index (row)=2 ("index"), index (col)=21 ("disabled index (col)")) -> (element=w2770:dbl)
                n1081 = Index Array(array=w2769, index (row)=2 ("index"), index (col)=23 ("disabled index (col)")) -> (element=w2768:dbl)
                n1082 = Index Array(array=w2767, index (row)=2 ("index"), index (col)=20 ("disabled index (col)")) -> (element=w2766:dbl)
              }
              frame "2000" {
                n1083 = Index Array(array=w2789, index (row)=3 ("index"), index (col)=22 ("disabled index (col)")) -> (element=w2788:dbl)
                n1084 = Index Array(array=w2787, index (row)=3 ("index"), index (col)=21 ("disabled index (col)")) -> (element=w2786:dbl)
                n1085 = Index Array(array=w2785, index (row)=3 ("index"), index (col)=23 ("disabled index (col)")) -> (element=w2784:dbl)
                n1086 = Index Array(array=w2783, index (row)=3 ("index"), index (col)=20 ("disabled index (col)")) -> (element=w2782:dbl)
              }
              frame "3000" {
                n1087 = Index Array(array=w2805, index (row)=4 ("index"), index (col)=22 ("disabled index (col)")) -> (element=w2801:dbl)
                n1088 = Index Array(array=w2804, index (row)=4 ("index"), index (col)=21 ("disabled index (col)")) -> (element=w2800:dbl)
                n1089 = Index Array(array=w2803, index (row)=4 ("index"), index (col)=23 ("disabled index (col)")) -> (element=w2799:dbl)
                n1090 = Index Array(array=w2802, index (row)=4 ("index"), index (col)=20 ("disabled index (col)")) -> (element=w2798:dbl)
              }
              frame "4000" {
                n1091 = Index Array(array=w2821, index (row)=5 ("index"), index (col)=22 ("disabled index (col)")) -> (element=w2817:dbl)
                n1092 = Index Array(array=w2820, index (row)=5 ("index"), index (col)=21 ("disabled index (col)")) -> (element=w2816:dbl)
                n1093 = Index Array(array=w2819, index (row)=5 ("index"), index (col)=23 ("disabled index (col)")) -> (element=w2815:dbl)
                n1094 = Index Array(array=w2818, index (row)=5 ("index"), index (col)=20 ("disabled index (col)")) -> (element=w2814:dbl)
              }
              frame "5000" {
                n1095 = Index Array(array=w2837, index (row)=6 ("index"), index (col)=22 ("disabled index (col)")) -> (element=w2830:dbl)
                n1096 = Index Array(array=w2836, index (row)=6 ("index"), index (col)=21 ("disabled index (col)")) -> (element=w2831:dbl)
                n1097 = Index Array(array=w2835, index (row)=6 ("index"), index (col)=23 ("disabled index (col)")) -> (element=w2832:dbl)
                n1098 = Index Array(array=w2834, index (row)=6 ("index"), index (col)=20 ("disabled index (col)")) -> (element=w2833:dbl)
              }
              frame "6000" {
                n1099 = Index Array(array=w2853, index (row)=7 ("index"), index (col)=22 ("disabled index (col)")) -> (element=w2849:dbl)
                n1100 = Index Array(array=w2852, index (row)=7 ("index"), index (col)=21 ("disabled index (col)")) -> (element=w2848:dbl)
                n1101 = Index Array(array=w2851, index (row)=7 ("index"), index (col)=23 ("disabled index (col)")) -> (element=w2847:dbl)
                n1102 = Index Array(array=w2850, index (row)=7 ("index"), index (col)=20 ("disabled index (col)")) -> (element=w2846:dbl)
              }
              frame "7000" {
                n1103 = Index Array(array=w2869, index (row)=8 ("index"), index (col)=22 ("disabled index (col)")) -> (element=w2864:dbl)
                n1104 = Index Array(array=w2868, index (row)=8 ("index"), index (col)=21 ("disabled index (col)")) -> (element=w2865:dbl)
                n1105 = Index Array(array=w2867, index (row)=8 ("index"), index (col)=23 ("disabled index (col)")) -> (element=w2863:dbl)
                n1106 = Index Array(array=w2866, index (row)=8 ("index"), index (col)=20 ("disabled index (col)")) -> (element=w2862:dbl)
              }
              frame "8000" {
                n1107 = Index Array(array=w2885, index (row)=9 ("index"), index (col)=22 ("disabled index (col)")) -> (element=w2878:dbl)
                n1108 = Index Array(array=w2884, index (row)=9 ("index"), index (col)=21 ("disabled index (col)")) -> (element=w2879:dbl)
                n1109 = Index Array(array=w2883, index (row)=9 ("index"), index (col)=23 ("disabled index (col)")) -> (element=w2880:dbl)
                n1110 = Index Array(array=w2882, index (row)=9 ("index"), index (col)=20 ("disabled index (col)")) -> (element=w2881:dbl)
              }
              frame "9000" {
                n1111 = Index Array(array=w2901, index (row)=10 ("index"), index (col)=22 ("disabled index (col)")) -> (element=w2894:dbl)
                n1112 = Index Array(array=w2900, index (row)=10 ("index"), index (col)=21 ("disabled index (col)")) -> (element=w2895:dbl)
                n1113 = Index Array(array=w2899, index (row)=10 ("index"), index (col)=23 ("disabled index (col)")) -> (element=w2896:dbl)
                n1114 = Index Array(array=w2898, index (row)=10 ("index"), index (col)=20 ("disabled index (col)")) -> (element=w2897:dbl)
              }
              frame "10000" {
                n1115 = Index Array(array=w2917, index (row)=11 ("index"), index (col)=22 ("disabled index (col)")) -> (element=w2913:dbl)
                n1116 = Index Array(array=w2916, index (row)=11 ("index"), index (col)=21 ("disabled index (col)")) -> (element=w2912:dbl)
                n1117 = Index Array(array=w2915, index (row)=11 ("index"), index (col)=23 ("disabled index (col)")) -> (element=w2911:dbl)
                n1118 = Index Array(array=w2914, index (row)=11 ("index"), index (col)=20 ("disabled index (col)")) -> (element=w2910:dbl)
              }
            }
          }
        }
      }
      frame "Vida 6.5mm" {
        n1119 = case shown="\"Burulma Gerilmesi\"" w2934 {
          tunnel: w2935 -> [_ w2944 w3145]
          tunnel: w2933 -> [_ w2943 w3144]
          tunnel: w2932 -> [_ w2942 w3143]
          tunnel: w2931 -> [_ w2941 w3142]
          tunnel: w2930 -> [_ w2940 w3141]
          tunnel: [_ w2939 w3140] -> w2929
          tunnel: [_ w2938 w3139] -> w2928
          tunnel: [_ w2937 w3138] -> w2927
          tunnel: [_ w2936 w3137] -> w2926
          frame "False", Default {
          }
          frame "Basma Gerilmesi" {
            n1120 = case shown="\"10000\"" w2944 {
              tunnel: w2943 -> [_ w2952 w2968 w2984 w3000 w3016 w3032 w3048 w3064 w3080 w3096 w3112 w3128]
              tunnel: w2942 -> [_ w2951 w2966 w2983 w2999 w3015 w3031 w3047 w3063 w3078 w3095 w3111 w3127]
              tunnel: w2941 -> [_ w2950 w2964 w2982 w2998 w3014 w3028 w3046 w3062 w3076 w3094 w3110 w3126]
              tunnel: w2940 -> [_ w2949 w2962 w2981 w2997 w3013 w3026 w3045 w3061 w3074 w3089 w3109 w3125]
              tunnel: [_ w2948 w2967 w2980 w2996 w3012 w3029 w3041 w3057 w3079 w3093 w3108 w3124] -> w2939
              tunnel: [_ w2947 w2965 w2979 w2995 w3011 w3030 w3042 w3058 w3077 w3092 w3107 w3123] -> w2938
              tunnel: [_ w2946 w2963 w2978 w2994 w3010 w3027 w3043 w3059 w3075 w3091 w3106 w3122] -> w2937
              tunnel: [_ w2945 w2961 w2977 w2993 w3009 w3025 w3044 w3060 w3073 w3090 w3105 w3121] -> w2936
              frame "False", Default {
              }
              frame "100" {
                n1121 = Index Array(array=w2952, index (row)=0 ("index"), index (col)=26 ("disabled index (col)")) -> (element=w2948:dbl)
                n1122 = Index Array(array=w2950, index (row)=0 ("index"), index (col)=25 ("disabled index (col)")) -> (element=w2946:dbl)
                n1123 = Index Array(array=w2951, index (row)=0 ("index"), index (col)=27 ("disabled index (col)")) -> (element=w2947:dbl)
                n1124 = Index Array(array=w2949, index (row)=0 ("index"), index (col)=24 ("disabled index (col)")) -> (element=w2945:dbl)
              }
              frame "500" {
                n1125 = Index Array(array=w2968, index (row)=1 ("index"), index (col)=26 ("disabled index (col)")) -> (element=w2967:dbl)
                n1126 = Index Array(array=w2964, index (row)=1 ("index"), index (col)=25 ("disabled index (col)")) -> (element=w2963:dbl)
                n1127 = Index Array(array=w2966, index (row)=1 ("index"), index (col)=27 ("disabled index (col)")) -> (element=w2965:dbl)
                n1128 = Index Array(array=w2962, index (row)=1 ("index"), index (col)=24 ("disabled index (col)")) -> (element=w2961:dbl)
              }
              frame "1000" {
                n1129 = Index Array(array=w2984, index (row)=2 ("index"), index (col)=26 ("disabled index (col)")) -> (element=w2980:dbl)
                n1130 = Index Array(array=w2982, index (row)=2 ("index"), index (col)=25 ("disabled index (col)")) -> (element=w2978:dbl)
                n1131 = Index Array(array=w2983, index (row)=2 ("index"), index (col)=27 ("disabled index (col)")) -> (element=w2979:dbl)
                n1132 = Index Array(array=w2981, index (row)=2 ("index"), index (col)=24 ("disabled index (col)")) -> (element=w2977:dbl)
              }
              frame "2000" {
                n1133 = Index Array(array=w3000, index (row)=3 ("index"), index (col)=26 ("disabled index (col)")) -> (element=w2996:dbl)
                n1134 = Index Array(array=w2998, index (row)=3 ("index"), index (col)=25 ("disabled index (col)")) -> (element=w2994:dbl)
                n1135 = Index Array(array=w2999, index (row)=3 ("index"), index (col)=27 ("disabled index (col)")) -> (element=w2995:dbl)
                n1136 = Index Array(array=w2997, index (row)=3 ("index"), index (col)=24 ("disabled index (col)")) -> (element=w2993:dbl)
              }
              frame "3000" {
                n1137 = Index Array(array=w3016, index (row)=4 ("index"), index (col)=26 ("disabled index (col)")) -> (element=w3012:dbl)
                n1138 = Index Array(array=w3014, index (row)=4 ("index"), index (col)=25 ("disabled index (col)")) -> (element=w3010:dbl)
                n1139 = Index Array(array=w3015, index (row)=4 ("index"), index (col)=27 ("disabled index (col)")) -> (element=w3011:dbl)
                n1140 = Index Array(array=w3013, index (row)=4 ("index"), index (col)=24 ("disabled index (col)")) -> (element=w3009:dbl)
              }
              frame "4000" {
                n1141 = Index Array(array=w3032, index (row)=5 ("index"), index (col)=26 ("disabled index (col)")) -> (element=w3029:dbl)
                n1142 = Index Array(array=w3028, index (row)=5 ("index"), index (col)=25 ("disabled index (col)")) -> (element=w3027:dbl)
                n1143 = Index Array(array=w3031, index (row)=5 ("index"), index (col)=27 ("disabled index (col)")) -> (element=w3030:dbl)
                n1144 = Index Array(array=w3026, index (row)=5 ("index"), index (col)=24 ("disabled index (col)")) -> (element=w3025:dbl)
              }
              frame "5000" {
                n1145 = Index Array(array=w3048, index (row)=6 ("index"), index (col)=26 ("disabled index (col)")) -> (element=w3041:dbl)
                n1146 = Index Array(array=w3046, index (row)=6 ("index"), index (col)=25 ("disabled index (col)")) -> (element=w3043:dbl)
                n1147 = Index Array(array=w3047, index (row)=6 ("index"), index (col)=27 ("disabled index (col)")) -> (element=w3042:dbl)
                n1148 = Index Array(array=w3045, index (row)=6 ("index"), index (col)=24 ("disabled index (col)")) -> (element=w3044:dbl)
              }
              frame "6000" {
                n1149 = Index Array(array=w3064, index (row)=7 ("index"), index (col)=26 ("disabled index (col)")) -> (element=w3057:dbl)
                n1150 = Index Array(array=w3062, index (row)=7 ("index"), index (col)=25 ("disabled index (col)")) -> (element=w3059:dbl)
                n1151 = Index Array(array=w3063, index (row)=7 ("index"), index (col)=27 ("disabled index (col)")) -> (element=w3058:dbl)
                n1152 = Index Array(array=w3061, index (row)=7 ("index"), index (col)=24 ("disabled index (col)")) -> (element=w3060:dbl)
              }
              frame "7000" {
                n1153 = Index Array(array=w3080, index (row)=8 ("index"), index (col)=26 ("disabled index (col)")) -> (element=w3079:dbl)
                n1154 = Index Array(array=w3076, index (row)=8 ("index"), index (col)=25 ("disabled index (col)")) -> (element=w3075:dbl)
                n1155 = Index Array(array=w3078, index (row)=8 ("index"), index (col)=27 ("disabled index (col)")) -> (element=w3077:dbl)
                n1156 = Index Array(array=w3074, index (row)=8 ("index"), index (col)=24 ("disabled index (col)")) -> (element=w3073:dbl)
              }
              frame "8000" {
                n1157 = Index Array(array=w3096, index (row)=9 ("index"), index (col)=26 ("disabled index (col)")) -> (element=w3093:dbl)
                n1158 = Index Array(array=w3094, index (row)=9 ("index"), index (col)=25 ("disabled index (col)")) -> (element=w3091:dbl)
                n1159 = Index Array(array=w3095, index (row)=9 ("index"), index (col)=27 ("disabled index (col)")) -> (element=w3092:dbl)
                n1160 = Index Array(array=w3089, index (row)=9 ("index"), index (col)=24 ("disabled index (col)")) -> (element=w3090:dbl)
              }
              frame "9000" {
                n1161 = Index Array(array=w3112, index (row)=10 ("index"), index (col)=26 ("disabled index (col)")) -> (element=w3108:dbl)
                n1162 = Index Array(array=w3110, index (row)=10 ("index"), index (col)=25 ("disabled index (col)")) -> (element=w3106:dbl)
                n1163 = Index Array(array=w3111, index (row)=10 ("index"), index (col)=27 ("disabled index (col)")) -> (element=w3107:dbl)
                n1164 = Index Array(array=w3109, index (row)=10 ("index"), index (col)=24 ("disabled index (col)")) -> (element=w3105:dbl)
              }
              frame "10000" {
                n1165 = Index Array(array=w3128, index (row)=11 ("index"), index (col)=26 ("disabled index (col)")) -> (element=w3124:dbl)
                n1166 = Index Array(array=w3126, index (row)=11 ("index"), index (col)=25 ("disabled index (col)")) -> (element=w3122:dbl)
                n1167 = Index Array(array=w3127, index (row)=11 ("index"), index (col)=27 ("disabled index (col)")) -> (element=w3123:dbl)
                n1168 = Index Array(array=w3125, index (row)=11 ("index"), index (col)=24 ("disabled index (col)")) -> (element=w3121:dbl)
              }
            }
          }
          frame "Burulma Gerilmesi" {
            n1169 = case shown="\"10000\"" w3145 {
              tunnel: w3144 -> [_ w3153 w3169 w3185 w3201 w3217 w3233 w3249 w3265 w3281 w3297 w3313 w3329]
              tunnel: w3143 -> [_ w3151 w3167 w3183 w3199 w3215 w3232 w3247 w3263 w3274 w3295 w3311 w3328]
              tunnel: w3142 -> [_ w3149 w3165 w3181 w3197 w3213 w3231 w3245 w3261 w3278 w3293 w3309 w3327]
              tunnel: w3141 -> [_ w3147 w3163 w3179 w3195 w3211 w3230 w3243 w3259 w3276 w3291 w3307 w3326]
              tunnel: [_ w3152 w3168 w3184 w3200 w3216 w3229 w3248 w3264 w3280 w3296 w3312 w3325] -> w3140
              tunnel: [_ w3150 w3166 w3182 w3198 w3214 w3228 w3246 w3262 w3279 w3294 w3310 w3324] -> w3139
              tunnel: [_ w3148 w3164 w3180 w3196 w3212 w3227 w3244 w3260 w3277 w3292 w3308 w3323] -> w3138
              tunnel: [_ w3146 w3162 w3178 w3194 w3210 w3226 w3242 w3258 w3275 w3290 w3306 w3322] -> w3137
              frame "False", Default {
              }
              frame "100" {
                n1170 = Index Array(array=w3153, index (row)=12 ("index"), index (col)=26 ("disabled index (col)")) -> (element=w3152:dbl)
                n1171 = Index Array(array=w3149, index (row)=12 ("index"), index (col)=25 ("disabled index (col)")) -> (element=w3148:dbl)
                n1172 = Index Array(array=w3151, index (row)=12 ("index"), index (col)=27 ("disabled index (col)")) -> (element=w3150:dbl)
                n1173 = Index Array(array=w3147, index (row)=12 ("index"), index (col)=24 ("disabled index (col)")) -> (element=w3146:dbl)
              }
              frame "500" {
                n1174 = Index Array(array=w3169, index (row)=13 ("index"), index (col)=26 ("disabled index (col)")) -> (element=w3168:dbl)
                n1175 = Index Array(array=w3165, index (row)=13 ("index"), index (col)=25 ("disabled index (col)")) -> (element=w3164:dbl)
                n1176 = Index Array(array=w3167, index (row)=13 ("index"), index (col)=27 ("disabled index (col)")) -> (element=w3166:dbl)
                n1177 = Index Array(array=w3163, index (row)=13 ("index"), index (col)=24 ("disabled index (col)")) -> (element=w3162:dbl)
              }
              frame "1000" {
                n1178 = Index Array(array=w3185, index (row)=14 ("index"), index (col)=26 ("disabled index (col)")) -> (element=w3184:dbl)
                n1179 = Index Array(array=w3181, index (row)=14 ("index"), index (col)=25 ("disabled index (col)")) -> (element=w3180:dbl)
                n1180 = Index Array(array=w3183, index (row)=14 ("index"), index (col)=27 ("disabled index (col)")) -> (element=w3182:dbl)
                n1181 = Index Array(array=w3179, index (row)=14 ("index"), index (col)=24 ("disabled index (col)")) -> (element=w3178:dbl)
              }
              frame "2000" {
                n1182 = Index Array(array=w3201, index (row)=15 ("index"), index (col)=26 ("disabled index (col)")) -> (element=w3200:dbl)
                n1183 = Index Array(array=w3197, index (row)=15 ("index"), index (col)=25 ("disabled index (col)")) -> (element=w3196:dbl)
                n1184 = Index Array(array=w3199, index (row)=15 ("index"), index (col)=27 ("disabled index (col)")) -> (element=w3198:dbl)
                n1185 = Index Array(array=w3195, index (row)=15 ("index"), index (col)=24 ("disabled index (col)")) -> (element=w3194:dbl)
              }
              frame "3000" {
                n1186 = Index Array(array=w3217, index (row)=16 ("index"), index (col)=26 ("disabled index (col)")) -> (element=w3216:dbl)
                n1187 = Index Array(array=w3213, index (row)=16 ("index"), index (col)=25 ("disabled index (col)")) -> (element=w3212:dbl)
                n1188 = Index Array(array=w3215, index (row)=16 ("index"), index (col)=27 ("disabled index (col)")) -> (element=w3214:dbl)
                n1189 = Index Array(array=w3211, index (row)=16 ("index"), index (col)=24 ("disabled index (col)")) -> (element=w3210:dbl)
              }
              frame "4000" {
                n1190 = Index Array(array=w3233, index (row)=17 ("index"), index (col)=26 ("disabled index (col)")) -> (element=w3229:dbl)
                n1191 = Index Array(array=w3231, index (row)=17 ("index"), index (col)=25 ("disabled index (col)")) -> (element=w3227:dbl)
                n1192 = Index Array(array=w3232, index (row)=17 ("index"), index (col)=27 ("disabled index (col)")) -> (element=w3228:dbl)
                n1193 = Index Array(array=w3230, index (row)=17 ("index"), index (col)=24 ("disabled index (col)")) -> (element=w3226:dbl)
              }
              frame "5000" {
                n1194 = Index Array(array=w3249, index (row)=18 ("index"), index (col)=26 ("disabled index (col)")) -> (element=w3248:dbl)
                n1195 = Index Array(array=w3245, index (row)=18 ("index"), index (col)=25 ("disabled index (col)")) -> (element=w3244:dbl)
                n1196 = Index Array(array=w3247, index (row)=18 ("index"), index (col)=27 ("disabled index (col)")) -> (element=w3246:dbl)
                n1197 = Index Array(array=w3243, index (row)=18 ("index"), index (col)=24 ("disabled index (col)")) -> (element=w3242:dbl)
              }
              frame "6000" {
                n1198 = Index Array(array=w3265, index (row)=19 ("index"), index (col)=26 ("disabled index (col)")) -> (element=w3264:dbl)
                n1199 = Index Array(array=w3261, index (row)=19 ("index"), index (col)=25 ("disabled index (col)")) -> (element=w3260:dbl)
                n1200 = Index Array(array=w3263, index (row)=19 ("index"), index (col)=27 ("disabled index (col)")) -> (element=w3262:dbl)
                n1201 = Index Array(array=w3259, index (row)=19 ("index"), index (col)=24 ("disabled index (col)")) -> (element=w3258:dbl)
              }
              frame "7000" {
                n1202 = Index Array(array=w3281, index (row)=20 ("index"), index (col)=26 ("disabled index (col)")) -> (element=w3280:dbl)
                n1203 = Index Array(array=w3278, index (row)=20 ("index"), index (col)=25 ("disabled index (col)")) -> (element=w3277:dbl)
                n1204 = Index Array(array=w3274, index (row)=20 ("index"), index (col)=27 ("disabled index (col)")) -> (element=w3279:dbl)
                n1205 = Index Array(array=w3276, index (row)=20 ("index"), index (col)=24 ("disabled index (col)")) -> (element=w3275:dbl)
              }
              frame "8000" {
                n1206 = Index Array(array=w3297, index (row)=21 ("index"), index (col)=26 ("disabled index (col)")) -> (element=w3296:dbl)
                n1207 = Index Array(array=w3293, index (row)=21 ("index"), index (col)=25 ("disabled index (col)")) -> (element=w3292:dbl)
                n1208 = Index Array(array=w3295, index (row)=21 ("index"), index (col)=27 ("disabled index (col)")) -> (element=w3294:dbl)
                n1209 = Index Array(array=w3291, index (row)=21 ("index"), index (col)=24 ("disabled index (col)")) -> (element=w3290:dbl)
              }
              frame "9000" {
                n1210 = Index Array(array=w3313, index (row)=22 ("index"), index (col)=26 ("disabled index (col)")) -> (element=w3312:dbl)
                n1211 = Index Array(array=w3309, index (row)=22 ("index"), index (col)=25 ("disabled index (col)")) -> (element=w3308:dbl)
                n1212 = Index Array(array=w3311, index (row)=22 ("index"), index (col)=27 ("disabled index (col)")) -> (element=w3310:dbl)
                n1213 = Index Array(array=w3307, index (row)=22 ("index"), index (col)=24 ("disabled index (col)")) -> (element=w3306:dbl)
              }
              frame "10000" {
                n1214 = Index Array(array=w3329, index (row)=23 ("index"), index (col)=26 ("disabled index (col)")) -> (element=w3325:dbl)
                n1215 = Index Array(array=w3327, index (row)=23 ("index"), index (col)=25 ("disabled index (col)")) -> (element=w3323:dbl)
                n1216 = Index Array(array=w3328, index (row)=23 ("index"), index (col)=27 ("disabled index (col)")) -> (element=w3324:dbl)
                n1217 = Index Array(array=w3326, index (row)=23 ("index"), index (col)=24 ("disabled index (col)")) -> (element=w3322:dbl)
              }
            }
          }
        }
      }
    }
    "Min. VonMises Gerilmesi (MPA)" <- w498
    "Max.VonMises Gerilmesi(MPA)" <- w497
    "Max. Yer Değiştirme(mm)" <- w496
    "Min. Yer Değiştirme(mm)" <- w495
  }
  n1218 = while {
    stop <- "Çıkış" stop-if-true
    n1219 = case shown="True" "Oku" {
      tunnel: "Analiz Yapmak İstedeğiniz Parçanın Veri Dosyasını Açınız!" -> [_ w3343]
      frame False {
      }
      frame True {
        n1220 = call-poly <vilib>:"Read Delimited Spreadsheet.vi"("file path (dialog if empty)"=w3343, "format (%.3f)"="%s" ("format (%s)")) -> ("all rows"=→"Sonuçlar":dbl[][])  [unwired: 8 in, 5 out]
      }
    }
  }
